vi "Multichannel Lockin--Develop.vi"() -> ()   [LabVIEW 2019, in "Instrument.Lockin.lvclass"]
uses:
  Instrument.Lockin/Instrument.Lockin.lvclass
  <vilib>/JKI/JKI SMO/SMO/Typedefs/SMOState --Enum.ctl
  Instrument.DAQ/Typedefs/Sweep.Channel--Cluster--Array.ctl
  Instrument.DAQ/Typedefs/Sweep.Channel--Cluster.ctl
  Instrument.DAQ/Typedefs/Sweep.Pattern--Enum.ctl
  Instrument.Lockin/Typedefs/Results Type--Enum.ctl
  <vilib>/Utility/error.llb/DialogType.ctl
  Instrument UI.Lockin/Instrument UI.Lockin.lvclass
  <vilib>/measure/NI_MAPro.lvlib
  <vilib>/Waveform/WDTOps.llb/WDT Waveform to XY Pairs DBL.vi
  <vilib>/Utility/config.llb/NI_LVConfig.lvlib
  <vilib>/JKI/JKI SMO/SMO/SMO.lvclass
  <userlib>/LevyLab/Instrument Framework/SMOs/RemoteControl/RemoteControl.lvclass
  <userlib>/LevyLab/Instrument Framework/SMOs/RemoteControl/Typedefs/Message--Cluster.ctl
  <userlib>/LevyLab/Instrument Framework/SMOs/RemoteControl/Typedefs/PrivateEvents--RemoteControl.Configure.ctl
  <userlib>/LevyLab/Instrument Framework/SMOs/Instrument/Instrument.lvclass
  Instrument.DAQ/Instrument.DAQ.lvclass
  <userlib>/LevyLab/Lockin-Multichannel/Lockin.DAQ/Typedefs/Set State-enum.ctl
  <vilib>/JKI/JKI SMO/SMO/Typedefs/Reserve State--Enum.ctl
  <vilib>/JKI/JKI SMO/SMO/Typedefs/Public Events.ctl
  <userlib>/LevyLab/Lockin-Multichannel/Lockin.DAQ/Typedefs/446xAO-enum.ctl
  <userlib>/LevyLab/Lockin-Multichannel/Lockin.DAQ/Typedefs/446xAI-enum.ctl
  Instrument.DAQ/Typedefs/DAQ.Config.AI.Coupling--enum.ctl
  Instrument.Lockin/Typedefs/Offset Mode--Enum.ctl
  Instrument.Lockin/Typedefs/API/Lockin.setAO_Amp--cluster.ctl
  Instrument.Lockin/Typedefs/API/Lockin.setAO_DC--cluster.ctl
  Instrument.Lockin/Typedefs/API/Lockin.setAO_f--cluster.ctl
  Instrument.Lockin/Typedefs/API/Lockin.setAO_phi--cluster.ctl
  Instrument.Lockin/Typedefs/API/Lockin.setAO_function--cluster.ctl
  Instrument.Lockin/Typedefs/API/Lockin.setAUX--cluster.ctl
  Instrument.Lockin/Typedefs/API/Lockin.setREF_f--cluster.ctl
  Instrument.Lockin/Typedefs/API/Lockin.setREF_phi--cluster.ctl
  Instrument.Lockin/Typedefs/REF Parameter--Enum.ctl
  Instrument.Lockin/Typedefs/API/Lockin.setREF_RollOff--cluster.ctl
  Instrument.Lockin/Typedefs/API/Lockin.setREF_TC--cluster.ctl
  db8adddc-ea00-4bba-81e3-073856fab83d.vi
  b40249d6-2344-4325-9322-c62ca3c32e30.vi
  4ac90d73-6816-45e1-9a9a-5cf5a9c18b14.vi
  7c039171-ebc7-488c-b96c-d45d5d49dc9d.vi
  615c5a2f-0bbc-45ac-9186-a3a982afc109.vi
  be3ecfbe-d453-46a9-a75a-8e102851b763.vi
  23a6cf49-6d38-4771-9ca1-822e649f0410.vi
  1f83e66f-7f6f-456b-9483-784a7ec7341a.vi
  8ae36af7-599d-4610-9c2c-7851f0fb9f0d.vi
  988d757e-36db-49af-af4d-8efcd29764ac.vi
  0dfb07b1-2a32-4a42-a1b7-b992f3b48bb1.vi
  90cbbb8a-83a7-4fa9-8dc2-325b52b36250.vi
  14a45371-8849-4e3a-b935-04e113710313.vi
  9e70ac36-a5eb-4546-996f-d1975d74bcd7.vi
  c2f37f8d-0579-483e-97a6-2ed33b24ebbd.vi
  aed423ae-cdb5-42aa-bd8f-e22cfa73b434.vi
  f9e94923-d644-4e5e-a3f3-1c5941609ee7.vi
  38ece5aa-da02-4231-8862-a988c08df37c.vi
  2d311ae9-1292-4ca0-8339-5bd3e0a854c1.vi
  37d717e0-1655-46e4-bb9c-9d30b95463df.vi
  3940afdf-3a76-4cdf-9013-99d5ad11d00a.vi
  5a0835ea-af00-4b0c-b4aa-accca3fcb3e4.vi
  95e32a6d-11f2-4e85-a49f-a0a7f7e69c5a.vi
  e3f2fa16-99b1-472f-9532-9ae1f83afe4f.vi
  <userlib>/LevyLab/Instrument Framework/SMOs/Logger.Error/Logger.Error.lvclass
  <vilib>/Utility/sysdir.llb/System Directory Type.ctl
  C:/Program Files (x86)/National Instruments/LabVIEW 2019/vi.lib/JKI/JKI SMO/SMO/SMO.lvclass
  Instrument.DAQ/Typedefs/AO.Channel.Function--Enum.ctl
  Instrument.DAQ/Typedefs/Sweep.Configuration--Cluster.ctl
  C:/Program Files (x86)/National Instruments/LabVIEW 2019/user.lib/LevyLab/Instrument Framework/SMOs/Instrument/Instrument.lvclass
  <userlib>/_OpenG.lib/error/error.llb/Filter Error Codes (Array)__ogtk.vi
  <vilib>/Waveform/WDTOps.llb/WDT Waveform Duration DBL.vi
  <vilib>/Platform/browser.llb/Open URL in Default Browser (string).vi
  <vilib>/measure/maspectr.llb/FFT Power Spectrum and PSD for N Chan.vi
panel:
  out "Results Plot Names":string[](array[string])
  out "Version":string="vDevelopment" caption="V"
  in  "Tab Control 4":T1(tab)
  in  "Disable all AI Ref":bool
  in  "Enable only AI Ref1":bool
  in  "Reset Phase":bool
  in  "AI Channels":T2(array[cluster]) {"References" items=["", "1"]}
  in  "AO freq link":dbl=13.0 format="%.3p"
  in  "AO Amp Limit":dbl=0.009999999 format="%.3p"
  in  "Limit Amplitudes":bool
  in  "Link Frequencies":bool
  in  "LP f (Hz)":dbl=100.0 format="%.3p"
  in  "Line":bool
  in  "Lowpass":bool
  in  "AO Channels":T3(array[cluster]) {"Phase" format="%.3g"; "Frequency" min=0.0001 max=10000.0 format="%.3g"; "Offset" format="%.3p"; "Amplitude" min=0.0 max=10.0 format="%.3p"}
  in  "REF Channels":T4(array[cluster]) {"Roll-Off" min=1; "TC" min=0.0001 format="%#_3p"; "Phase" format="%.3g"; "Frequency" min=0.0001 max=10000.0 format="%.3g"}
  in  "DAQ Config":T5(array[cluster]) {"AI.Coupling" items=["AC"=10045, "DC"=10050, "GND"=10066]}
  in  "auto DAQ":bool
  in  "Max Fs Refresh Rate (Hz)":dbl=10.0 format="%#_13g"
  in  "Sampling Mode":enum16{"Manual", "Auto Fs", "Max Fs"}(ring)
  in  "Sampling":cluster{"Fs":dbl, "#s":i32}={"Fs"=10000.0, "#s"=1000}
  in  "Auto x*F1":dbl=5000.0 format="%#_13g"
  in  "Load Configuration":bool
  in  "Save Configuration":bool
  in  "AI Simulation mode":T6(ring)=enum."AI = noise*AO"
  in  "decimating factor":i32=1
  in  "Remove":bool
  in  "Measure":bool
  in  "Stop Sweep":bool caption="Stop"
  in  "Sweep Time (s)":dbl=20.0 format="%#_1f"
  in  "Start Sweep":bool caption="Start"
  in  "Initial Wait (s)":dbl=1.0
  out "Sweep Timer (s)":dbl caption="Timer (s)"
  in  "Return to Start?":bool
  in  "Sweep Channels":T7 {"Channel" items=["AO1"=1, "AO2"=2]; "Start" format="%#_6p"; "End" format="%#_6p"}
  out "Sampling Status":string="Good"
  in  "Output Gain":cluster{"AI.Ch":string, "Gain":dbl}[](array[cluster])=[{"AI.Ch"="AO1", "Gain"=1.0}, {"AI.Ch"="AO2", "Gain"=1.0}, {"AI.Ch"="AO3", "Gain"=1.0}, {"AI.Ch"="AO4", "Gain"=1.0}, {"AI.Ch"="AO5", "Gain"=1.0}, {"AI.Ch"="AO6", "Gain"=1.0}, {"AI.Ch"="AO7", "Gain"=1.0}, {"AI.Ch"="AO8", "Gain"=1.0}, {"AI.Ch"="AO9", "Gain"=1.0}, {"AI.Ch"="AO10", "Gain"=1.0}, {"AI.Ch"="AO11", "Gain"=1.0}, {"AI.Ch"="AO12", "Gain"=1.0}, {"AI.Ch"="AO13", "Gain"=1.0}, {"AI.Ch"="AO14", "Gain"=1.0}, {"AI.Ch"="AO15", "Gain"=1.0}, {"AI.Ch"="AO16", "Gain"=1.0}]
  in  "Input Gain":cluster{"AI.Ch":string, "Gain":dbl}[](array[cluster])=[{"AI.Ch"="AI1", "Gain"=1.0}, {"AI.Ch"="AI2", "Gain"=1.0}, {"AI.Ch"="AI3", "Gain"=1.0}, {"AI.Ch"="AI4", "Gain"=1.0}, {"AI.Ch"="AI5", "Gain"=1.0}, {"AI.Ch"="AI6", "Gain"=1.0}, {"AI.Ch"="AI7", "Gain"=1.0}, {"AI.Ch"="AI8", "Gain"=1.0}, {"AI.Ch"="AI9", "Gain"=1.0}, {"AI.Ch"="AI10", "Gain"=1.0}, {"AI.Ch"="AI11", "Gain"=1.0}, {"AI.Ch"="AI12", "Gain"=1.0}, {"AI.Ch"="AI13", "Gain"=1.0}, {"AI.Ch"="AI14", "Gain"=1.0}, {"AI.Ch"="AI15", "Gain"=1.0}, {"AI.Ch"="AI16", "Gain"=1.0}]
  out "State History":string=" Exit\r Data: Cleanup\r Events: Unregister\r UI: Cleanup\r UI: Disable Buttons\r Configuration: Write\r Error Logger: Destroy\r Lockin SMO: Stop\r Remote SMO: Stop\r Macro: Exit\r UI: Update Sweep Timer\r UI: Update Lockin Graphs\r UI: Update Waveform Graphs\r 4461: OUT\r UI: Update Sweep Timer\r UI: Update Lockin Graphs\r UI: Update Waveform Graphs\r 4461: OUT\r UI: Update Sweep Timer\r UI: Update Lockin Graphs\r UI: Update Waveform Graphs\r 4461: OUT"
  out "Refresh time (ms)":u32=103
  out "LockinDAQ SMO State":T10=enum."Stopped" caption="SMO State"
  out "RC SMO State":T10=enum."Stopped" caption="SMO State"
  in  "Update":bool
  in  "Enable Output":bool caption="Enable"
  in  "Output Channel":i32=1 min=1
  out "Output (V)":dbl
  in  "Aux Channel":tag="Dev2/ao0"
  in  "Voltage Output (V)":dbl min=-50.0 max=50.0
  in  "Amplifier Gain":dbl=1.0 min=-15.0 max=15.0
  out "DAQ Output (V)":dbl=-0.0 min=-3.5 max=3.5
  out "Amplified Output (V)":dbl=-0.0 min=-3.5 max=3.5
  in  "AI Channel":i32=1
  in  "Reference Channel":i32=1
  in  "Type":T11
  in  "Allowed remote system":string
  in  "Get Calibration":bool
  out "Cal Info":T12(array[cluster]) {"SelfCal.LastDate/Time" format="%<%I:%M %p\n%m/%d/%Y>T"}
  in  "Self Calibrate":bool
  in  "Save":bool
  in  "Path":path=path "C:/Data/lockin"
  in  "Notes":string
  in  "Tab Control 3":enum32{"Page 1"}(tab)
  out "X":dbl=0.0014996100939563214 caption="X (V)" format="%#_3p"
  out "Y":dbl=-29.79492153733761 caption="Y (V)" format="%#_3p"
  in  "Channel":i32(ring)=1 items=["AI1 Ref1", "AI2 Ref1", "AI3 Ref1", "AI4 Ref1", "AI5 Ref1", "AI6 Ref1", "AI7 Ref1", "AI8 Ref1"]
  out "R":dbl=0.0014996100939563214 caption="R (V)" format="%#_3p"
  out "Theta":dbl=-29.79492153733761 caption="Theta (°)" format="%#_3p"
  in  "Display":enum16{"X and Y", "R and Theta", "Mean"}(ring)=enum."R and Theta" caption="Enum"
  in  "Close":bool
  out "Status":string="Shutdown"
  in  "Pause":bool
  in  "Reset":bool
  in  "Start":bool
  in  "Help":bool
  in  "Trigger":bool
  in  "Tab Control 2":T13(tab)
  in  "AI Graph All":bool
  in  "AI Graph None":bool
  in  "Y Axis (Output)":enum16{"Analog Output", "Reference"}(ring) caption="Enum 3"
  in  "Y Axis (Input)":enum16{"Device", "ADC"}(ring) caption="Enum 3"
  in  "Decimate":enum16{"1", "10", "100", "1000"}(ring) caption="Enum 3"
  in  "X Axis":enum16{"Time", "Samples"}(ring) caption="Enum 3"
  out "AI Graph":waveform(dbl)[](graph)
  out "AO Graph":waveform(dbl)[](graph)
  in  "AO Graph All":bool
  in  "AO Graph None":bool
  in  "Y/Theta Range":dbl caption="Axis Range" format="%#_6p"
  in  "X/R Range":dbl caption="Axis Range" format="%#_6p"
  out "Lockin 2":waveform(dbl)[](graph) caption="Lockin Display 2"
  out "Lockin 1":waveform(dbl)[](graph)
  in  "Lockin 1 None":bool
  in  "Lockin 1 All":bool
  out "Results":string[][](table)
  out "XY Graph":cluster{"Wavenumber":dbl[], "Data":dbl[]}[](graph)
  in  "XY Axis Range":dbl caption="Axis Range" format="%#_6p"
  out "Sweep Results Y":waveform(dbl)[](graph)
  out "Sweep Results X":waveform(dbl)[](graph)
  out "Sweep Results AI":waveform(dbl)[](graph)
  out "Sweep Results AO":waveform(dbl)[](graph)
  in  "# averages":u32=10 min=1
  in  "weighting mode":enum16{"Linear", "Exponential"}(ring)=enum."Exponential"
  in  "averaging mode":T14(ring)=enum."RMS averaging"
  in  "window":u16(ring) items=["Rectangle", "Hanning"]
  in  "export mode":u16(ring)=1 items=["Power Spectrum", "Power Spectral Density"]
  in  "restart":bool
  out "done?":bool=TRUE
  out "PS Chart":dbl[][](graph)
  out "PS WFGraph":cluster{"f0":dbl, "df":dbl, "magnitude":dbl[]}[](graph)
  out "averages":dbl=180.0
  # "Output"
  # "Input"
  # ">> DEVICE >>"
  # "Amp (V)"
  # "(*)"
  # "Ch"
  # "DC (V)"
  # "f (Hz)"
  # "Phase (°)"
  # "Function"
  # "Sweep"
  # "(*)"
  # "Ch"
  # "Ref1   2     3    4"
  # "Input: Pre-Filter"
  # "Output Settings"
  # "Reference"
  # "Reference Settings"
  # "Ch"
  # "f (Hz)"
  # "Phase (°)"
  # "TC (s)"
  # "Order"
  # "DAQ Channels"
  # "AI"
  # "Device"
  # "AO"
  # "Input: Offset"
  # "Ch"
  # "Range"
  # "Ch"
  # "Range"
  # "Coupling"
  # "Other Configuration"
  # "Sampling"
  # "Changing settings in this box will automatically\nreset the lockin and restart acquisition"
  # "Sweep"
  # "Channel"
  # "Start"
  # "End"
  # "Pattern"
  # "Status"
  # "Channel"
  # "Channel"
  # "Input Gain"
  # "Output Gain"
  # "Auxiliary Output"
  # "Configuration"
  # "- Use to control an auxiliiary card such as a multifunction DAQ (6115, 6120, etc)"
  # "Forward Lockin Input --> Lockin Output"
  # "- Choose an input lockin channel and value (X,Y, etc) and it will be written as a DC value to an output channel of your choosing.\n- Output is scaled by the input amplifier gain."
  # "Calibration"
  # "Self Cal\nLast Time"
  # "Self Cal\nLast Temp"
  # "Temp\nNow"
  # "Cal\nDue"
  # "Device"
  # "AI Graph"
  # "AO/Reference Graph"
  # "Lockin Results 1"
  # "Lockin Results 2"
  # "Lockin Results 2"
  # "Sweep Results"
  # "Sweep AO/AI"
  # "Power Spectra"
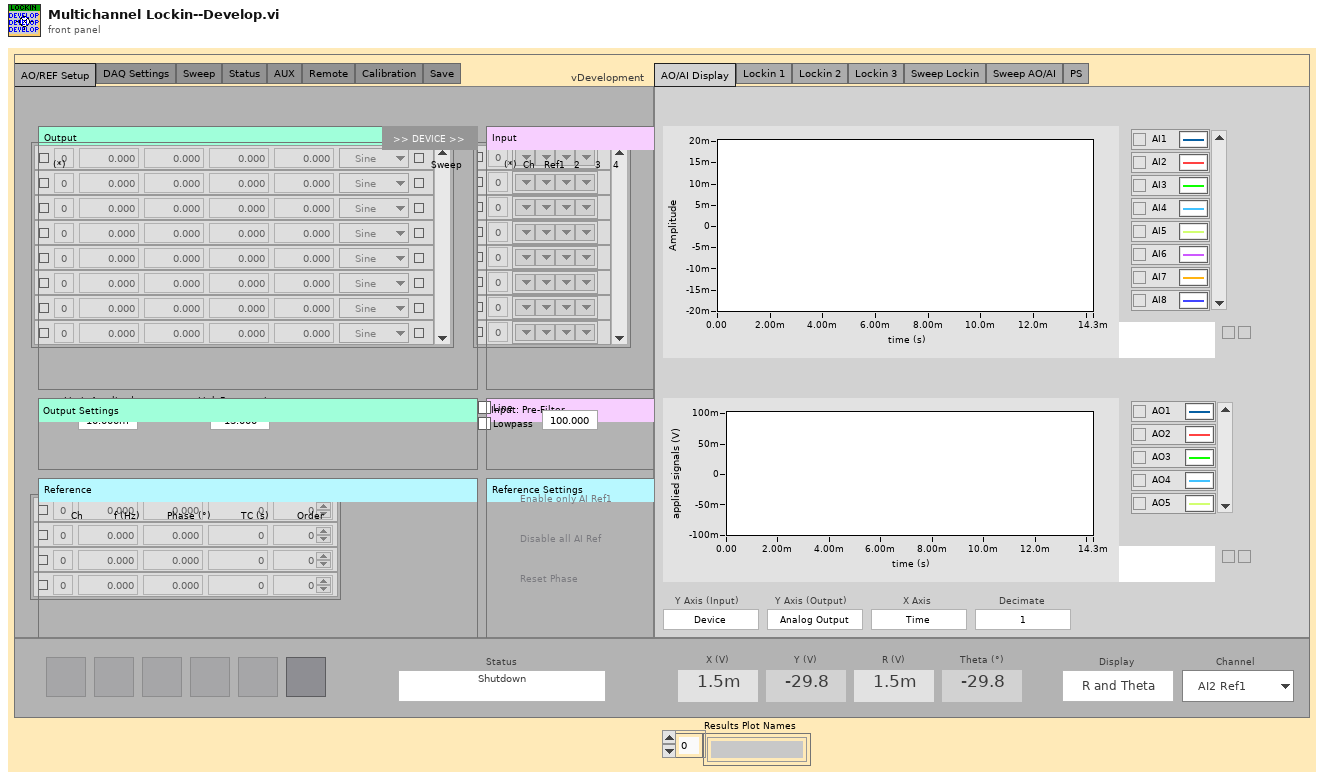
[diagram p1: front panel]
types:
  T1 = enum32{"AO/REF Setup", "DAQ Settings", "Sweep", "Status", "AUX", "Remote", "Calibration", "Save"}
  T2 = cluster{"Enable?":bool, "Channel":i32, "References":u16[]}[]
  T3 = cluster{"Enable?":bool, "Channel":i32, "Amplitude":dbl, "Offset":dbl, "Frequency":dbl, "Phase":dbl, "Function":enum16{"Sine", "Triangle", "Square"}, "Sweeping?":bool}[]
  T4 = cluster{"Enable?":bool, "Channel":i32, "Frequency":dbl, "Phase":dbl, "TC":dbl, "Roll-Off":i32}[]
  T5 = cluster{"Device":string, "AO.Ch":string, "AO.Range":enum16{"±0.1", "±1.0", "±10.0"}, "AI.Ch":string, "AI.Range":enum16{"±0.316", "±1.00", "±3.16", "±10.0", "±31.6", "±42.4"}, "AI.Coupling":u16}[]
  T6 = enum16{"AI = HW simulated", "AI = noise*AO", "AI = waveguide"}
  T7 = typedef "Instrument.DAQ.lvclass/Sweep.Channel--Cluster--Array.ctl" = T8[]
  T8 = typedef "Instrument.DAQ.lvclass/Sweep.Channel--Cluster.ctl" = cluster{"Enable?":bool, "Channel":u16, "Start":dbl, "End":dbl, "Pattern":T9}
  T9 = typedef "Instrument.DAQ.lvclass/Sweep.Pattern--Enum.ctl" = enum16{"Ramp /", "Ramp /\\", "Smooth Ramp _/", "Smooth Ramp _/\\_", "Frequency"}
  T10 = typedef "SMO.lvclass/SMOState --Enum.ctl" = enum16{"unknown", "Created", "Started", "Stopped"}
  T11 = typedef "Instrument.Lockin.lvclass/Results Type--Enum.ctl" = enum16{"X", "Y", "R", "Theta", "Mean"}
  T12 = cluster{"Active Device":string, "SelfCal.LastDate/Time":dbl, "SelfCal.LastTemp":dbl, "DevTemp":dbl, "calibration due?":bool}[]
  T13 = enum32{"AO/AI Display", "Lockin 1", "Lockin 2", "Lockin 3", "Sweep Lockin", "Sweep AO/AI", "PS"}
  T14 = enum16{"No averaging", "Vector averaging", "RMS averaging", "Peak hold"}
  T15 = enum16{"start", "stop", "reset", "start sweep", "stop sweep"}
  T16 = typedef "Lockin.DAQ.lvclass/Set State-enum.ctl" = enum16{"start", "stop", "reset", "start sweep", "stop sweep"}
  T17 = typedef "Instrument.DAQ.lvclass/Sweep.Configuration--Cluster.ctl" = cluster{"Sweep Time (s)":dbl, "Initial Wait (s)":dbl, "Return to Start":bool, "Channels":T7}
  T18 = enum32{"invalid app kind", "Development System", "Run Time System", "Student Edition", "Embedded LabVIEW", "Evaluation", "Custom"}
  T19 = enum32{"Invalid", "Standard", "Closed", "Hidden", "Minimized", "Maximized"}
  T20 = enum8{"Enabled", "Disabled", "Disabled and Grayed Out"}
  T21 = typedef "Instrument.Lockin.lvclass/Lockin.setAO_Amp--cluster.ctl" = cluster{"AO Channel":i32, "Amplitude (V)":dbl}
  T22 = enum16{"Amplitude", "DC", "Frequency", "Phase", "Function"}
  T23 = typedef "Instrument.Lockin.lvclass/Lockin.setAO_DC--cluster.ctl" = cluster{"AO Channel":i32, "DC (V)":dbl}
  T24 = typedef "Instrument.Lockin.lvclass/Lockin.setAO_f--cluster.ctl" = cluster{"AO Channel":i32, "Frequency (Hz)":dbl}
  T25 = typedef "Instrument.Lockin.lvclass/Lockin.setAO_phi--cluster.ctl" = cluster{"AO Channel":i32, "Phase (°)":dbl}
  T26 = typedef "Instrument.Lockin.lvclass/Lockin.setAO_function--cluster.ctl" = cluster{"AO Channel":i32, "Function":T27}
  T27 = typedef "Instrument.DAQ.lvclass/AO.Channel.Function--Enum.ctl" = enum16{"Sine", "Triangle", "Square"}
  T28 = typedef "Instrument.Lockin.lvclass/REF Parameter--Enum.ctl" = enum16{"Frequency", "Phase", "Time Constant", "RollOff"}
  T29 = typedef "Instrument.Lockin.lvclass/Lockin.setREF_f--cluster.ctl" = cluster{"REF Channel":i32, "Frequency (Hz)":dbl}
  T30 = typedef "Instrument.Lockin.lvclass/Lockin.setREF_phi--cluster.ctl" = cluster{"REF Channel":i32, "Phase (°)":dbl}
  T31 = typedef "Instrument.Lockin.lvclass/Lockin.setREF_TC--cluster.ctl" = cluster{"REF Channel":i32, "TC (s)":dbl}
  T32 = typedef "Instrument.Lockin.lvclass/Lockin.setREF_RollOff--cluster.ctl" = cluster{"REF Channel":i32, "Roll-Off":i32}
  T33 = typedef "Instrument.Lockin.lvclass/Offset Mode--Enum.ctl" = enum16{"Measure", "Remove"}
  T34 = cluster{"averaging mode":enum16{"No averaging", "Vector averaging", "RMS averaging", "Peak hold"}, "weighting mode":enum16{"Linear", "Exponential"}, "number of averages":u32}
  T35 = typedef "Instrument.Lockin.lvclass/Lockin.setAUX--cluster.ctl" = cluster{"AO Channel":i32, "AUX (V)":dbl}
  T36 = typedef "Lockin.DAQ.lvclass/446xAO-enum.ctl" = enum16{"±0.1", "±1.0", "±10.0"}
  T37 = typedef "Lockin.DAQ.lvclass/446xAI-enum.ctl" = enum16{"±0.316", "±1.00", "±3.16", "±10.0", "±31.6", "±42.4"}
  T38 = typedef "Instrument.DAQ.lvclass/DAQ.Config.AI.Coupling--enum.ctl" = u16
  T39 = cluster{"Device":string, "AO.Ch":string, "AO.Range":T36, "AI.Ch":string, "AI.Range":T37, "AI.Coupling":T38}[]
  T40 = typedef "Instrument.DAQ.lvclass/Channel.Gain--Cluster--Array.ctl" = T41[]
  T41 = typedef "Instrument.DAQ.lvclass/Channel.Gain--Cluster.ctl" = cluster{"Channel":string, "Gain":dbl}
  T42 = typedef "RemoteControl.lvclass/PrivateEvents--RemoteControl.Configure.ctl" = cluster{"address":string, "Port":u16, "AllowedRemote":string, "Commands":string[], "timeout":i32}
  T43 = typedef "RemoteControl.lvclass/Message--Cluster.ctl" = cluster{"Command":string, "Data":variant, "ID":string}
  T44 = cluster{"Core":cluster{"Current VI Reference":refnum<vi>, "Close Panel on Exit?":bool}, "to":i32, "Lockin":refnum<class "Instrument.Lockin.lvclass">, "RemoteControl":refnum<class "RemoteControl.lvclass">, "Lockin.DAQ":refnum<class "Instrument.DAQ.lvclass">, "Logger.Error":refnum<class "Logger.Error.lvclass">, "DAQ state":enum16{"idle", "created", "started", "stopped", "sweeping"}, "RemoteControl.Configure":T42, "Message":T43, "HandledMessage":T43, "SweepResults":cluster{"X results":waveform(dbl)[], "Y Results":waveform(dbl)[]}, "SweepWaveforms":cluster{"Sweep_AO":waveform(dbl)[], "Sweep_AI":waveform(dbl)[]}}
  T45 = enum16{"idle", "created", "started", "stopped", "sweeping"}
  T46 = typedef "Instrument.DAQ.lvclass/DAQ.Config.AO--Cluster--Array.ctl" = T47[]
  T47 = typedef "Instrument.DAQ.lvclass/DAQ.Config.AO--Cluster.ctl" = cluster{"Channels":tag, "Range":T48, "output terminal configuration":i32, "Type":T49}
  T48 = typedef "Instrument.DAQ.lvclass/DAQ.Config.AO.Range--enum.ctl" = enum16{"±0.1", "±1.0", "±10.0"}
  T49 = typedef "Instrument.DAQ.lvclass/DAQ.Type--enum.ctl" = enum16{"None", "USB 4431", "PXI 446x"}
  T50 = typedef "Instrument.DAQ.lvclass/DAQ.Config.AI--Cluster--Array.ctl" = T51[]
  T51 = typedef "Instrument.DAQ.lvclass/DAQ.Config.AI--Cluster.ctl" = cluster{"Channels":tag, "Coupling":T38, "Range":T52, "input terminal configuration":i32, "Type":T49}
  T52 = typedef "Instrument.DAQ.lvclass/DAQ.Config.AI.Range--enum.ctl" = enum16{"±0.316", "±1.00", "±3.16", "±10.0", "±31.6", "±42.4"}
  T53 = typedef "Lockin.DAQ.lvclass/Results--Cluster.ctl" = cluster{"Time Stamp":timestamp, "Results (Dictionary)":cluster{"key":string, "value":dbl}[]}
  T54 = typedef "Lockin.DAQ.lvclass/AO-cluster.ctl" = T55[]
  T55 = typedef "Instrument.Lockin.UI.lvclass/AO Channel--Cluster.ctl" = cluster{"Enable?":bool, "Channel":i32, "Amplitude":dbl, "Offset":dbl, "Frequency":dbl, "Phase":dbl, "Function":T56, "Sweeping?":bool}
  T56 = typedef "Lockin.DAQ.lvclass/Function-enum.ctl" = enum16{"Sine", "Triangle", "Square"}
  T57 = typedef "Lockin.DAQ.lvclass/REF-cluster.ctl" = T58[]
  T58 = typedef "Instrument.Lockin.UI.lvclass/REF Channel--Cluster.ctl" = cluster{"Enable?":bool, "Channel":i32, "Frequency":dbl, "Phase":dbl, "TC":dbl, "Roll-Off":i32}
  T59 = typedef "Lockin.DAQ.lvclass/PublicEvents--Lockin.DAQ.getDAQconfig.ctl" = T60[]
  T60 = typedef "Instrument.Lockin.UI.lvclass/Device Configuration--Cluster.ctl" = cluster{"Device":string, "AO.Ch":string, "AO.Range":T36, "AI.Ch":string, "AI.Range":T37, "AI.Coupling":T61}
  T61 = typedef "Lockin.DAQ.lvclass/AI.coupling-enum.ctl" = u16
  T62 = typedef "Lockin.DAQ.lvclass/PublicEvents--Lockin.DAQ.getCalibration.ctl" = T63[]
  T63 = typedef "Lockin.DAQ.lvclass/Cal Info - Cluster.ctl" = cluster{"Active Device":string, "SelfCal.LastDate/Time":dbl, "SelfCal.LastTemp":dbl, "DevTemp":dbl, "calibration due?":bool}
  T64 = typedef "Lockin.DAQ.lvclass/SweepResults--Cluster.ctl" = cluster{"X results":waveform(dbl)[], "Y Results":waveform(dbl)[]}
  T65 = cluster{"X":waveform(dbl)[], "Y":waveform(dbl)[]}
  T66 = typedef "Lockin.DAQ.lvclass/PublicEvents--Lockin.DAQ.getAI.ctl" = waveform(dbl)[]
  T67 = typedef "Lockin.DAQ.lvclass/PublicEvents--Lockin.DAQ.getAO.ctl" = waveform(dbl)[]
  T68 = typedef "Lockin.DAQ.lvclass/State-enum.ctl" = enum16{"idle", "created", "started", "stopped", "sweeping"}
  T69 = typedef "DialogType.ctl" = u16
  T70 = cluster{"Sweep_AO":waveform(dbl)[], "Sweep_AI":waveform(dbl)[]}
  T71 = cluster{"X results":waveform(dbl)[], "Y Results":waveform(dbl)[]}
  T72 = cluster{"Time Stamp":timestamp, "Results (Dictionary)":cluster{"key":string, "value":dbl}[]}
  T73 = cluster{"Current VI Reference":refnum<vi>, "Close Panel on Exit?":bool}
  T74 = typedef "SMO.lvclass/Public Events.ctl" = cluster{"Error":refnum<user-event>, "State":refnum<user-event>, "Reserve State":refnum<user-event>}
  T75 = typedef "RemoteControl.lvclass/PublicEvents--Cluster.ctl" = cluster{"SendMessageFromProcess":refnum<user-event>}
  T76 = typedef "Lockin.DAQ.lvclass/PublicEvents--Cluster.ctl" = cluster{"getAO":refnum<user-event>, "getAI":refnum<user-event>, "getREF":refnum<user-event>, "getResults":refnum<user-event>, "getCalibration":refnum<user-event>, "getAOChannels":refnum<user-event>, "getREFChannels":refnum<user-event>, "getDAQState":refnum<user-event>, "getSweepResults":refnum<user-event>, "getSweepWaveforms":refnum<user-event>, "getDAQconfig":refnum<user-event>}
  T77 = typedef "Instrument.DAQ.lvclass/AI.Channel--Cluster--Array.ctl" = T78[]
  T78 = typedef "Instrument.DAQ.lvclass/AI.Channel--Cluster.ctl" = cluster{"Enable?":bool, "Channel":i32, "References":i32[]}
  T79 = typedef "System Directory Type.ctl" = i32
  T80 = typedef "RemoteControl.lvclass/RC Com Type--enum.ctl" = enum16{"RC", "STM", "ZMQ"}
  T81 = typedef "Instrument.DAQ.lvclass/AO.Channel--Cluster--Array.ctl" = T82[]
  T82 = typedef "Instrument.DAQ.lvclass/AO.Channel--Cluster.ctl" = cluster{"Enable?":bool, "Channel":i32, "Amplitude":dbl, "Offset":dbl, "Frequency":dbl, "Phase":dbl, "Function":T27, "Sweeping?":bool}
  T83 = typedef "Instrument.DAQ.lvclass/REF.Channel--Cluster--Array.ctl" = T84[]
  T84 = typedef "Instrument.DAQ.lvclass/REF.Channel--Cluster.ctl" = cluster{"Enable?":bool, "Channel":i32, "Frequency":dbl, "Phase":dbl, "TC":dbl, "Roll-Off":i32}
  T85 = typedef "Instrument.DAQ.lvclass/Configuration.Prefilter--Cluster.ctl" = cluster{"60 Hz":bool, "Low Pass":bool, "Low Pass Cutoff (Hz)":dbl}
  T86 = typedef "Instrument.Lockin.lvclass/Lockin.Configuration--Cluster.ctl" = cluster{"AO Channels":T54, "REF Channels":T57, "AI Channels":T87, "REF Filter":T89, "Amplifers":cluster{"offsets":dbl[], "Input Gain":dbl[], "Output Gain":dbl[], "Amplifiers":T90}, "DAQ":cluster{"sampling":T91, "sample mode":i32, "buffer size (S)":u32, "decimation":u32}, "Calibration":cluster{"Cal Info":T63[]}, "AI Configuration":T92, "AO Configuration":T95, "Aux Channel":tag, "Simulation mode":T97}
  T87 = typedef "Lockin.DAQ.lvclass/AI-cluster.ctl" = T88[]
  T88 = typedef "Instrument.Lockin.UI.lvclass/AI Channel--Cluster.ctl" = cluster{"Enable?":bool, "Channel":i32, "References":u16[]}
  T89 = typedef "Lockin.DAQ.lvclass/AI Prefilter-cluster.ctl" = cluster{"60 Hz prefilter":bool, "LP prefilter":bool, "LP cutoff (Hz)":dbl}
  T90 = typedef "Lockin.DAQ.lvclass/AmplifierType-enum.ctl" = enum16{"Manual", "Krohn Hite", "Femto"}
  T91 = typedef "Lockin.DAQ.lvclass/Sampling.ctl" = cluster{"Fs":dbl, "#s":i32}
  T92 = typedef "Lockin.DAQ.lvclass/AI.config-array.ctl" = T93[]
  T93 = typedef "Lockin.DAQ.lvclass/AI.config-cluster.ctl" = cluster{"AI.channels":tag, "AI.Coupling":T61, "AI.Range":T37, "input terminal configuration":i32, "DAQ Type":T94}
  T94 = typedef "Lockin.DAQ.lvclass/DAQType-enum.ctl" = enum16{"None", "USB 4431", "PXI 446x"}
  T95 = typedef "Lockin.DAQ.lvclass/AO.config-array.ctl" = T96[]
  T96 = typedef "Lockin.DAQ.lvclass/AO.config-cluster.ctl" = cluster{"AO.channels":tag, "AO.Range":T36, "output terminal configuration":i32, "DAQ Type":T94}
  T97 = typedef "Lockin.DAQ.lvclass/AI Simulation-enum.ctl" = enum16{"AI = HW simulated", "AI = noise*AO", "AI = waveguide"}
  T98 = typedef "Instrument.DAQ.lvclass/DAQ.Configuration--Cluster.ctl" = cluster{"Device":string, "AO.Ch":string, "AO.Range":T48, "AI.Ch":string, "AI.Range":T52, "AI.Coupling":T38}
  T99 = typedef "Instrument.DAQ.lvclass/DAQ.Sampling--Cluster.ctl" = cluster{"Sampling":T100, "Sample Mode":T101, "Fs Mode":T102, "Fs Multiplier":dbl, "Refresh Rate (Hz)":dbl, "Decimation":i32}
  T100 = typedef "Instrument.DAQ.lvclass/DAQ.Sampling.Sampling--Cluster.ctl" = cluster{"Fs":dbl, "#s":i32}
  T101 = typedef "Instrument.DAQ.lvclass/DAQ.Sampling.Sample Mode--Ring.ctl" = i32
  T102 = typedef "Instrument.DAQ.lvclass/DAQ.Sampling.Fs Mode--enum.ctl" = enum16{"Manual", "Auto Fs", "Max Fs"}
  T103 = cluster{"Sweep Time (s)":dbl, "Initial Wait (s)":dbl, "Return to Start":bool, "Channels":T8[]}
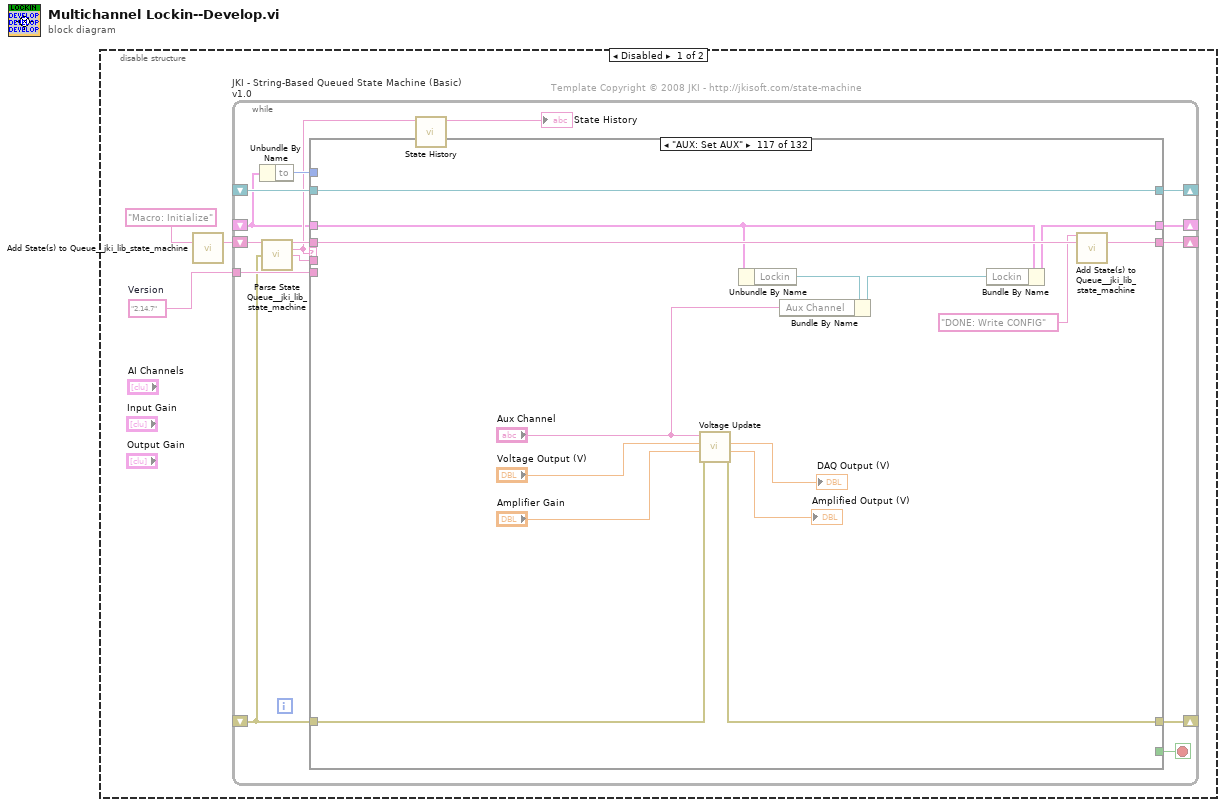
[diagram p0: block diagram]
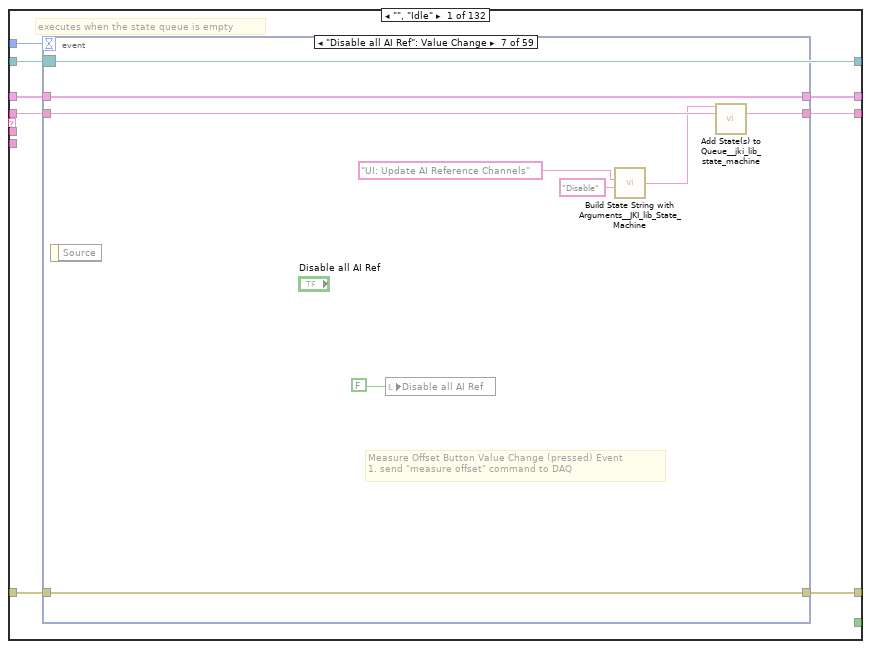
[diagram p2: hidden frame]
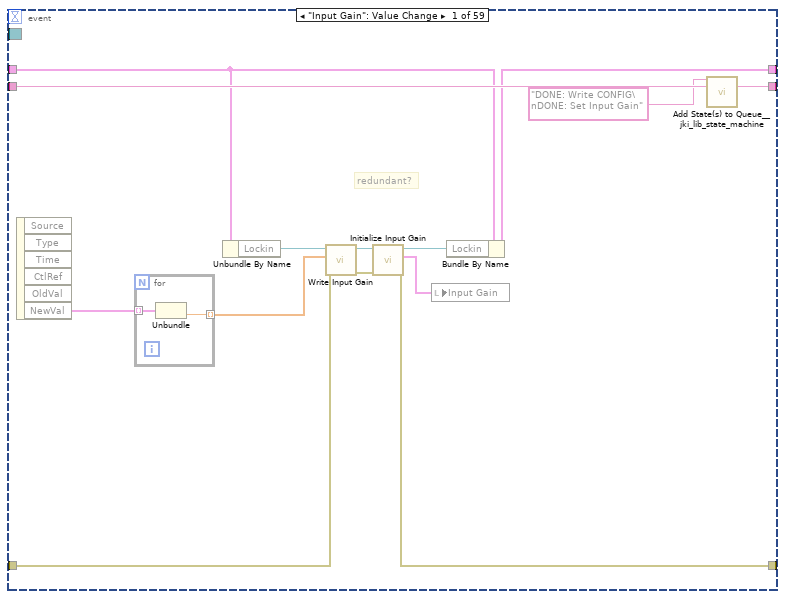
[diagram p3: hidden frame]
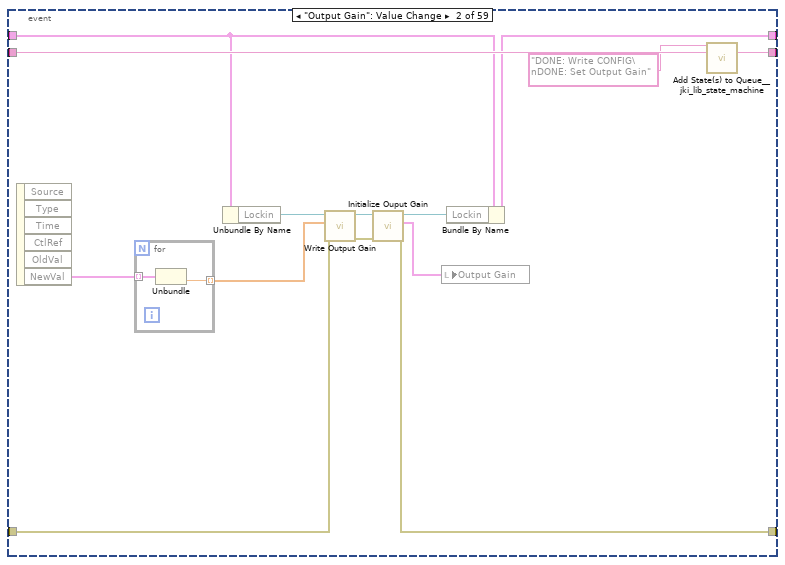
[diagram p4: hidden frame]
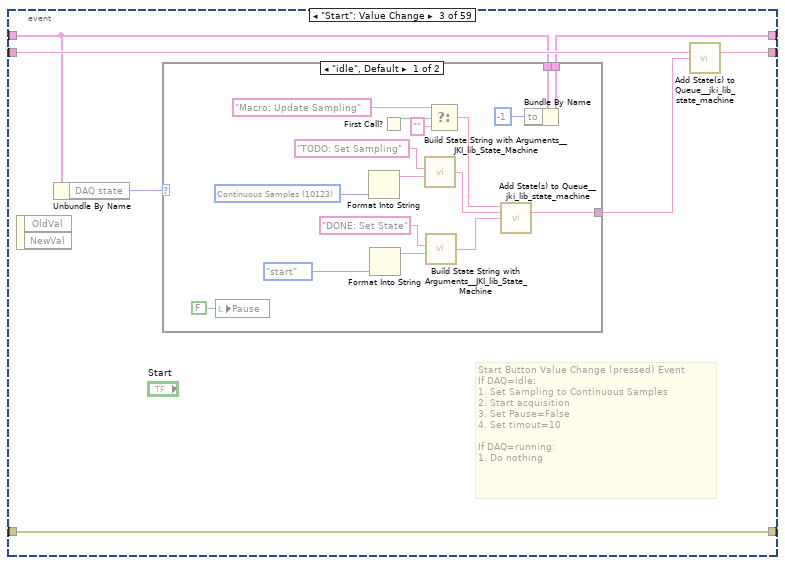
[diagram p5: hidden frame]
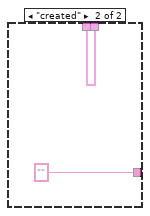
[diagram p6: hidden frame]
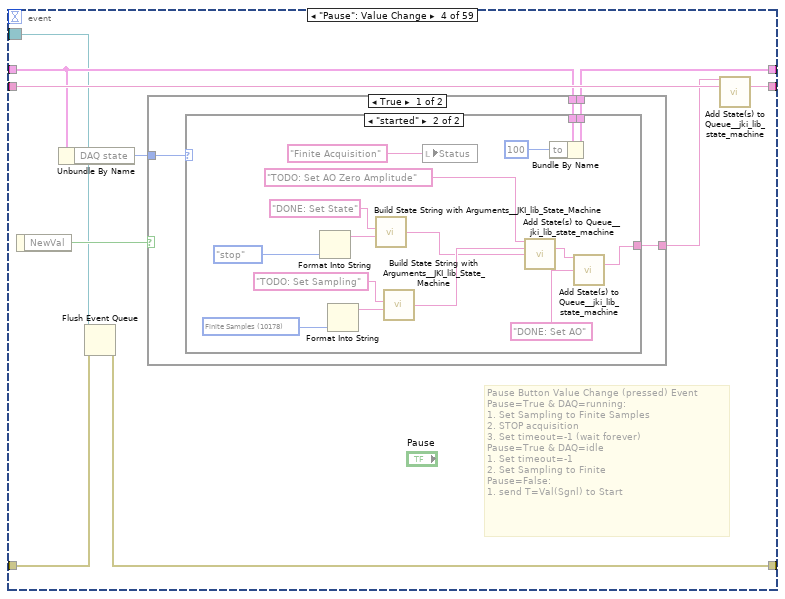
[diagram p7: hidden frame]
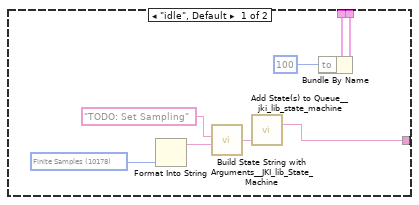
[diagram p8: hidden frame]
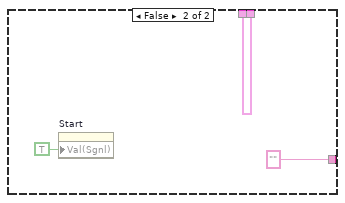
[diagram p9: hidden frame]
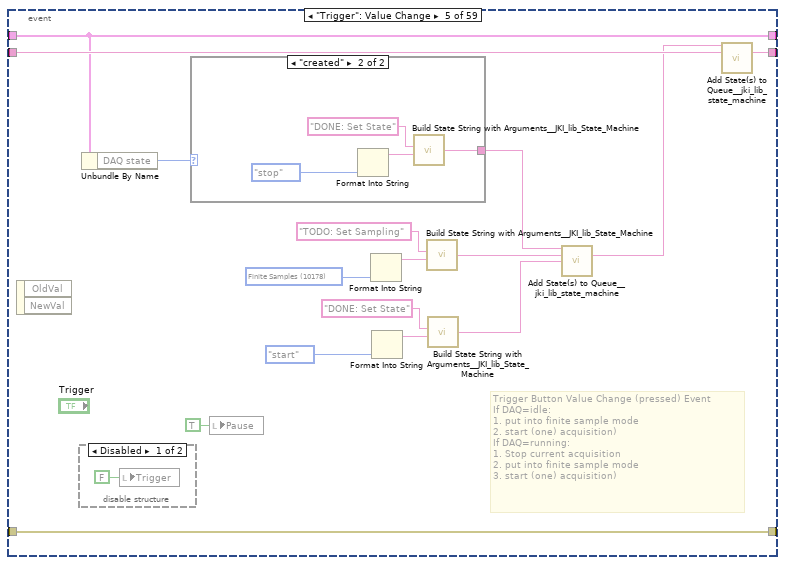
[diagram p10: hidden frame]
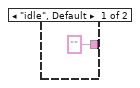
[diagram p12: hidden frame]
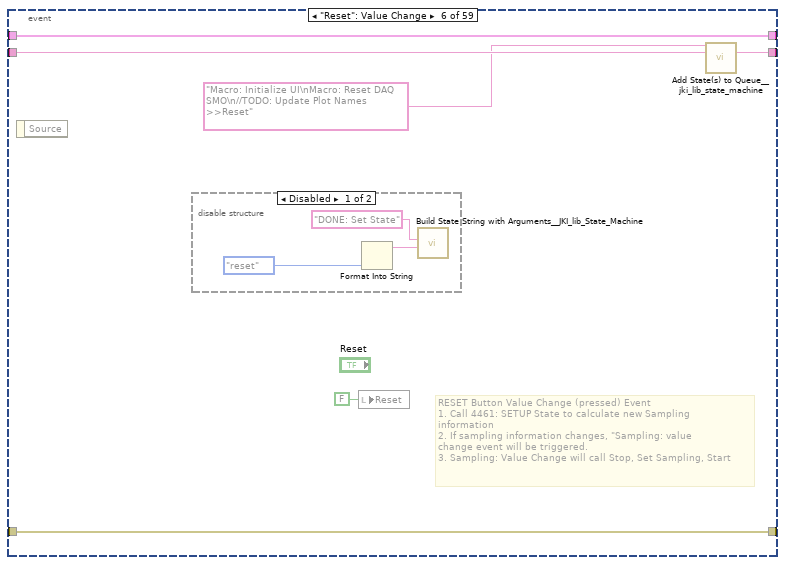
[diagram p13: hidden frame]
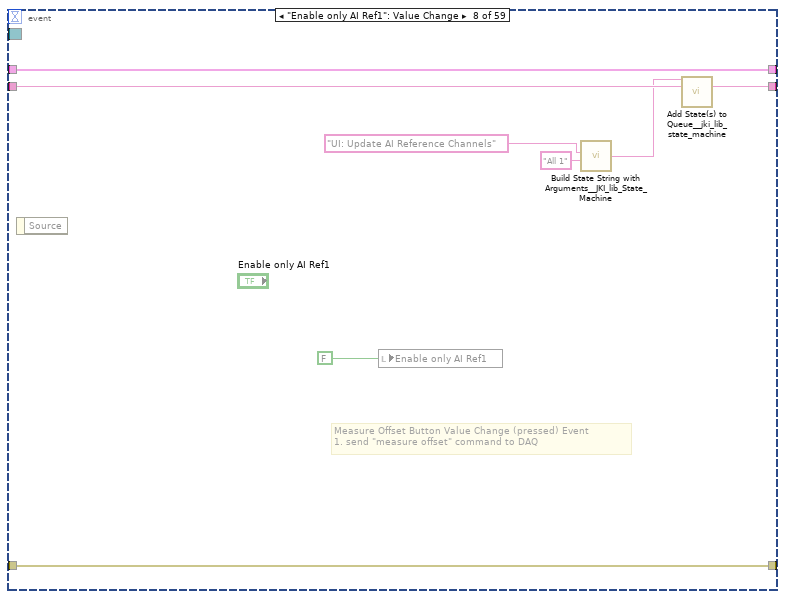
[diagram p15: hidden frame]
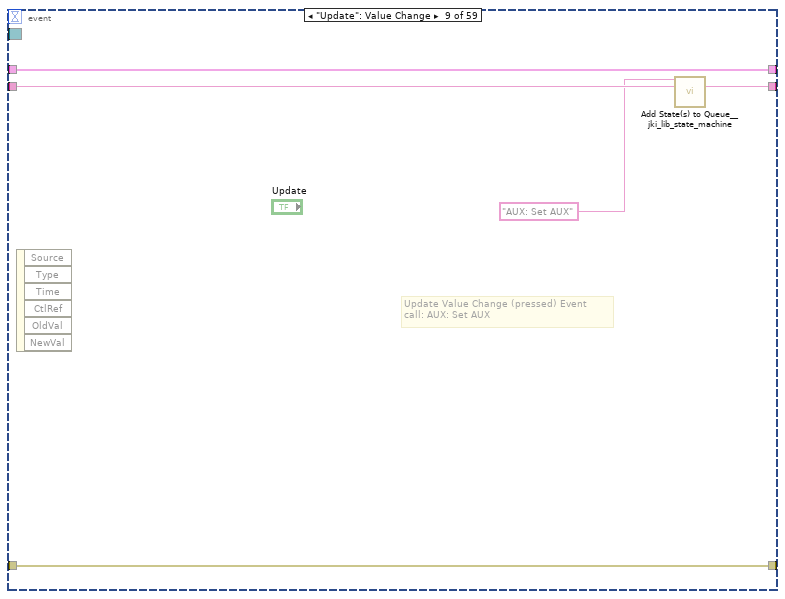
[diagram p16: hidden frame]
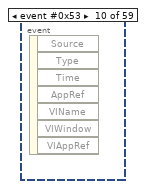
[diagram p17: hidden frame]
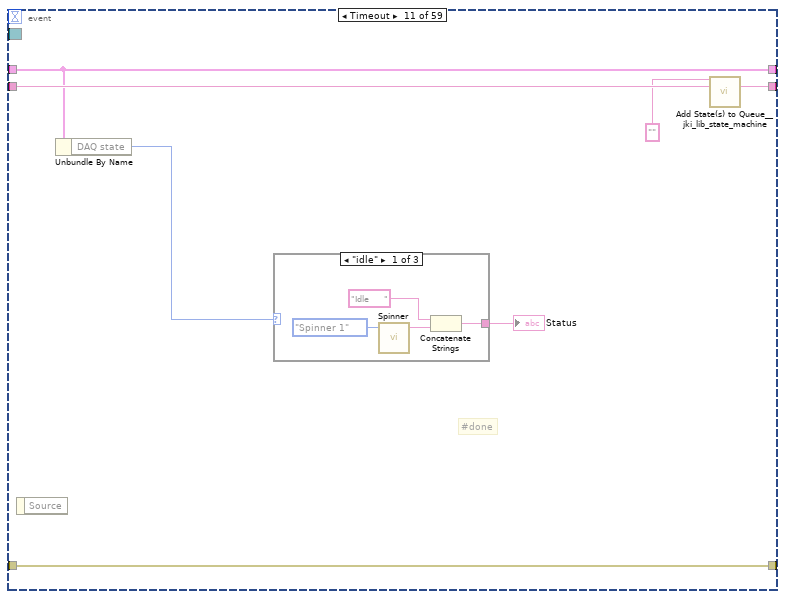
[diagram p18: hidden frame]
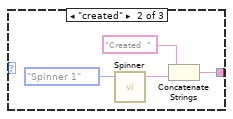
[diagram p19: hidden frame]
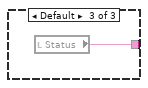
[diagram p20: hidden frame]
diagram:
  n1 = disable-structure shown="Disabled" {
    frame Disabled {
      w1 = "2.14.7"  # Version
      # "Template Copyright © 2008 JKI - http://jkisoft.com/state-machine"
      n2 = call <vilib>:"Add State(s) to Queue__jki_lib_state_machine.vi"("State(s) in (\"\")"="Macro: Initialize") -> ("States Out"=w3:string)  [unwired: 14 in]
      n3 = while "JKI - String-Based Queued State Machine (Basic) v1.0" {
        shift-right: [w10] -> _
        shift-left: _ -> [w4]
        shift-right: [w7] -> _
        shift-left: _ -> [w5]
        shift-right: [w17] -> _
        shift-left: w3 -> [w14]
        shift-right: [w11] -> _
        shift-left: _ -> [w12]
        tunnel: w1 -> [w6]
        stop <- w16 stop-if-true
        n4 = Unbundle By Name(w4) -> ("to"=w13:i32)
        n5 = call <vilib>:"Parse State Queue__jki_lib_state_machine.vi"("State Queue"=w14, "Error In (no error)"=w5) -> ("Remaining States"=w15:string, "Current State"=w8:string, "Arguments"=w18:string)  [unwired: 11 in]
        n6 = case shown="\"AUX: Set AUX\"" w8 {
          selector: w8 -> [_ _ w614 _ _ _ _ _ _ _ _ _ _ _ _ _ _ _ _ _ _ _ _ _ _ _ _ _ _ _ _ _ _ _ _ _ _ _ _ _ _ _ _ _ _ _ _ _ _ _ _ _ _ _ _ _ _ _ _ _ _ _ _ _ _ _ _ _ _ _ _ _ _ _ _ _ _ _ _ _ _ _ _ _ _ _ _ _ _ _ _ _ _ _ _ _ _ _ _ _ _ _ _ _ _ _ _ _ _ _ _ _ _ _ _ _ _ _ _ _ _ _ _ _ _ _ _ _ _ _ _ _]
          tunnel: w18 -> [_ _ _ _ _ _ _ _ _ _ _ _ _ _ _ _ _ _ _ _ w842 _ _ _ _ _ _ _ _ _ w1006 w1019 w1029 _ _ _ w1139 _ _ _ w1227 w1239 _ _ _ _ _ _ _ _ _ _ _ _ _ _ _ _ w1536 _ _ _ _ _ _ _ _ w1627 _ _ _ _ _ _ _ _ _ _ _ _ _ _ _ _ _ _ _ _ _ _ _ _ _ _ _ _ _ _ _ _ _ _ _ _ _ _ _ _ _ _ _ w2202 w2245 _ _ _ _ _ _ _ _ _ _ _ _ _ _ _ _ _ _ _]
          tunnel: [w25 w610 w617 w635 w648 w660 w665 w682 w689 w694 w719 w725 w730 w737 w742 w750 w776 w813 w835 w840 w853 w873 w888 w901 w906 w919 w940 w965 w972 w994 w1011 w1020 w1032 w1061 w1068 w1081 w1142 w1165 w1173 w1210 w1230 w1243 w1256 w1269 w1284 w1313 w1324 w1335 w1351 w1380 w1389 w1411 w1449 w1467 w1476 w1485 w1507 w1526 w1542 w1562 w1571 w1580 w1589 w1598 w1607 w1616 w1625 w1634 w1643 w1651 w1659 w1667 w1679 w1701 w1710 w1727 w1755 w1761 w1767 w1773 w1779 w1785 w1791 w1797 w1803 w1809 w1815 w1820 w1829 w1839 w1849 w1859 w1869 w1879 w1889 w1899 w1921 w1943 w1965 w1987 w2009 w2031 w2053 w2075 w2097 w2111 w2123 w2140 w2165 w2170 w2187 w2210 w2252 w2259 w2268 w2309 w2328 w2333 w2349 w2364 w2380 w2396 w2411 w2427 w2445 w2460 w2475 w2494 w2517 w2536 w2550 w2565] -> w17
          tunnel: [_ _ _ _ _ TRUE _ _ _ _ _ _ _ _ _ _ _ _ _ _ _ _ _ _ _ _ _ _ _ _ _ _ _ _ _ _ _ _ _ _ _ _ _ _ _ _ _ _ _ _ _ _ _ _ _ _ _ _ _ _ _ _ _ _ _ _ _ _ _ _ _ _ _ _ _ _ _ _ _ _ _ _ _ _ _ _ _ _ _ _ _ _ _ _ _ _ _ _ _ _ _ _ _ _ _ _ _ _ _ _ _ _ _ _ _ _ _ _ _ _ _ _ _ _ _ _ _ _ _ _ _ _] -> w16
          tunnel: w13 -> [w20 _ _ _ _ _ _ _ _ _ _ _ _ _ _ _ _ _ _ _ _ _ _ _ _ _ _ _ _ _ _ _ _ _ _ _ _ _ _ _ _ _ _ _ _ _ _ _ _ _ _ _ _ _ _ _ _ _ _ _ _ _ _ _ _ _ _ _ _ _ _ _ _ _ _ _ _ _ _ _ _ _ _ _ _ _ _ _ _ _ _ _ _ _ _ _ _ _ _ _ _ _ _ _ _ _ _ _ _ _ _ _ _ _ _ _ _ _ _ _ _ _ _ _ _ _ _ _ _ _ _ _]
          tunnel: w15 -> [w26 w611 w618 w636 w649 w661 w666 w683 w690 w695 w720 w726 w731 w732 w743 w751 w777 w814 w836 w841 w854 w874 w889 w902 w907 w920 w941 w966 w973 w995 w1012 w1021 w1033 w1062 w1069 w1082 w1143 w1166 w1174 w1211 w1231 w1244 w1257 w1270 w1285 w1314 w1325 w1336 w1352 w1381 w1390 w1412 w1450 w1468 w1477 w1486 w1508 w1527 w1543 w1563 w1572 w1581 w1590 w1599 w1608 w1617 w1626 w1635 w1644 w1652 w1660 w1668 w1680 w1702 w1709 w1726 w1756 w1762 w1768 w1774 w1780 w1786 w1792 w1798 w1804 w1810 w1816 w1821 w1830 w1840 w1850 w1860 w1870 w1880 w1890 w1900 w1922 w1944 w1966 w1988 w2010 w2032 w2054 w2076 w2098 w2112 w2124 w2127 w2166 w2171 w2188 w2211 w2253 w2260 w2267 w2305 w2329 w2334 w2350 w2365 w2381 w2397 w2412 w2428 w2446 w2461 w2476 w2495 w2518 w2537 w2551 w2566]
          tunnel: w12 -> [w19 w608 w613 w624 w644 w657 w663 w680 w688 w692 _ w722 w727 w735 w739 w749 w775 w811 w828 w837 w852 w872 w887 w899 w903 w917 w939 w962 w970 w991 w1009 w1017 w1026 w1059 w1066 w1079 w1140 w1164 w1170 w1209 w1228 w1241 w1253 w1266 w1283 w1312 w1323 w1334 w1349 w1379 w1388 w1405 w1444 w1466 w1475 w1481 w1502 w1522 w1541 w1561 w1570 w1579 w1588 w1597 w1606 w1615 w1624 w1633 w1642 w1650 w1658 w1666 w1670 w1700 w1708 w1725 w1754 w1760 w1766 w1772 w1778 w1784 w1790 w1796 w1802 w1808 w1814 w1817 w1828 w1838 w1848 w1858 w1868 w1878 w1888 w1898 w1920 w1942 w1964 w1986 w2008 w2030 w2052 w2074 w2096 w2110 w2122 w2132 w2162 w2167 w2186 w2209 w2251 w2256 w2266 w2306 w2327 w2330 w2348 w2363 w2379 w2395 w2410 w2426 w2444 w2459 w2474 w2493 w2516 w2535 w2549 w2564]
          tunnel: [w19 w608 w613 w624 w644 w657 w663 w680 w688 w692 w718 w722 w727 w735 w739 w749 w775 w811 w828 w837 w852 w872 w887 w899 w903 w917 w939 w962 w970 w991 w1009 w1017 w1026 w1059 w1066 w1079 w1140 w1164 w1170 w1209 w1228 w1241 w1253 w1266 w1283 w1312 w1323 w1334 w1349 w1379 w1388 w1405 w1444 w1466 w1475 w1481 w1502 w1522 w1541 w1561 w1570 w1579 w1588 w1597 w1606 w1615 w1624 w1633 w1642 w1650 w1658 w1666 w1670 w1700 w1708 w1725 w1754 w1760 w1766 w1772 w1778 w1784 w1790 w1796 w1802 w1808 w1814 w1817 w1828 w1838 w1848 w1858 w1868 w1878 w1888 w1898 w1920 w1942 w1964 w1986 w2008 w2030 w2052 w2074 w2096 w2110 w2122 w2132 w2162 w2167 w2186 w2209 w2251 w2256 w2266 w2306 w2327 w2330 w2348 w2363 w2379 w2395 w2410 w2426 w2444 w2459 w2474 w2493 w2516 w2535 w2549 w2564] -> w11
          tunnel: [w22 w607 w616 w634 w641 w656 w662 w676 w685 w691 w717 w724 w728 w733 w740 w745 w771 w798 w829 w838 w851 w871 w886 w900 w904 w918 w924 w963 w967 w992 w1010 w1018 w1028 w1058 w1065 w1080 w1141 w1163 w1171 w1201 w1229 w1242 w1254 w1267 w1279 w1311 w1322 w1333 w1350 w1353 w1387 w1401 w1439 w1465 w1473 w1480 w1497 w1516 w1534 w1555 w1565 w1578 w1584 w1595 w1600 w1613 w1620 w1632 w1641 w1649 w1653 w1661 w1669 w1696 w1703 w1715 w1743 w1758 w1764 w1770 w1776 w1782 w1788 w1794 w1800 w1806 w1812 w1818 w1826 w1832 w1845 w1853 w1862 w1872 w1881 w1891 w1911 w1933 w1955 w1977 w1999 w2022 w2044 w2066 w2088 w2106 w2116 w2126 w2163 w2168 w2178 w2193 w2243 w2257 w2262 w2303 w2322 w2331 w2344 w2357 w2373 w2391 w2408 w2423 w2443 w2453 w2469 w2491 w2514 w2532 w2547 w2561] -> w10
          tunnel: [w24 w609 w620 w633 w642 w659 w664 w674 w684 w693 w698 w721 w729 w736 w741 w744 w770 w812 w834 w839 w849 w860 w876 w897 w905 w909 w938 w964 w971 w993 w1007 w1015 w1027 w1060 w1067 w1070 w1127 w1148 w1172 w1188 w1221 w1234 w1255 w1268 w1280 w1305 w1315 w1326 w1348 w1360 w1382 w1410 w1442 w1463 w1471 w1479 w1499 w1520 w1538 w1558 w1567 w1575 w1586 w1592 w1604 w1609 w1618 w1629 w1638 w1646 w1654 w1664 w1678 w1693 w1707 w1724 w1745 w1759 w1765 w1771 w1777 w1783 w1789 w1795 w1801 w1807 w1813 w1819 w1827 w1837 w1847 w1856 w1866 w1877 w1886 w1897 w1907 w1929 w1951 w1973 w1995 w2018 w2040 w2062 w2084 w2102 w2119 w2131 w2164 w2169 w2179 w2207 w2248 w2258 w2263 w2286 w2315 w2332 w2346 w2362 w2375 w2393 w2401 w2421 w2430 w2458 w2473 w2486 w2510 w2533 w2539 w2560] -> w7
          tunnel: w6 -> [_ _ _ _ _ _ _ _ _ _ _ _ _ _ _ _ _ _ _ _ _ _ _ _ _ _ _ _ _ _ _ _ _ _ _ _ _ _ _ _ _ _ _ _ _ _ _ _ w1339 _ _ _ _ _ _ _ _ _ _ _ _ _ _ _ _ _ _ _ _ _ _ _ _ _ _ _ _ _ _ _ _ _ _ _ _ _ _ _ _ _ _ _ _ _ _ _ _ _ _ _ _ _ _ _ _ _ _ _ _ _ _ _ _ _ _ _ _ _ _ _ _ _ _ _ _ _ _ _ _ _ _ _]
          tunnel: w5 -> [w23 w609 w619 w633 w638 w659 w664 w674 w686 w693 w697 w721 w729 w736 w741 w747 w773 w812 w834 w839 w844 w868 w884 w897 w905 w912 w927 w964 w971 w993 w1008 w1016 w1031 w1060 w1067 w1071 w1137 w1155 w1172 w1192 w1226 w1238 w1255 w1268 w1275 w1307 w1318 w1329 w1346 w1356 w1383 w1409 w1448 w1464 w1472 w1482 w1496 w1519 w1539 w1559 w1568 w1576 w1583 w1593 w1601 w1611 w1619 w1630 w1639 w1647 w1655 w1662 w1672 w1692 w1704 w1723 w1746 w1759 w1765 w1771 w1777 w1783 w1789 w1795 w1801 w1807 w1813 w1819 w1827 w1837 w1847 w1856 w1866 w1877 w1886 w1897 w1903 w1927 w1947 w1969 w1991 w2013 w2035 w2057 w2079 w2101 w2120 w2131 w2164 w2169 w2184 w2199 w2249 w2258 w2261 w2291 w2316 w2332 w2337 w2353 w2366 w2387 w2400 w2415 w2431 w2451 w2466 w2485 w2507 w2525 w2540 w2554]
          tunnel: w4 -> [w21 w607 w616 w627 w641 w656 w662 _ w685 w691 w717 w724 w728 w733 w740 w745 w771 w798 w829 w838 w850 w870 w885 w900 w904 w918 w925 w963 w967 w992 w1010 w1018 w1028 w1058 w1065 w1080 w1141 w1163 w1171 w1201 w1229 w1242 w1254 w1267 w1279 w1310 w1321 w1332 w1350 w1362 w1387 w1402 w1440 w1465 w1473 w1480 w1498 w1515 w1534 w1555 w1565 w1578 w1584 w1595 w1600 w1613 w1620 w1632 w1641 w1649 w1653 w1661 w1669 w1691 w1703 w1717 w1744 w1758 w1764 w1770 w1776 w1782 w1788 w1794 w1800 w1806 w1812 w1818 w1822 w1835 w1841 w1851 w1861 w1871 w1884 w1895 w1910 w1932 w1954 w1976 w1998 w2021 w2043 w2065 w2087 w2105 w2118 w2126 w2163 w2168 w2178 w2193 w2243 w2257 w2262 w2303 w2318 w2331 w2340 w2361 w2377 w2388 w2406 w2424 w2434 w2452 w2472 w2490 w2512 w2529 w2545 w2562]
          frame "", "Idle" {
            # "executes when the state queue is empty"
            n7 = event shown="[6] \"Disable all AI Ref\": Value Change" {
              selector: w19 -> [_ _ _ w86 _ _ _ _ _ _ _ _ _ _ _ _ _ _ _ _ _ _ _ _ _ _ _ _ _ _ _ _ _ _ _ _ _ _ _ _ _ _ _ _ _ _ _ _ _ _ _ _ _ _ _ _ _ _ _]
              dyn-events: _ -> [_ _ _ _ _ _ _ _ _ _ _ _ _ _ _ _ _ _ _ _ _ _ _ _ _ _ _ _ _ _ _ _ _ _ _ _ _ _ _ _ _ _ _ _ _ _ _ _ _ _ _ _ _ _ _ _ _ _ _]
              timeout: w20 -> [_ _ _ _ _ _ _ _ _ _ _ _ _ _ _ _ _ _ _ _ _ _ _ _ _ _ _ _ _ _ _ _ _ _ _ _ _ _ _ _ _ _ _ _ _ _ _ _ _ _ _ _ _ _ _ _ _ _ _]
              tunnel: w26 -> [w40 w56 w65 w94 w141 w153 w164 w172 w176 _ w184 w204 w213 w223 w230 w240 w244 w249 w254 w259 w264 w269 w276 w283 w287 w292 w308 w323 w340 w350 w356 w362 w370 w377 w389 w399 w427 w429 w437 w445 w455 w470 w477 w482 w487 w492 w497 w505 w512 w519 w526 w532 w552 w561 w570 w579 w585 w591 w598]
              tunnel: [w39 w55 w64 w93 w140 w152 w163 w171 w177 _ w182 w205 w214 w224 w229 w239 w245 w250 w255 w260 w265 w270 w275 w282 w288 w293 w309 w322 w339 w349 w355 w361 w369 w376 w388 w398 w426 w430 w436 w444 w454 w469 w476 w483 w488 w493 w498 w504 w511 w518 w525 w531 w551 w560 w569 w578 w584 w590 w602] -> w25
              tunnel: [w33 w44 w63 w87 w139 w150 w161 w169 w174 _ w178 w197 w206 w217 w228 w235 w242 w247 w252 w257 w262 w267 w274 w281 w284 w290 w303 w311 w332 w341 w353 w359 w365 w374 w381 w391 w419 w431 w433 w441 w459 w463 w472 w480 w485 w490 w495 w502 w509 w516 w523 w530 w540 w559 w567 w576 w582 w587 w601] -> w24
              tunnel: w23 -> [w35 w48 w63 w88 w139 w150 w161 w169 w174 _ w178 w198 w206 w218 w228 w236 w242 w247 w252 w257 w262 w267 w274 w281 w284 w290 w295 w317 w334 w342 w353 w359 w365 w374 w382 w393 w420 w431 w433 w441 w459 w463 w472 w480 w485 w490 w495 w502 w509 w516 w523 w530 w550 w559 w567 w576 w582 w588 w601]
              tunnel: [w38 w53 w62 w92 w138 w151 w162 w170 w175 _ w183 w203 w212 w222 w227 w238 w243 w248 w253 w258 w263 w268 w272 w279 w285 w291 w306 w321 w337 w347 w354 w360 w367 w372 w386 w397 w424 w432 w438 w446 w457 w467 w474 w481 w486 w491 w496 w503 w510 w517 w524 w529 w543 w558 w568 w577 w583 w589 w600] -> w22
              tunnel: w21 -> [w37 w52 w61 w91 w138 w151 w162 w170 w175 _ w183 w201 w210 w220 w227 w234 w243 w248 w253 w258 w263 w268 w272 w279 w285 w291 w304 w320 w336 w346 w354 w360 w366 w373 w385 w396 w423 w432 w438 w446 w458 w466 w473 w481 w486 w491 w496 w503 w510 w517 w524 w529 w543 w558 w568 w577 w583 w589 w600]
              event "Input Gain": Value Change {
                # "redundant?"
                n8 = event-data() -> ("NewVal"=w30:cluster{"AI.Ch":string, "Gain":dbl}[])  [unwired: 1 in, 5 out]
                n9 = for {
                  tunnel: w30 -> [w42] mode=indexing
                  tunnel: [w41] -> w29 mode=indexing
                  n10 = Unbundle(w42) -> ("Gain"=w41:dbl)  [unwired: 1 out]
                }
                n11 = Unbundle By Name(w37) -> ("Lockin"=w36:refnum<class "Instrument.Lockin.lvclass">)
                n12 = call <userlib>:"Write Input Gain.vi"("error in (no error)"=w35, "InputGain"=w29, "Instrument.Lockin in"=w36) -> ("error out"=w34:errorcluster, "Instrument.Lockin out"=w32:refnum<class "Instrument.Lockin.lvclass">)  [unwired: 7 in]
                n13 = call "Initialize Input Gain.vi"("error in (no error)"=w34, "Instrument.DAQ"=w32) -> ("error out"=w33:errorcluster, "Input Gain"=w28:T40, "Instrument.DAQ out"=w31:refnum<class "Instrument.DAQ.lvclass">)  [unwired: 7 in]
                n14 = local write "Input Gain"(w28) -> ()
                n15 = Bundle By Name(cluster=w37, "Lockin"=w31) -> (w38:T44)
                n16 = call <vilib>:"Add State(s) to Queue__jki_lib_state_machine.vi"("State(s) in Front (\"\")"="DONE: Write CONFIG\nDONE: Set Input Gain" ("State(s) in Front (\"\")"), "State(s) in (\"\")"=w40) -> ("States Out"=w39:string)  [unwired: 13 in]
              }
              event "Output Gain": Value Change {
                n17 = event-data() -> ("NewVal"=w51:cluster{"AI.Ch":string, "Gain":dbl}[])  [unwired: 1 in, 5 out]
                n18 = for {
                  tunnel: w51 -> [w58] mode=indexing
                  tunnel: [w57] -> w50 mode=indexing
                  n19 = Unbundle(w58) -> ("Gain"=w57:dbl)  [unwired: 1 out]
                }
                n20 = Unbundle By Name(w52) -> ("Lockin"=w49:refnum<class "Instrument.Lockin.lvclass">)
                n21 = call <userlib>:"Write Output Gain.vi"("error in (no error)"=w48, "OutputGain"=w50, "Instrument.Lockin in"=w49) -> ("error out"=w46:errorcluster, "Instrument.Lockin out"=w47:refnum<class "Instrument.Lockin.lvclass">)  [unwired: 7 in]
                n22 = call "Initialize Ouput Gain.vi"("error in (no error)"=w46, "Instrument.DAQ"=w47) -> ("error out"=w44:errorcluster, "Output Gain"=w43:T40, "Instrument.DAQ out"=w45:refnum<class "Instrument.DAQ.lvclass">)  [unwired: 7 in]
                n23 = local write "Output Gain"(w43) -> ()
                n24 = Bundle By Name(cluster=w52, "Lockin"=w45) -> (w53:T44)
                n25 = call <vilib>:"Add State(s) to Queue__jki_lib_state_machine.vi"("State(s) in Front (\"\")"="DONE: Write CONFIG\nDONE: Set Output Gain" ("State(s) in Front (\"\")"), "State(s) in (\"\")"=w56) -> ("States Out"=w55:string)  [unwired: 13 in]
              }
              event "Start": Value Change {
                # "Start Button Value Change (pressed) Event\nIf DAQ=idle:\n1. Set Sampling to Continuous Samples\n2. Start acquisition\n3. Set Pause=False\n4. Set timout=10\n\nIf DAQ=running:\n1. Do nothing"
                n26 = event-data() -> ()  [unwired: 1 in, 2 out]
                n27 = Unbundle By Name(w61) -> ("DAQ state"=w60:T45)
                n28 = case shown="\"idle\", Default" w60 {
                  tunnel: [w72 "" ("State with Arguments")] -> w59
                  tunnel: w61 -> [w78 w84]
                  tunnel: [w77 w84] -> w62
                  frame "idle", Default {
                    w73 = 10123 items=["Finite Samples"=10178, "Continuous Samples"=10123] ("Sample Mode")
                    n29 = local write "Pause"(FALSE ("Pause")) -> ()
                    n30 = Format Into String(w73) -> (resulting string=w74:string)  [unwired: 3 in, 1 out]
                    n31 = Format Into String(T15."start" ("State")) -> (resulting string=w82:string)  [unwired: 3 in, 1 out]
                    n32 = First Call?() -> (First Call?: T/F=w69:bool)
                    n33 = call <vilib>:"Build State String with Arguments__JKI_lib_State_Machine.vi"("Arguments (\"\")"=w74, "State"="TODO: Set Sampling" ("f")) -> ("State with Arguments"=w71:string)  [unwired: 4 in]
                    n34 = call <vilib>:"Build State String with Arguments__JKI_lib_State_Machine.vi"("Arguments (\"\")"=w82, "State"="DONE: Set State" ("f")) -> ("State with Arguments"=w70:string)  [unwired: 4 in]
                    n35 = Select(t="Macro: Update Sampling" ("f"), s=w69, f="") -> (s? t:f=w67:string)
                    n36 = call <vilib>:"Add State(s) to Queue__jki_lib_state_machine.vi"("State(s) in Front (\"\")"=w67, "State(s) in (\"\")"=w71, "State(s) at Back (\"\")"=w70) -> ("States Out"=w72:string)  [unwired: 12 in]
                    n37 = Bundle By Name(cluster=w78, "to"=-1) -> (w77:T44)
                  }
                  frame "created" {
                  }
                }
                n38 = call <vilib>:"Add State(s) to Queue__jki_lib_state_machine.vi"("State(s) in (\"\")"=w65, "State(s) at Back (\"\")"=w59) -> ("States Out"=w64:string)  [unwired: 13 in]
              }
              event "Pause": Value Change {
                # "Pause Button Value Change (pressed) Event\nPause=True & DAQ=running:\n1. Set Sampling to Finite Samples\n2. STOP acquisition\n3. Set timeout=-1 (wait forever)\nPause=True & DAQ=idle\n1. Set timeout=-1\n2. Set Sampling to Finite\nPause=False:\n1. send T=Val(Sgnl) to Start"
                n39 = event-data() -> ("NewVal"=w90:bool)  [unwired: 1 in]
                n40 = Unbundle By Name(w91) -> ("DAQ state"=w89:T45)
                n41 = Flush Event Queue(0:w86, 3:w88) -> (11:w87:errorcluster)  [unwired: 4 in, 2 out]
                n42 = case shown="True" w90 {
                  tunnel: [w96 "" ("States Out")] -> w85
                  tunnel: w91 -> [w98 w124]
                  tunnel: [w97 w124] -> w92
                  tunnel: w89 -> [w95 _]
                  frame True {
                    n43 = case shown="\"started\"" w95 {
                      tunnel: w98 -> [w103 w119]
                      tunnel: [w102 w118] -> w97
                      tunnel: [w99 w109] -> w96
                      frame "idle", Default {
                        w105 = 10178 items=["Finite Samples"=10178, "Continuous Samples"=10123] ("Sample Mode")
                        n44 = Format Into String(w105) -> (resulting string=w106:string)  [unwired: 3 in, 1 out]
                        n45 = call <vilib>:"Build State String with Arguments__JKI_lib_State_Machine.vi"("Arguments (\"\")"=w106, "State"="TODO: Set Sampling" ("f")) -> ("State with Arguments"=w100:string)  [unwired: 4 in]
                        n46 = call <vilib>:"Add State(s) to Queue__jki_lib_state_machine.vi"("State(s) at Back (\"\")"=w100) -> ("States Out"=w99:string)  [unwired: 14 in]
                        n47 = Bundle By Name(cluster=w103, "to"=100) -> (w102:T44)
                      }
                      frame "started" {
                        w114 = 10178 items=["Finite Samples"=10178, "Continuous Samples"=10123] ("Sample Mode")
                        n48 = Format Into String(T15."stop" ("State")) -> (resulting string=w122:string)  [unwired: 3 in, 1 out]
                        n49 = Format Into String(w114) -> (resulting string=w115:string)  [unwired: 3 in, 1 out]
                        n50 = call <vilib>:"Build State String with Arguments__JKI_lib_State_Machine.vi"("Arguments (\"\")"=w122, "State"="DONE: Set State" ("f")) -> ("State with Arguments"=w107:string)  [unwired: 4 in]
                        n51 = call <vilib>:"Build State String with Arguments__JKI_lib_State_Machine.vi"("Arguments (\"\")"=w115, "State"="TODO: Set Sampling" ("f")) -> ("State with Arguments"=w108:string)  [unwired: 4 in]
                        n52 = local write "Status"("Finite Acquisition" ("Status")) -> ()
                        n53 = call <vilib>:"Add State(s) to Queue__jki_lib_state_machine.vi"("State(s) in Front (\"\")"="TODO: Set AO Zero Amplitude" ("f"), "State(s) in (\"\")"=w108, "State(s) at Back (\"\")"=w107) -> ("States Out"=w111:string)  [unwired: 12 in]
                        n54 = Bundle By Name(cluster=w119, "to"=100) -> (w118:T44)
                        n55 = call <vilib>:"Add State(s) to Queue__jki_lib_state_machine.vi"("State(s) in Front (\"\")"=w111, "State(s) at Back (\"\")"="DONE: Set AO" ("f")) -> ("States Out"=w109:string)  [unwired: 13 in]
                      }
                    }
                  }
                  frame False {
                    n56 = property on="Start" class="Bool (strict)"("Val(Sgnl)"=TRUE ("Value (Signaling)")) -> ()  [unwired: 2 in, 2 out]
                  }
                }
                n57 = call <vilib>:"Add State(s) to Queue__jki_lib_state_machine.vi"("State(s) in Front (\"\")"=w85, "State(s) in (\"\")"=w94) -> ("States Out"=w93:string)  [unwired: 13 in]
              }
              event "Trigger": Value Change {
                w136 = 10178 items=["Finite Samples"=10178, "Continuous Samples"=10123] ("Sample Mode")
                # "Trigger Button Value Change (pressed) Event\nIf DAQ=idle:\n1. put into finite sample mode\n2. start (one) acquisition)\nIf DAQ=running:\n1. Stop current acquisition\n2. put into finite sample mode\n3. start (one) acquisition)"
                n58 = event-data() -> ()  [unwired: 1 in, 2 out]
                n59 = disable-structure shown="Disabled" {
                  frame Disabled {
                    n60 = local write "Trigger"(FALSE ("Trigger")) -> ()
                  }
                  frame Enabled {
                  }
                }
                n61 = Unbundle By Name(w138) -> ("DAQ state"=w137:T45)
                n62 = case shown="\"created\"" w137 {
                  tunnel: ["" ("State with Arguments") w144] -> w128
                  frame "idle", Default {
                  }
                  frame "created" {
                    n63 = Format Into String(T15."stop" ("State")) -> (resulting string=w147:string)  [unwired: 3 in, 1 out]
                    n64 = call <vilib>:"Build State String with Arguments__JKI_lib_State_Machine.vi"("Arguments (\"\")"=w147, "State"="DONE: Set State" ("f")) -> ("State with Arguments"=w144:string)  [unwired: 4 in]
                  }
                }
                n65 = local write "Pause"(TRUE ("Pause")) -> ()
                n66 = Format Into String(w136) -> (resulting string=w135:string)  [unwired: 3 in, 1 out]
                n67 = Format Into String(T15."start" ("State")) -> (resulting string=w131:string)  [unwired: 3 in, 1 out]
                n68 = call <vilib>:"Build State String with Arguments__JKI_lib_State_Machine.vi"("Arguments (\"\")"=w135, "State"="TODO: Set Sampling" ("f")) -> ("State with Arguments"=w130:string)  [unwired: 4 in]
                n69 = call <vilib>:"Build State String with Arguments__JKI_lib_State_Machine.vi"("Arguments (\"\")"=w131, "State"="DONE: Set State" ("f")) -> ("State with Arguments"=w129:string)  [unwired: 4 in]
                n70 = call <vilib>:"Add State(s) to Queue__jki_lib_state_machine.vi"("State(s) in Front (\"\")"=w128, "State(s) in (\"\")"=w130, "State(s) at Back (\"\")"=w129) -> ("States Out"=w127:string)  [unwired: 12 in]
                n71 = call <vilib>:"Add State(s) to Queue__jki_lib_state_machine.vi"("State(s) in Front (\"\")"=w127, "State(s) in (\"\")"=w141) -> ("States Out"=w140:string)  [unwired: 13 in]
              }
              event "Reset": Value Change {
                # "RESET Button Value Change (pressed) Event\n1. Call 4461: SETUP State to calculate new Sampling\ninformation\n2. If sampling information changes, \"Sampling: value\nchange event will be triggered.\n3. Sampling: Value Change will call Stop, Set Sampling, Start"
                n72 = event-data() -> ()  [unwired: 1 in, 1 out]
                n73 = disable-structure shown="Disabled" {
                  frame Disabled {
                    n74 = Format Into String(Set_State-enum."reset" ("State")) -> (resulting string=w156:string)  [unwired: 3 in, 1 out]
                    n75 = call <vilib>:"Build State String with Arguments__JKI_lib_State_Machine.vi"("Arguments (\"\")"=w156, "State"="DONE: Set State" ("f")) -> ()  [unwired: 4 in, 1 out]
                  }
                  frame Enabled {
                  }
                }
                n76 = local write "Reset"(FALSE ("Reset")) -> ()
                n77 = call <vilib>:"Add State(s) to Queue__jki_lib_state_machine.vi"("State(s) in Front (\"\")"="Macro: Initialize UI\nMacro: Reset DAQ SMO\n//TODO: Update Plot Names >>Reset" ("State(s) in Front (\"\")"), "State(s) in (\"\")"=w153) -> ("States Out"=w152:string)  [unwired: 13 in]
              }
              event "Disable all AI Ref": Value Change {
                # "Measure Offset Button Value Change (pressed) Event\n1. send \"measure offset\" command to DAQ"
                n78 = event-data() -> ()  [unwired: 1 in, 1 out]
                n79 = local write "Disable all AI Ref"(FALSE ("Measure\nOffset")) -> ()
                n80 = call <vilib>:"Build State String with Arguments__JKI_lib_State_Machine.vi"("Arguments (\"\")"="Disable" ("Arguments (\"\")"), "State"="UI: Update AI Reference Channels" ("State(s) in Front (\"\")")) -> ("State with Arguments"=w160:string)  [unwired: 4 in]
                n81 = call <vilib>:"Add State(s) to Queue__jki_lib_state_machine.vi"("State(s) in Front (\"\")"=w160, "State(s) in (\"\")"=w164) -> ("States Out"=w163:string)  [unwired: 13 in]
              }
              event "Enable only AI Ref1": Value Change {
                # "Measure Offset Button Value Change (pressed) Event\n1. send \"measure offset\" command to DAQ"
                n82 = event-data() -> ()  [unwired: 1 in, 1 out]
                n83 = local write "Enable only AI Ref1"(FALSE ("Measure\nOffset")) -> ()
                n84 = call <vilib>:"Build State String with Arguments__JKI_lib_State_Machine.vi"("Arguments (\"\")"="All 1" ("Arguments (\"\")"), "State"="UI: Update AI Reference Channels" ("State(s) in Front (\"\")")) -> ("State with Arguments"=w168:string)  [unwired: 4 in]
                n85 = call <vilib>:"Add State(s) to Queue__jki_lib_state_machine.vi"("State(s) in Front (\"\")"=w168, "State(s) in (\"\")"=w172) -> ("States Out"=w171:string)  [unwired: 13 in]
              }
              event "Update": Value Change {
                # "Update Value Change (pressed) Event\ncall: AUX: Set AUX"
                n86 = event-data() -> ()  [unwired: 1 in, 6 out]
                n87 = call <vilib>:"Add State(s) to Queue__jki_lib_state_machine.vi"("State(s) in Front (\"\")"="AUX: Set AUX" ("State(s) in Front (\"\")"), "State(s) in (\"\")"=w176) -> ("States Out"=w177:string)  [unwired: 13 in]
              }
              event event #0x53 {
                n88 = event-data() -> ()  [unwired: 1 in, 7 out]
              }
              event Timeout {
                # "#done"
                n89 = event-data() -> ()  [unwired: 1 in, 1 out]
                n90 = Unbundle By Name(w183) -> ("DAQ state"=w179:T45)
                n91 = case shown="\"idle\"" w179 {
                  tunnel: [w187 w191 w193] -> w181
                  frame "idle" {
                    n92 = call "Spinner.vi"("Enum"=enum16{"Spinner 1", "Spinner 2", "Spinner 3"}."Spinner 1") -> ("Spinner Out"=w185:string)  [unwired: 4 in]
                    n93 = Concatenate Strings("Idle     " ("Status"), w185) -> (w187:string)
                  }
                  frame "created" {
                    n94 = call "Spinner.vi"("Enum"=enum16{"Spinner 1", "Spinner 2", "Spinner 3"}."Spinner 1") -> ("Spinner Out"=w189:string)  [unwired: 4 in]
                    n95 = Concatenate Strings("Created  " ("Status"), w189) -> (w191:string)
                  }
                  frame Default {
                    n96 = local read "Status"() -> (w193:string)
                  }
                }
                "Status" <- w181
                n97 = call <vilib>:"Add State(s) to Queue__jki_lib_state_machine.vi"("State(s) in Front (\"\")"="" ("t"), "State(s) in (\"\")"=w184) -> ("States Out"=w182:string)  [unwired: 13 in]
              }
              event "REF Channels": Value Change {
                # "if number of lockin channels is not the same as before reset the lockin\nupdate: no, just reset phase...?"
                n98 = event-data() -> ("NewVal"=w194:T4, "OldVal"=w195:T4)  [unwired: 1 in]
                n99 = Unbundle By Name(w201) -> ("Lockin"=w200:refnum<class "Instrument.Lockin.lvclass">)  [unwired: 1 out]
                n100 = Not Equal?(x=w194, y=w195) -> ()  [unwired: 1 out]
                n101 = call <userlib>:"Write Channels_ REF.vi"("error in (no error)"=w198, "Channels: REF"=w194, "Instrument.Lockin in"=w200) -> ("error out"=w197:errorcluster, "Instrument.Lockin out"=w199:refnum<class "Instrument.Lockin.lvclass">)  [unwired: 7 in]
                n102 = Bundle By Name(cluster=w201, "Lockin"=w199) -> (w203:T44)
                n103 = call <vilib>:"Add State(s) to Queue__jki_lib_state_machine.vi"("State(s) in (\"\")"="DONE: Adjust Channels\nUI: Update Rings\nTODO: Update Plot Names\nDONE: Write CONFIG\nDONE: Set REF\nDONE: Reset Phase" ("f")) -> ("States Out"=w202:string)  [unwired: 14 in]
                n104 = call <vilib>:"Add State(s) to Queue__jki_lib_state_machine.vi"("State(s) in Front (\"\")"=w202, "State(s) in (\"\")"=w204) -> ("States Out"=w205:string)  [unwired: 13 in]
              }
              event "AI Channels": Value Change {
                n105 = event-data() -> ("NewVal"=w207:T2)  [unwired: 1 in]
                n106 = Unbundle By Name(w210) -> ("Lockin"=w209:refnum<class "Instrument.Lockin.lvclass">)
                n107 = Bundle By Name(cluster=w209, "AI"=w207) -> (w208:refnum<class "Instrument.Lockin.lvclass">)
                n108 = Bundle By Name(cluster=w210, "Lockin"=w208) -> (w212:T44)
                n109 = call <vilib>:"Add State(s) to Queue__jki_lib_state_machine.vi"("State(s) in Front (\"\")"="UI: Update Rings\nDONE: Write CONFIG\nDONE: Set AI" ("f"), "State(s) in (\"\")"=w213) -> ("States Out"=w214:string)  [unwired: 13 in]
              }
              event "AO Channels": Value Change {
                n110 = event-data() -> ("NewVal"=w215:T3)  [unwired: 1 in, 5 out]
                n111 = Unbundle By Name(w220) -> ("Lockin"=w219:refnum<class "Instrument.Lockin.lvclass">)
                n112 = call <userlib>:"Write Channels_ AO.vi"("error in (no error)"=w218, "Channels: AO"=w215, "Instrument.Lockin in"=w219) -> ("error out"=w217:errorcluster, "Instrument.Lockin out"=w216:refnum<class "Instrument.Lockin.lvclass">)  [unwired: 7 in]
                n113 = Bundle By Name(cluster=w220, "Lockin"=w216) -> (w222:T44)
                n114 = call <vilib>:"Add State(s) to Queue__jki_lib_state_machine.vi"("State(s) in Front (\"\")"="DONE: Adjust Channels\nUI: Update Rings\nDONE: Write CONFIG\nDONE: Set AO" ("f"), "State(s) in (\"\")"=w223) -> ("States Out"=w224:string)  [unwired: 13 in]
              }
              event "Auto x*F1", "Max Fs Refresh Rate (Hz)", "Sampling Mode", "decimating factor": Value Change {
                # "#done mostly"
                n115 = event-data() -> ()  [unwired: 1 in, 6 out]
                n116 = call <vilib>:"Add State(s) to Queue__jki_lib_state_machine.vi"("State(s) in Front (\"\")"="Macro: Update Sampling" ("State(s) in Front (\"\")")) -> ("States Out"=w226:string)  [unwired: 14 in]
                n117 = call <vilib>:"Add State(s) to Queue__jki_lib_state_machine.vi"("State(s) in Front (\"\")"=w226, "State(s) in (\"\")"=w230) -> ("States Out"=w229:string)  [unwired: 13 in]
              }
              event "Sampling": Value Change {
                # "#done\nmostly"
                n118 = event-data() -> ("NewVal"=w233:cluster{"Fs":dbl, "#s":i32})  [unwired: 1 in, 1 out]
                n119 = Unbundle By Name(w234) -> ("Lockin"=w232:refnum<class "Instrument.Lockin.lvclass">)  [unwired: 1 out]
                n120 = call <userlib>:"Write sampling.vi"("error in (no error)"=w236, "sampling"=w233, "Instrument.Lockin in"=w232) -> ("error out"=w235:errorcluster, "Instrument.Lockin out"=w237:refnum<class "Instrument.Lockin.lvclass">)  [unwired: 7 in]
                n121 = Bundle By Name(cluster=w234, "Lockin"=w237) -> (w238:T44)
                n122 = call <vilib>:"Add State(s) to Queue__jki_lib_state_machine.vi"("State(s) in Front (\"\")"="Macro: Update Sampling" ("State(s) in Front (\"\")"), "State(s) in (\"\")"=w240) -> ("States Out"=w239:string)  [unwired: 13 in]
              }
              event "AI Graph All": Value Change {
                # "#done"
                # "X Axis, Y Axis Out Value Change (pressed) Event\ncall: UI: Update Waveform Graph Labels"
                n123 = event-data() -> ()  [unwired: 1 in, 6 out]
                n124 = call <vilib>:"Add State(s) to Queue__jki_lib_state_machine.vi"("State(s) in Front (\"\")"="DONE: AI Graph Plot Visible >> All" ("State(s) in Front (\"\")"), "State(s) in (\"\")"=w244) -> ("States Out"=w245:string)  [unwired: 13 in]
              }
              event "AI Graph None": Value Change {
                # "#done"
                # "X Axis, Y Axis Out Value Change (pressed) Event\ncall: UI: Update Waveform Graph Labels"
                n125 = event-data() -> ()  [unwired: 1 in, 6 out]
                n126 = call <vilib>:"Add State(s) to Queue__jki_lib_state_machine.vi"("State(s) in Front (\"\")"="DONE: AI Graph Plot Visible >> None" ("State(s) in Front (\"\")"), "State(s) in (\"\")"=w249) -> ("States Out"=w250:string)  [unwired: 13 in]
              }
              event "AO Graph All": Value Change {
                # "#done"
                # "X Axis, Y Axis Out Value Change (pressed) Event\ncall: UI: Update Waveform Graph Labels"
                n127 = event-data() -> ()  [unwired: 1 in, 6 out]
                n128 = call <vilib>:"Add State(s) to Queue__jki_lib_state_machine.vi"("State(s) in Front (\"\")"="DONE: AO Graph Plot Visible >> All" ("State(s) in Front (\"\")"), "State(s) in (\"\")"=w254) -> ("States Out"=w255:string)  [unwired: 13 in]
              }
              event "AO Graph None": Value Change {
                # "#done"
                # "X Axis, Y Axis Out Value Change (pressed) Event\ncall: UI: Update Waveform Graph Labels"
                n129 = event-data() -> ()  [unwired: 1 in, 6 out]
                n130 = call <vilib>:"Add State(s) to Queue__jki_lib_state_machine.vi"("State(s) in Front (\"\")"="DONE: AO Graph Plot Visible >> None" ("State(s) in Front (\"\")"), "State(s) in (\"\")"=w259) -> ("States Out"=w260:string)  [unwired: 13 in]
              }
              event "Lockin 1 All": Value Change {
                # "#done"
                # "X Axis, Y Axis Out Value Change (pressed) Event\ncall: UI: Update Waveform Graph Labels"
                n131 = event-data() -> ()  [unwired: 1 in, 6 out]
                n132 = call <vilib>:"Add State(s) to Queue__jki_lib_state_machine.vi"("State(s) in Front (\"\")"="DONE: Lockin 1 Plot Visible >> All" ("State(s) in Front (\"\")"), "State(s) in (\"\")"=w264) -> ("States Out"=w265:string)  [unwired: 13 in]
              }
              event "Lockin 1 None": Value Change {
                # "#done"
                # "X Axis, Y Axis Out Value Change (pressed) Event\ncall: UI: Update Waveform Graph Labels"
                n133 = event-data() -> ()  [unwired: 1 in, 6 out]
                n134 = call <vilib>:"Add State(s) to Queue__jki_lib_state_machine.vi"("State(s) in Front (\"\")"="DONE: Lockin 1 Plot Visible >> None" ("State(s) in Front (\"\")"), "State(s) in (\"\")"=w269) -> ("States Out"=w270:string)  [unwired: 13 in]
              }
              event "Get Calibration": Value Change {
                # "#done"
                # "Self Calibrate Mode Button Value Change (pressed) Event"
                n135 = event-data() -> ()  [unwired: 1 in, 2 out]
                n136 = local write "Get Calibration"(FALSE ("Self Calibrate")) -> ()
                n137 = call <vilib>:"Add State(s) to Queue__jki_lib_state_machine.vi"("State(s) in Front (\"\")"="DONE: Calibration >> False" ("f"), "State(s) in (\"\")"=w276) -> ("States Out"=w275:string)  [unwired: 13 in]
              }
              event "Self Calibrate": Value Change {
                # "#done"
                # "Self Calibrate Mode Button Value Change (pressed) Event"
                n138 = event-data() -> ()  [unwired: 1 in, 2 out]
                n139 = local write "Self Calibrate"(FALSE ("Self Calibrate")) -> ()
                n140 = property on="Pause" class="Bool (strict)"("Val(Sgnl)"=TRUE ("Value (Signaling)")) -> ()  [unwired: 2 in, 2 out]
                n141 = call <vilib>:"Add State(s) to Queue__jki_lib_state_machine.vi"("State(s) in Front (\"\")"="\nDONE: Calibration >> True" ("f"), "State(s) in (\"\")"=w283) -> ("States Out"=w282:string)  [unwired: 13 in]
              }
              event "AI Simulation mode": Value Change {
                # "#done"
                n142 = event-data() -> ()  [unwired: 1 in, 1 out]
                n143 = call <vilib>:"Add State(s) to Queue__jki_lib_state_machine.vi"("State(s) in Front (\"\")"="DONE: Write CONFIG\nDONE: Set AI Config" ("State(s) in Front (\"\")"), "State(s) in (\"\")"=w287) -> ("States Out"=w288:string)  [unwired: 13 in]
              }
              event "Link Frequencies", "Limit Amplitudes", "AO freq link": Value Change {
                # "#done"
                # "Same f\", \"Limit Amp\", \"AO freq link\": Value Change Value Change (pressed) Event\ncall:\nData: Adjust Channels\nConfiguration: Write\nLockin SMO: Set AO\nLockin SMO: Set REF"
                n144 = event-data() -> ()  [unwired: 1 in, 6 out]
                n145 = call <vilib>:"Add State(s) to Queue__jki_lib_state_machine.vi"("State(s) in Front (\"\")"="DONE: Adjust Channels\nUI: Update Rings\nDONE: Write CONFIG\nDONE: Set AO\nDONE: Set REF" ("f"), "State(s) in (\"\")"=w292) -> ("States Out"=w293:string)  [unwired: 13 in]
              }
              event "DAQ Config": Value Change {
                w298 = -1 items=["Default"=-1, "RSE"=10083, "Differential"=10106, "Pseudodifferential"=12529] ("output terminal configuration")
                w299 = -1 items=["Default"=-1, "RSE"=10083, "NRSE"=10078, "Differential"=10106, "Pseudodifferential"=12529] ("input terminal configuration")
                # "#done\nmost of these commands are taken care \nof Instrument.DAQ itself"
                n146 = event-data() -> ("NewVal"=w297:T5)  [unwired: 1 in]
                n147 = Unbundle By Name(w304) -> ("Lockin"=w300:refnum<class "Instrument.Lockin.lvclass">)
                n148 = call "config UI to not UI (AO and AI).vi"("output terminal configuration"=w298, "input terminal configuration"=w299, "New Ch []"=w297) -> ("AO Config"=w302:T46, "AI Config"=w296:T50)  [unwired: 7 in]
                n149 = call <userlib>:"Write AI Configuration.vi"("error in (no error)"=w295, "AI Configuration"=w296, "Instrument.Lockin in"=w300) -> ("error out"=w294:errorcluster, "Instrument.Lockin out"=w301:refnum<class "Instrument.Lockin.lvclass">)  [unwired: 7 in]
                n150 = call <userlib>:"Write AO Configuration.vi"("error in (no error)"=w294, "AO Configuration"=w302, "Instrument.Lockin in"=w301) -> ("error out"=w303:errorcluster, "Instrument.Lockin out"=w305:refnum<class "Instrument.Lockin.lvclass">)  [unwired: 7 in]
                n151 = Bundle By Name(cluster=w304, "Lockin"=w305) -> (w306:T44)
                n152 = call <vilib>:"Add State(s) to Queue__jki_lib_state_machine.vi"("State(s) in Front (\"\")"="DONE: Write CONFIG\nDONE: Set AO Config\nDONE: Set AI Config\nDONE: Initialize REF Ch\nDONE: Initialize AO Ch\nDONE: Initialize AI Ch\nDONE: Initialize Gains\nTODO: Update Plot Names" ("State(s) in Front (\"\")"), "State(s) in (\"\")"=w308) -> ("States Out"=w309:string)  [unwired: 13 in]
              }
              event User Event {
                # "#done"
                n153 = event-data() -> ("Results"=w316:T53)  [unwired: 1 in, 4 out]
                n154 = Unbundle By Name(w320) -> ("Lockin"=w319:refnum<class "Instrument.Lockin.lvclass">)
                n155 = call <userlib>:"Write Results.vi"("error in (no error)"=w317, "Results"=w316, "Instrument.Lockin in"=w319) -> ("error out"=w313:errorcluster, "Instrument.Lockin out"=w318:refnum<class "Instrument.Lockin.lvclass">)  [unwired: 7 in]
                n156 = call <userlib>:"MGI Milliseconds Since Last Call.vi"("Error In"=w313) -> ("ms"=→"Refresh time (ms)":u32, "Error Out"=w311:errorcluster)  [unwired: 5 in]
                n157 = Bundle By Name(cluster=w320, "Lockin"=w318) -> (w321:T44)
                n158 = call <userlib>:"Periodic Trigger__ogtk.vi"("time (ms)"=u32 100) -> ("Triggered"=w315:bool)  [unwired: 12 in, 2 out]
                n159 = case shown="True" w315 {
                  tunnel: ["" ("State(s) in Front (\"\")") w327] -> w310
                  frame False {
                  }
                  frame True {
                    n160 = local read "Tab Control 2"() -> (w328:T13)
                    n161 = case shown="\"PS\"" w328 {
                      tunnel: ["" ("State(s) in Front (\"\")") "4461: FFT" ("State(s) in Front (\"\")")] -> w326
                      frame Default {
                      }
                      frame "PS" {
                      }
                    }
                    n162 = call <vilib>:"Add State(s) to Queue__jki_lib_state_machine.vi"("State(s) in Front (\"\")"="4461: OUT\nDONE: Update Waveform Graphs\nDONE: Sync AO AI Plot Visibility\nDONE: Update Lockin Graphs\nDONE: Sync Lockin Plot Visibility\nDONE: Update Sweep Timer" ("State(s) in Front (\"\")"), "State(s) at Back (\"\")"=w326) -> ("States Out"=w327:string)  [unwired: 13 in]
                  }
                }
                n163 = call <vilib>:"Add State(s) to Queue__jki_lib_state_machine.vi"("State(s) in Front (\"\")"=w310, "State(s) in (\"\")"=w323) -> ("States Out"=w322:string)  [unwired: 13 in]
              }
              event User Event {
                # "#done"
                n164 = event-data() -> ("Channels: AO"=w331:T54)  [unwired: 1 in, 4 out]
                n165 = Unbundle By Name(w336) -> ("Lockin"=w335:refnum<class "Instrument.Lockin.lvclass">)
                n166 = call <userlib>:"Write Channels_ AO.vi"("error in (no error)"=w334, "Channels: AO"=w331, "Instrument.Lockin in"=w335) -> ("error out"=w332:errorcluster, "Instrument.Lockin out"=w333:refnum<class "Instrument.Lockin.lvclass">)  [unwired: 7 in]
                n167 = local write "AO Channels"(w331) -> ()
                n168 = Bundle By Name(cluster=w336, "Lockin"=w333) -> (w337:T44)
                n169 = call <vilib>:"Add State(s) to Queue__jki_lib_state_machine.vi"("State(s) in Front (\"\")"="" ("State(s) in Front (\"\")"), "State(s) in (\"\")"=w340) -> ("States Out"=w339:string)  [unwired: 13 in]
              }
              event User Event {
                # "#done"
                n170 = event-data() -> ("Channels: REF"=w343:T57)  [unwired: 1 in, 4 out]
                n171 = Unbundle By Name(w346) -> ("Lockin"=w345:refnum<class "Instrument.Lockin.lvclass">)
                n172 = call <userlib>:"Write Channels_ REF.vi"("error in (no error)"=w342, "Channels: REF"=w343, "Instrument.Lockin in"=w345) -> ("error out"=w341:errorcluster, "Instrument.Lockin out"=w344:refnum<class "Instrument.Lockin.lvclass">)  [unwired: 7 in]
                n173 = Bundle By Name(cluster=w346, "Lockin"=w344) -> (w347:T44)
                n174 = call <vilib>:"Add State(s) to Queue__jki_lib_state_machine.vi"("State(s) in Front (\"\")"="" ("State(s) in Front (\"\")"), "State(s) in (\"\")"=w350) -> ("States Out"=w349:string)  [unwired: 13 in]
              }
              event User Event {
                # "#done"
                # "Check Calibrate Mode Button Value Change (pressed) Event"
                n175 = event-data() -> ("getDAQconfig"=w351:T59)  [unwired: 1 in]
                n176 = property on="DAQ Config" class="Arr (strict)"("Val(Sgnl)"=w351) -> ()  [unwired: 2 in, 2 out]
                n177 = call <vilib>:"Add State(s) to Queue__jki_lib_state_machine.vi"("State(s) in (\"\")"=w356, "State(s) at Back (\"\")"="" ("State(s) at Back (\"\")")) -> ("States Out"=w355:string)  [unwired: 13 in]
              }
              event User Event {
                # "#done"
                # "Check Calibrate Mode Button Value Change (pressed) Event"
                n178 = event-data() -> ("getCalibration"=→"Cal Info":T62)  [unwired: 1 in]
                n179 = call <vilib>:"Add State(s) to Queue__jki_lib_state_machine.vi"("State(s) in (\"\")"=w362, "State(s) at Back (\"\")"="" ("State(s) at Back (\"\")")) -> ("States Out"=w361:string)  [unwired: 13 in]
              }
              event User Event {
                # "#done"
                n180 = event-data() -> ("Sweep_AO"=w364:waveform(dbl)[], "Sweep_AI"=w363:waveform(dbl)[])  [unwired: 1 in, 4 out]
                n181 = Bundle By Name(cluster=w366, "SweepWaveforms.Sweep_AO"=w364, "SweepWaveforms.Sweep_AI"=w363) -> (w367:T44)
                n182 = call <vilib>:"Add State(s) to Queue__jki_lib_state_machine.vi"("State(s) in Front (\"\")"="DONE: Update Sweep WFMs Graphs" ("State(s) in Front (\"\")"), "State(s) in (\"\")"=w370) -> ("States Out"=w369:string)  [unwired: 13 in]
              }
              event User Event {
                # "#done"
                n183 = event-data() -> ("getSweepResults"=w371:T64)  [unwired: 1 in, 4 out]
                n184 = Bundle By Name(cluster=w373, "SweepResults"=w371) -> (w372:T44)
                n185 = call <vilib>:"Add State(s) to Queue__jki_lib_state_machine.vi"("State(s) in Front (\"\")"="DONE: Update Sweep Results Graphs" ("State(s) in Front (\"\")"), "State(s) in (\"\")"=w377) -> ("States Out"=w376:string)  [unwired: 13 in]
              }
              event User Event {
                # "#done"
                n186 = event-data() -> ("X"=w380:waveform(dbl)[], "Y"=w379:waveform(dbl)[])  [unwired: 1 in]
                n187 = Bundle("X"=w380, "Y"=w379) -> (w378:T65)  [unwired: 1 in]
                n188 = Unbundle By Name(w385) -> ("Lockin"=w384:refnum<class "Instrument.Lockin.lvclass">)
                n189 = call <userlib>:"Write REF WFM.vi"("error in (no error)"=w382, "Reference"=w378, "Instrument.Lockin in"=w384) -> ("error out"=w381:errorcluster, "Instrument.Lockin out"=w383:refnum<class "Instrument.Lockin.lvclass">)  [unwired: 7 in]
                n190 = Bundle By Name(cluster=w385, "Lockin"=w383) -> (w386:T44)
                n191 = call <vilib>:"Add State(s) to Queue__jki_lib_state_machine.vi"("State(s) in Front (\"\")"="" ("State(s) in Front (\"\")"), "State(s) in (\"\")"=w389) -> ("States Out"=w388:string)  [unwired: 13 in]
              }
              event User Event {
                # "#done"
                n192 = event-data() -> ("getAI"=w390:T66)  [unwired: 1 in, 4 out]
                n193 = Unbundle By Name(w396) -> ("Lockin"=w395:refnum<class "Instrument.Lockin.lvclass">)
                n194 = call <userlib>:"Write AI WFM.vi"("error in (no error)"=w393, "AI WFM"=w390, "Instrument.Lockin in"=w395) -> ("error out"=w392:errorcluster, "Instrument.Lockin out"=w394:refnum<class "Instrument.Lockin.lvclass">)  [unwired: 7 in]
                n195 = Bundle By Name(cluster=w396, "Lockin"=w394) -> (w397:T44)
                n196 = disable-structure shown="Disabled" {
                  disable-tunnel: w392 -> [w406 w417]
                  disable-tunnel: [w405 w417] -> w391
                  disable-tunnel: w390 -> [w404 _]
                  frame Enabled {
                    n197 = Index Array(array=w404) -> (element=w416:waveform(dbl))  [unwired: 1 in]
                    n198 = local read "Refresh time (ms)"() -> (w400:u32)
                    n199 = call-poly <vilib>:"Waveform Duration.vi"("error in (no error)"=w406, "waveform in"=w416) -> ("error out"=w405:errorcluster, "duration"=w415:dbl)  [unwired: 7 in, 1 out]
                    n200 = Multiply(x=w415, y=1000.0) -> (x*y=w402:dbl)
                    n201 = Multiply(x=w402, y=2.0) -> (x*y=w401:dbl)
                    n202 = Less?(x=w400, y=w401) -> (x < y?=w407:bool)
                    n203 = Select(t=u32 6618880, s=w407, f=u32 16711680) -> (s? t:f=w411:u32)
                    n204 = Select(t="Good", s=w407, f="#s/Fs: too small!") -> (s? t:f=→"Sampling Status":string)
                    n205 = property on="Sampling Status" class="Str"("Text.BGColor"=w411) -> ()  [unwired: 2 in, 2 out]
                  }
                  frame Disabled {
                  }
                }
                n206 = call <vilib>:"Add State(s) to Queue__jki_lib_state_machine.vi"("State(s) in (\"\")"=w399) -> ("States Out"=w398:string)  [unwired: 14 in]
              }
              event User Event {
                # "#done"
                n207 = event-data() -> ("get AO"=w421:T67)  [unwired: 1 in, 4 out]
                n208 = Unbundle By Name(w423) -> ("Lockin"=w422:refnum<class "Instrument.Lockin.lvclass">)
                n209 = call <userlib>:"Write AO WFM.vi"("error in (no error)"=w420, "AO WFM"=w421, "Instrument.Lockin in"=w422) -> ("error out"=w419:errorcluster, "Instrument.Lockin out"=w418:refnum<class "Instrument.Lockin.lvclass">)  [unwired: 7 in]
                n210 = Bundle By Name(cluster=w423, "Lockin"=w418) -> (w424:T44)
                n211 = call <vilib>:"Add State(s) to Queue__jki_lib_state_machine.vi"("State(s) in Front (\"\")"="" ("State(s) in Front (\"\")"), "State(s) in (\"\")"=w427) -> ("States Out"=w426:string)  [unwired: 13 in]
              }
              event "Allowed remote system": Value Change {
                # "#done\n(not used)"
                n212 = event-data() -> ()  [unwired: 1 in, 6 out]
                n213 = call <vilib>:"Add State(s) to Queue__jki_lib_state_machine.vi"("State(s) in Front (\"\")"="DONE: AllowedRemote" ("State(s) in Front (\"\")"), "State(s) in (\"\")"=w429) -> ("States Out"=w430:string)  [unwired: 13 in]
              }
              event User Event {
                # "#done\n(obsolete)"
                # "Disable: I think this could cause an infinite loop when trying to exit"
                n214 = event-data() -> ("SMO State"=w434:T10)  [unwired: 1 in]
                "RC SMO State" <- w434
                n215 = case shown="\"Started\"" w434 {
                  tunnel: ["" ("State Queue") "//DONE: Stop Remote\n//DONE: Start Remote" ("State Queue")] -> w435
                  frame "Started" {
                  }
                  frame Default {
                  }
                }
                n216 = call <vilib>:"Add State(s) to Queue__jki_lib_state_machine.vi"("State(s) in Front (\"\")"=w435, "State(s) in (\"\")"=w437) -> ("States Out"=w436:string)  [unwired: 13 in]
              }
              event User Event {
                # "#done"
                n217 = event-data() -> ("SMO State"=w442:T10)  [unwired: 1 in]
                "LockinDAQ SMO State" <- w442
                n218 = case shown="Default" w442 {
                  tunnel: ["DONE: Enable Buttons" ("State Queue") "DONE: Stop\nDONE: Start" ("State Queue")] -> w443
                  frame "Started" {
                  }
                  frame Default {
                  }
                }
                n219 = call <vilib>:"Add State(s) to Queue__jki_lib_state_machine.vi"("State(s) in Front (\"\")"=w443, "State(s) in (\"\")"=w445) -> ("States Out"=w444:string)  [unwired: 13 in]
              }
              event User Event {
                # "#done\n(obsolete)"
                # "#todo: future: call Command: Handle Command"
                # "Message sent by the RemoteControl.lvclass:process"
                n220 = event-data() -> ("Message"=w456:T43, "Message.Command"=w453:string)  [unwired: 1 in, 4 out]
                n221 = Bundle By Name(cluster=w458, "Message"=w456) -> (w457:T44)
                n222 = Concatenate Strings("Command: ", w453) -> (w451:string)
                n223 = call <vilib>:"Add State(s) to Queue__jki_lib_state_machine.vi"("State(s) in Front (\"\")"=w451, "State(s) at Back (\"\")"="DONE: Reply to Command") -> ("States Out"=w450:string)  [unwired: 13 in]
                n224 = call <vilib>:"Add State(s) to Queue__jki_lib_state_machine.vi"("State(s) in Front (\"\")"=w450, "State(s) in (\"\")"=w455) -> ("States Out"=w454:string)  [unwired: 13 in]
              }
              event "Line", "Lowpass", "LP f (Hz)": Value Change {
                # "#done"
                n225 = event-data() -> ()  [unwired: 1 in, 6 out]
                n226 = Unbundle By Name(w466) -> ("Lockin"=w465:refnum<class "Instrument.Lockin.lvclass">)
                n227 = Bundle By Name(cluster=w465, "60 Hz"="Line", "Low Pass"="Lowpass", "Low Pass Cutoff (Hz)"="LP f (Hz)") -> (w464:refnum<class "Instrument.Lockin.lvclass">)
                n228 = Bundle By Name(cluster=w466, "Lockin"=w464) -> (w467:T44)
                n229 = call <vilib>:"Add State(s) to Queue__jki_lib_state_machine.vi"("State(s) in Front (\"\")"="DONE: Write CONFIG\nDONE: Set Prefilter" ("State(s) in Front (\"\")"), "State(s) in (\"\")"=w470) -> ("States Out"=w469:string)  [unwired: 13 in]
              }
              event User Event {
                # "#done"
                n230 = event-data() -> ("state"=w471:T68)  [unwired: 1 in, 4 out]
                n231 = case shown="\"sweeping\"" w471 {
                  frame Default {
                  }
                  frame "sweeping" {
                    n232 = call <userlib>:"MGI Milliseconds Since Last Reset.vi"("Reset (F)"=TRUE) -> ()  [unwired: 5 in, 2 out]
                  }
                }
                n233 = Bundle By Name(cluster=w473, "DAQ state"=w471) -> (w474:T44)
                n234 = call <vilib>:"Add State(s) to Queue__jki_lib_state_machine.vi"("State(s) in Front (\"\")"="DONE: Update Status" ("State(s) in Front (\"\")"), "State(s) in (\"\")"=w477) -> ("States Out"=w476:string)  [unwired: 13 in]
              }
              event "X Axis": Value Change {
                # "#done"
                # "X Axis, Y Axis Out Value Change (pressed) Event\ncall: UI: Update Waveform Graph Labels"
                n235 = event-data() -> ()  [unwired: 1 in, 6 out]
                n236 = call <vilib>:"Add State(s) to Queue__jki_lib_state_machine.vi"("State(s) in Front (\"\")"="done: Update Waveform Graph Labels" ("State(s) in Front (\"\")"), "State(s) in (\"\")"=w482) -> ("States Out"=w483:string)  [unwired: 13 in]
              }
              event "Y Axis (Output)": Value Change {
                # "#done"
                # "X Axis, Y Axis Out Value Change (pressed) Event\ncall: UI: Update Waveform Graph Labels"
                n237 = event-data() -> ()  [unwired: 1 in, 6 out]
                n238 = call <vilib>:"Add State(s) to Queue__jki_lib_state_machine.vi"("State(s) in Front (\"\")"="TODO: Update Plot Names" ("State(s) in Front (\"\")"), "State(s) in (\"\")"=w487) -> ("States Out"=w488:string)  [unwired: 13 in]
              }
              event "XY Axis Range", "X/R Range", "Y/Theta Range": Value Change {
                # "#done"
                # "X&Y Axis Range\", \"XorR Axis Range\", \"YorTheta Axis Range\" Value Change (pressed) Event\ncall: UI: Update Lockin Graph Range"
                n239 = event-data() -> ()  [unwired: 1 in, 6 out]
                n240 = call <vilib>:"Add State(s) to Queue__jki_lib_state_machine.vi"("State(s) in Front (\"\")"="DONE: Update Lockin Graph Range" ("State(s) in Front (\"\")"), "State(s) in (\"\")"=w492) -> ("States Out"=w493:string)  [unwired: 13 in]
              }
              event "Display": Value Change {
                # "#done"
                # "Display Value Change Value Change (pressed) Event\ncall:\nUI: Update Displays"
                n241 = event-data() -> ()  [unwired: 1 in, 6 out]
                n242 = call <vilib>:"Add State(s) to Queue__jki_lib_state_machine.vi"("State(s) in Front (\"\")"="DONE: Update Displays" ("f"), "State(s) in (\"\")"=w497) -> ("States Out"=w498:string)  [unwired: 13 in]
              }
              event "Reset Phase": Value Change {
                # "#done"
                # "Measure Offset Button Value Change (pressed) Event\n1. send \"measure offset\" command to DAQ"
                n243 = event-data() -> ()  [unwired: 1 in, 1 out]
                n244 = local write "Reset Phase"(FALSE ("Measure\nOffset")) -> ()
                n245 = call <vilib>:"Add State(s) to Queue__jki_lib_state_machine.vi"("State(s) in Front (\"\")"="DONE: Reset Phase" ("State(s) in Front (\"\")")) -> ("States Out"=w501:string)  [unwired: 14 in]
                n246 = call <vilib>:"Add State(s) to Queue__jki_lib_state_machine.vi"("State(s) in Front (\"\")"=w501, "State(s) in (\"\")"=w505) -> ("States Out"=w504:string)  [unwired: 13 in]
              }
              event "auto DAQ": Value Change {
                # "#done"
                # "Measure Offset Button Value Change (pressed) Event\n1. send \"measure offset\" command to DAQ"
                n247 = event-data() -> ()  [unwired: 1 in, 1 out]
                n248 = local write "auto DAQ"(FALSE ("Measure\nOffset")) -> ()
                n249 = call <vilib>:"Add State(s) to Queue__jki_lib_state_machine.vi"("State(s) in Front (\"\")"="DONE: Auto DAQ" ("State(s) in Front (\"\")")) -> ("States Out"=w508:string)  [unwired: 14 in]
                n250 = call <vilib>:"Add State(s) to Queue__jki_lib_state_machine.vi"("State(s) in Front (\"\")"=w508, "State(s) in (\"\")"=w512) -> ("States Out"=w511:string)  [unwired: 13 in]
              }
              event "Measure": Value Change {
                # "#done"
                # "Measure Offset Button Value Change (pressed) Event\n1. send \"measure offset\" command to DAQ"
                n251 = event-data() -> ()  [unwired: 1 in, 1 out]
                n252 = local write "Measure"(FALSE ("Measure\nOffset")) -> ()
                n253 = call <vilib>:"Add State(s) to Queue__jki_lib_state_machine.vi"("State(s) in Front (\"\")"="DONE: Measure Offset" ("State(s) in Front (\"\")")) -> ("States Out"=w515:string)  [unwired: 14 in]
                n254 = call <vilib>:"Add State(s) to Queue__jki_lib_state_machine.vi"("State(s) in Front (\"\")"=w515, "State(s) in (\"\")"=w519) -> ("States Out"=w518:string)  [unwired: 13 in]
              }
              event "Remove": Value Change {
                # "#done"
                # "Zero Offset Button Value Change (pressed) Event\n1. send \"zero offset\" command to DAQ"
                n255 = event-data() -> ()  [unwired: 1 in, 1 out]
                n256 = local write "Remove"(FALSE ("Zero\nOffset")) -> ()
                n257 = call <vilib>:"Add State(s) to Queue__jki_lib_state_machine.vi"("State(s) in Front (\"\")"="DONE: Remove Offset" ("State(s) in Front (\"\")")) -> ("States Out"=w522:string)  [unwired: 14 in]
                n258 = call <vilib>:"Add State(s) to Queue__jki_lib_state_machine.vi"("State(s) in Front (\"\")"=w522, "State(s) in (\"\")"=w526) -> ("States Out"=w525:string)  [unwired: 13 in]
              }
              event "Close": Value Change {
                w527 = "Macro: Exit"
                # "#done"
                # "Stop Button Value Change (pressed) Event\n(this executes Macro: Exit to terminate the VI)"
                n259 = event-data() -> ("OldVal"=w528:bool)  [unwired: 1 in]
                n260 = local write "Close"(w528) -> ()
                n261 = disable-structure shown="Disabled" {
                  disable-tunnel: w527 -> [w533 _]
                  frame Disabled {
                    n262 = Two Button Dialog(message="Are you sure you want to exit?") -> (T button?=w535:bool)  [unwired: 2 in]
                    n263 = Select(t=w533, s=w535, f="") -> ()  [unwired: 1 out]
                  }
                  frame Enabled {
                  }
                }
                n264 = call <vilib>:"Add State(s) to Queue__jki_lib_state_machine.vi"("State(s) in Front (\"\")"=w527, "State(s) in (\"\")"=w532) -> ("States Out"=w531:string)  [unwired: 13 in]
              }
              event "Start Sweep": Value Change {
                # "#done"
                # "New Start Button Value Change (pressed) Event"
                n265 = event-data() -> ()  [unwired: 1 in, 1 out]
                n266 = Unbundle By Name(w543) -> ("Lockin.DAQ"=w541:refnum<class "Instrument.DAQ.lvclass">)
                n267 = Bundle By Name(cluster=T17 {"Sweep Time (s)"=0.0, "Initial Wait (s)"=0.0, "Return to Start"=FALSE, "Channels"=[]} ("setSweep"), "Channels"="Sweep Channels", "Sweep Time (s)"="Sweep Time (s)", "Initial Wait (s)"="Initial Wait (s)", "Return to Start"="Return to Start?") -> (w538:T17)
                n268 = call "DAQ.setSweep.vi"("error in (no error)"=w550, "setSweep"=w538, "Instrument.DAQ"=w541) -> ("error out"=w540:errorcluster)  [unwired: 7 in, 1 out]
                n269 = Format Into String(T15."start sweep" ("State")) -> (resulting string=w549:string)  [unwired: 3 in, 1 out]
                n270 = call <vilib>:"Build State String with Arguments__JKI_lib_State_Machine.vi"("Arguments (\"\")"=w549, "State"="DONE: Set State" ("f")) -> ("State with Arguments"=w546:string)  [unwired: 4 in]
                n271 = call <vilib>:"Add State(s) to Queue__jki_lib_state_machine.vi"("State(s) in Front (\"\")"=w546, "State(s) in (\"\")"=w552) -> ("States Out"=w551:string)  [unwired: 13 in]
              }
              event "Stop Sweep": Value Change {
                # "New Start Button Value Change (pressed) Event"
                n272 = event-data() -> ()  [unwired: 1 in, 6 out]
                n273 = local write "Stop Sweep"(FALSE ("Sweep Start")) -> ()
                n274 = Format Into String(T15."stop sweep" ("State")) -> (resulting string=w556:string)  [unwired: 3 in, 1 out]
                n275 = call <vilib>:"Build State String with Arguments__JKI_lib_State_Machine.vi"("Arguments (\"\")"=w556, "State"="DONE: Set State" ("f")) -> ("State with Arguments"=w553:string)  [unwired: 4 in]
                n276 = call <vilib>:"Add State(s) to Queue__jki_lib_state_machine.vi"("State(s) in Front (\"\")"=w553, "State(s) in (\"\")"=w561) -> ("States Out"=w560:string)  [unwired: 13 in]
              }
              event "Load Configuration": Value Change {
                # "#done\n(not used)"
                # "LOAD CONFIG Button Value Change (pressed) Event"
                n277 = event-data() -> ("NewVal"=w566:bool)  [unwired: 1 in, 1 out]
                n278 = local write "Load Configuration"(FALSE ("load config")) -> ()
                n279 = Select(t="DONE: Read CONFIG" ("State(s) at Back (\"\")"), s=w566, f="") -> (s? t:f=w563:string)
                n280 = call <vilib>:"Add State(s) to Queue__jki_lib_state_machine.vi"("State(s) in Front (\"\")"=w563, "State(s) in (\"\")"=w570) -> ("States Out"=w569:string)  [unwired: 13 in]
              }
              event "Save Configuration": Value Change {
                # "#done\n(not used)"
                # "save config Button Value Change (pressed) Event"
                n281 = event-data() -> ("NewVal"=w573:bool)  [unwired: 1 in]
                n282 = local write "Save Configuration"(FALSE ("save config")) -> ()
                n283 = Select(t="DONE: Write CONFIG" ("State(s) at Back (\"\")"), s=w573, f="") -> (s? t:f=w574:string)
                n284 = call <vilib>:"Add State(s) to Queue__jki_lib_state_machine.vi"("State(s) in Front (\"\")"=w574, "State(s) in (\"\")"=w579) -> ("States Out"=w578:string)  [unwired: 13 in]
              }
              event "Save": Value Change {
                # "#done \n(not used)"
                # "Save Mode Button Value Change (pressed) Event"
                n285 = event-data() -> ("OldVal"=w580:bool)  [unwired: 1 in]
                n286 = local write "Save"(w580) -> ()
                n287 = call <vilib>:"Add State(s) to Queue__jki_lib_state_machine.vi"("State(s) in (\"\")"=w585, "State(s) at Back (\"\")"="done: SAVE") -> ("States Out"=w584:string)  [unwired: 13 in]
              }
              event "Help": Value Change {
                # "#done"
                # "Help Button Value Change (pressed) Event\nIf Help = True: Send user to help webpage; Set Help=False\nIf Help=Fale, Do nothing"
                n288 = event-data() -> ("NewVal"=w586:bool)  [unwired: 1 in]
                n289 = case shown="True" w586 {
                  tunnel: w588 -> [w592 w596]
                  tunnel: [w592 w594] -> w587
                  frame False {
                  }
                  frame True {
                    n290 = local write "Help"(FALSE ("Help")) -> ()
                    n291 = call-poly <vilib>:"Open URL in Default Browser.vi"("error in (no error)"=w596, "URL"="https://app.asana.com/0/205665857037275/list") -> ("error out"=w594:errorcluster)  [unwired: 4 in, 1 out]
                  }
                }
                n292 = call <vilib>:"Add State(s) to Queue__jki_lib_state_machine.vi"("State(s) in (\"\")"=w591) -> ("States Out"=w590:string)  [unwired: 14 in]
              }
              event Panel Close? {
                w597 = "Macro: Exit"
                # "Discard the event because we'll close the front panel ourselves in Macro: Exit"
                # "Close Panel button (pressed) Event\n(this executes Macro: Exit to terminate the VI)"
                n293 = event-data() -> ()  [unwired: 1 in, 1 out]
                n294 = disable-structure shown="Disabled" {
                  disable-tunnel: w597 -> [w603 _]
                  frame Disabled {
                    n295 = Two Button Dialog(message="Are you sure you want to exit?") -> (T button?=w605:bool)  [unwired: 2 in]
                    n296 = Select(t=w603, s=w605, f="") -> ()  [unwired: 1 out]
                  }
                  frame Enabled {
                  }
                }
                n297 = call <vilib>:"Add State(s) to Queue__jki_lib_state_machine.vi"("State(s) in Front (\"\")"=w597, "State(s) in (\"\")"=w598) -> ("States Out"=w602:string)  [unwired: 13 in]
                n298 = event-data("Discard?"=TRUE) -> ()  [unwired: 1 in, 1 out]
              }
            }
          }
          frame "---------- Core ----------" {
            # "Do not put any code in this frame.\n(it is a separator no-op)"
            n299 = call <vilib>:"Add State(s) to Queue__jki_lib_state_machine.vi"("State(s) in (\"\")"=w611) -> ("States Out"=w610:string)  [unwired: 14 in]
          }
          frame Default {
            w623 = 42 items=["No error", "Argument error", "Memory is full", "Out of zone", "End of file", "File already open", "Generic file I/O error", "File not found", "File permission error", "Disk is full", "Duplicate path", "Too many files open", "System feature not enabled", "Resource file not found", "Cannot add resource", "Resource not found", "Image not found", "Image memory error", "Pen does not exist", "Config type invalid", "Config token not found", "Config parse error", "Config memory error", "Bad external code format", "Bad external code offset", "External code not present", "Null window", "Destroy window error", "Null menu", "Print aborted", "Bad print record", "Print driver error", "Windows error during printing", "Memory error during printing", "Print dialog error", "Generic print error", "Invalid device refnum", "Device not found", "Device parameter error", "Device unit error", "Cannot open device", "Device call aborted", "Generic error", "Cancelled by user", "Object ID too low", "Object ID too high", "Object not in heap", "Unknown heap", "Unknown object (invalid DefProc)", "Unknown object (DefProc not in table)", "Message out of range", "Invalid (null) method", "Unknown message", "Manager call not supported", "Bad address", "Network operation in progress", "Network operation timed out", "Connection is busy", "Network attribute not supported", "Network error", "Address in use", "System out of memory", "Connection aborted", "Connection refused", "Not connected", "Already connected", "Connection closed", "Initialization error (interapplication manager)", "Bad occurrence", "Wait on unbound occurrence handler", "Occurrence queue overflow", "Datalog type conflict", "Unused", "Unrecognized type (interapplication manager)", "Memory corrupt", "Failed to make temporary DLL", "Old CIN version", "Drag socket not found", "Failed to load drop-object", "Failed to register OLE object", "Failed to release OLE object", "Format specifier type mismatch", "Unknown format specifier", "Too few format specifiers", "Too many format specifiers", "Scan failed", "Newer CIN version", "Error converting to variant", "Runtime menu error", "Password tampered", "Variant attribute not found", "Incompatible variant data type", "Event data is not available", "Event Store is not present", "Occurrence is not found", "Event Queue is not created", "Event info is not available", "Refnum passed is NULL", "Error retrieving Class GUID", "Error retrieving CoClass GUID", "Error retrieving TypeLib GUID.", "Bad built application magic bytes.", "Specific driver is different from the specific driver associated with the Logical Name.", "There is no session opened to the class driver.", "Max Error", "MAX - Error with config objects", "MAX - Error loading configuration", "MAX - Group not supported"]
            # "Current State"
            # "Do not delete, rename, or modify this frame.\n(this is used to capture unhandled states and typos)"
            # "Handle mistyped state name (developer tool)"
            n300 = Format Into String(format string="Software Exception: Unhandled State \"%s\"." ("message"), error in=w619, w614) -> (resulting string=w622:string, error out=w621:errorcluster)  [unwired: 1 in]
            n301 = call <vilib>:"Error Cluster From Error Code.vi"("show call chain? (False)"=TRUE, "error in (no error)"=w621, "error message (\"\")"=w622, "error code (0)"=w623) -> ("error out"=w620:errorcluster)  [unwired: 5 in]
            n302 = call <vilib>:"Add State(s) to Queue__jki_lib_state_machine.vi"("State(s) in (\"\")"=w618) -> ("States Out"=w617:string)  [unwired: 14 in]
          }
          frame "Initialize Core Data" {
            # "Do not delete, rename, or modify this frame.\n(this is used to determine panel behavior on exit)"
            # "originally closed?"
            # "exe?"
            # "If panel starts closed or is an EXE, then close it when we exit"
            n303 = property class="VI"() -> ("Front Panel.Open"=w632:bool)  [unwired: 2 in, 2 out]
            n304 = property class="App"() -> ("App.Kind"=w631:T18)  [unwired: 2 in, 2 out]
            n305 = control-ref of="Current VI Reference"() -> (w625:refnum<vi>)
            n306 = Not(x=w632) -> (.not. x?=w629:bool)
            n307 = Equal?(x=w631, y=T18."Run Time System" ("Application:Kind")) -> (x = y?=w628:bool)
            n308 = Or(x=w629, y=w628) -> (x .or. y?=w626:bool)
            n309 = Bundle By Name(cluster=w627, "Core.Current VI Reference"=w625, "Core.Close Panel on Exit?"=w626) -> (w634:T44)
            n310 = call <vilib>:"Add State(s) to Queue__jki_lib_state_machine.vi"("State(s) in (\"\")"=w636) -> ("States Out"=w635:string)  [unwired: 14 in]
          }
          frame "Error Handler" {
            # "Handle any errors here.\nYou can also output any states to clean-up after errors occur"
            # "Clear error"
            n311 = Unbundle By Name(w641) -> ("Lockin"=w640:refnum<class "Instrument.Lockin.lvclass">)
            n312 = call-dynamic "Handle Error.vi"("Stop on Unhandled Error (T)"=FALSE, "error in"=w638, "SMO"=w640) -> ("handling error"=w637:errorcluster)  [unwired: 6 in, 2 out]
            n313 = call-poly <userlib>:"Filter Error Codes__ogtk.vi"("Error In"=w637, "Error Codes to Filter"=i32[] [-200077, -200462, -200245, -200279]) -> ("Error Out"=w645:errorcluster)  [unwired: 7 in, 2 out]
            n314 = case shown="Error" w645 {
              selector: w645 -> [w650 w655]
              tunnel: ["" "Macro: Exit"] -> w647
              tunnel: [w650 w652] -> w643
              frame No Error {
              }
              frame Error {
                w653 = T69 1 items=["no dialog", "OK message", "continue or stop message", "OK message + warnings", "continue/stop + warnings"] ("type of dialog (OK msg:1)")
                # "Unhandled Error -- Display it"
                n315 = call <vilib>:"General Error Handler.vi"("type of dialog (OK msg:1)"=w653, "error in (no error)"=w655) -> ("error out"=w652:errorcluster)  [unwired: 9 in, 4 out]
              }
            }
            n316 = call <userlib>:"Clear All Errors__ogtk.vi"("Error In"=w643) -> ("Error Out"=w642:errorcluster)  [unwired: 3 in]
            n317 = call <vilib>:"Add State(s) to Queue__jki_lib_state_machine.vi"("State(s) in Front (\"\")"=w647, "State(s) in (\"\")"=w649) -> ("States Out"=w648:string)  [unwired: 13 in]
          }
          frame "Exit" {
            # "Do not put any code in this frame.\n(No errors that occur here will be handled.)"
            n318 = call <vilib>:"Add State(s) to Queue__jki_lib_state_machine.vi"("State(s) in (\"\")"=w661) -> ("States Out"=w660:string)  [unwired: 14 in]
          }
          frame "---------- Data ----------" {
            # "Do not put any code in this frame.\n(It is a separator no-op. You can make a copy of this frame to create a new Data frame)"
            n319 = call <vilib>:"Add State(s) to Queue__jki_lib_state_machine.vi"("State(s) in (\"\")"=w666) -> ("States Out"=w665:string)  [unwired: 14 in]
          }
          frame "Data: Initialize" {
            w667 = refnum<class "Instrument.DAQ.lvclass"> refnum  # Lockin.DAQ
            w669 = refnum<class "Logger.Error.lvclass"> refnum  # Logger.Error
            w675 = T70 {"Sweep_AO"=[], "Sweep_AI"=[]}  # SweepWaveforms
            w668 = T71 {"X results"=[], "Y Results"=[]}  # SweepResults
            w672 = T45."idle"  # DAQ state
            w677 = T42 {"address"="", "Port"=0, "AllowedRemote"="", "Commands"=[], "timeout"=0}  # RemoteControl.Configure
            (unwired) T72 {"Time Stamp"=timestamp(0 s since 1904-01-01), "Results (Dictionary)"=[]}  # Results
            w678 = T43 {"Command"="", "Data"=variant, "ID"=""}  # HandledMessage
            w679 = T43 {"Command"="", "Data"=variant, "ID"=""}  # Message
            w671 = refnum<class "Instrument.Lockin.lvclass"> refnum  # Lockin
            w670 = refnum<class "RemoteControl.lvclass"> refnum  # RemoteControl
            (unwired) waveform(dbl)[] []  # AI WFM
            w673 = 100  # to
            (unwired) waveform(dbl)[] []  # AO WFM
            (unwired) waveform(dbl)[] []  # REF WFM
            w681 = T73 {"Current VI Reference"=refnum, "Close Panel on Exit?"=FALSE}  # Core
            # "is sent to RC:process"
            # "comes from RC:process"
            # "do not delete - used by framework"
            # "Initialize the shift-register data, here.\n(data names are defined by what you wire into the bundle function)"
            n320 = call <vilib>:"Add State(s) to Queue__jki_lib_state_machine.vi"("State(s) in (\"\")"=w683) -> ("States Out"=w682:string)  [unwired: 14 in]
            n321 = Bundle("Core"=w681, "to"=w673, "Lockin"=w671, "RemoteControl"=w670, "Lockin.DAQ"=w667, "Logger.Error"=w669, "DAQ state"=w672, "RemoteControl.Configure"=w677, "Message"=w679, "HandledMessage"=w678, "SweepResults"=w668, "SweepWaveforms"=w675) -> (w676:T44)  [unwired: 1 in]
          }
          frame "Data: Cleanup" {
            # "Cleanup any data and references, here.\n(this is called automatically, by the Macro: Exit)"
            n322 = Unbundle By Name(w685) -> ("Core.Current VI Reference"=w687:refnum<vi>)
            n323 = Close Reference(reference=w687, error in (no error)=w686) -> (error out=w684:errorcluster)
            n324 = call <vilib>:"Add State(s) to Queue__jki_lib_state_machine.vi"("State(s) in (\"\")"=w690) -> ("States Out"=w689:string)  [unwired: 14 in]
          }
          frame "---------- Events ----------" {
            # "Template Separator\n(You can make a copy of, or modify, this frame)"
            n325 = call <vilib>:"Add State(s) to Queue__jki_lib_state_machine.vi"("State(s) in (\"\")"=w695) -> ("States Out"=w694:string)  [unwired: 14 in]
          }
          frame "Events: Register" {
            w704 = T74 {"Error"=refnum, "State"=refnum, "Reserve State"=refnum}  # LockinDAQ SMO Public Events
            w713 = T74 {"Error"=refnum, "State"=refnum, "Reserve State"=refnum}  # RC SMO Public Events
            n326 = Unbundle By Name(w717) -> ("RemoteControl"=w709:refnum<class "RemoteControl.lvclass">, "Lockin.DAQ"=w696:refnum<class "Instrument.DAQ.lvclass">)
            n327 = call <vilib>:"GetPublicEvents.vi"("SMO"=w709) -> ("error out"=w708:errorcluster, "Public Events"=w712:T74, "SMO out"=w706:refnum<class "RemoteControl.lvclass">)  [unwired: 8 in]
            n328 = Variant To Data(error in=w708, type=w713, Variant=w712) -> (data=w711:T74, error out=w707:errorcluster)
            n329 = call <vilib>:"GetPublicEvents.vi"("SMO"=w696) -> ("error out"=w701:errorcluster, "Public Events"=w703:T74, "SMO out"=w699:refnum<class "Instrument.DAQ.lvclass">)  [unwired: 8 in]
            n330 = call <userlib>:"RemoteControl.GetPublicEvents.vi"("RemoteControl"=w706) -> ("error out"=w705:errorcluster, "RC Public Events"=w716:T75)  [unwired: 8 in, 1 out]
            n331 = Variant To Data(error in=w701, type=w704, Variant=w703) -> (data=w702:T74, error out=w700:errorcluster)
            n332 = call <userlib>:"Lockin.DAQ.GetPublicEvents.vi"("Lockin.DAQ"=w699) -> ("error out"=w714:errorcluster, "LIADAQ Public Events"=w710:T76)  [unwired: 8 in, 1 out]
            n333 = register-events(w711, w716, w702, w710) -> (reference out=w718:refnum<event-registration>, error out=w715:errorcluster)  [unwired: 2 in]
            n334 = Merge Errors(w715, w714, w705, w700, w707, w697) -> (w698:errorcluster)
            n335 = call <vilib>:"Add State(s) to Queue__jki_lib_state_machine.vi"("State(s) in (\"\")"=w720) -> ("States Out"=w719:string)  [unwired: 14 in]
          }
          frame "Events: Unregister" {
            n336 = Unregister For Events(event registration refnum=w722, error in=w721) -> (error out=w723:errorcluster)
            n337 = call <vilib>:"Clear Errors.vi"("error in (no error)"=w723) -> ()  [unwired: 5 in, 2 out]
            n338 = call <vilib>:"Add State(s) to Queue__jki_lib_state_machine.vi"("State(s) in (\"\")"=w726) -> ("States Out"=w725:string)  [unwired: 14 in]
          }
          frame "---------- Macro ----------" {
            # "Do not put any code in this frame.\n(It is a separator no-op. You can make a copy of this frame to create a new Macro frame)"
            n339 = call <vilib>:"Add State(s) to Queue__jki_lib_state_machine.vi"("State(s) in (\"\")"=w731) -> ("States Out"=w730:string)  [unwired: 14 in]
          }
          frame "Macro: Initialize" {
            n340 = call <vilib>:"Add State(s) to Queue__jki_lib_state_machine.vi"("State(s) in Front (\"\")"="Data: Initialize\nInitialize Core Data\n\nDONE: Initialize\n\nDONE: Create Remote\nDONE: Create\nEvents: Register\nDONE: Start Remote\nDONE: Start\n\nDONE: Create\n\nUI: Front Panel State >> Open\n\nDONE: Initialize CONFIG\nDONE: Read CONFIG\n\nMacro: Initialize UI\nDONE: Update Sweep WFMs Graphs\nDONE: Disable Buttons\n\nDONE: AllowedRemote\n\nMacro: Initialize DAQ SMO", "State(s) in (\"\")"=w732) -> ("States Out"=w737:string)  [unwired: 13 in]
          }
          frame "Macro: Initialize UI" {
            n341 = call <vilib>:"Add State(s) to Queue__jki_lib_state_machine.vi"("State(s) in Front (\"\")"="DONE: Initialize REF Ch\nDONE: Initialize AO Ch\nDONE: Initialize Gains\nDONE: Initialize AI Ch\nTODO: Update Plot Names\ndone: Update Waveform Graph Labels\nDONE: Update Displays" ("State(s) in Front (\"\")"), "State(s) in (\"\")"=w743) -> ("States Out"=w742:string)  [unwired: 13 in]
          }
          frame "Macro: Initialize DAQ SMO" {
            # "#todo"
            n342 = Unbundle By Name(w745) -> ("Lockin.DAQ"=w748:refnum<class "Instrument.DAQ.lvclass">)
            n343 = while {
              tunnel: [w763] -> w746
              tunnel: w748 -> [w762]
              tunnel: w747 -> [w761]
              tunnel: [w759] -> w744
              i -> [w756]
              stop <- w753 stop-if-true
              n344 = call <vilib>:"GetState.vi"("error in (no error)"=w761, "SMO"=w762) -> ("error out"=w760:errorcluster, "SMO State"=w758:T10)  [unwired: 7 in, 1 out]
              n345 = case shown="\"Started\"" w758 {
                tunnel: ["" "DONE: Set AI Config\nDONE: Set AO Config\nDONE: Set AI\nDONE: Set AO\nDONE: Set REF\nDONE: Set Input Gain\nDONE: Set Output Gain\nMacro: Update Sampling\n//TODO: Set Sampling"] -> w763
                tunnel: w760 -> [w765 w768]
                tunnel: [w764 w768] -> w759
                frame Default {
                  n346 = call <userlib>:"Wait (ms)__ogtk.vi"("error in (no error)"=w765, "milliseconds to wait"=u32 100) -> ("error out"=w764:errorcluster)  [unwired: 8 in, 1 out]
                }
                frame "Started" {
                }
              }
              n347 = Equal?(x=w758, y=SMOState_--Enum."Started") -> (x = y?=w754:bool)
              n348 = Greater?(x=w756, y=10) -> (0:w752:bool)
              n349 = Or(x=w754, y=w752) -> (x .or. y?=w753:bool)
            }
            n350 = call <vilib>:"Add State(s) to Queue__jki_lib_state_machine.vi"("State(s) in Front (\"\")"=w746, "State(s) in (\"\")"=w751) -> ("States Out"=w750:string)  [unwired: 13 in]
          }
          frame "Macro: Reset DAQ SMO" {
            # "#todo"
            n351 = Unbundle By Name(w771) -> ("Lockin.DAQ"=w774:refnum<class "Instrument.DAQ.lvclass">)
            n352 = while {
              tunnel: [w789] -> w772
              tunnel: w774 -> [w788]
              tunnel: w773 -> [w787]
              tunnel: [w785] -> w770
              i -> [w782]
              stop <- w779 stop-if-true
              n353 = call <vilib>:"GetState.vi"("error in (no error)"=w787, "SMO"=w788) -> ("error out"=w786:errorcluster, "SMO State"=w784:T10)  [unwired: 7 in, 1 out]
              n354 = case shown="\"Started\"" w784 {
                tunnel: ["" "DONE: Set AI Config\nDONE: Set AO Config\nDONE: Set AI\nDONE: Set AO\nDONE: Set REF\nDONE: Set Input Gain\nDONE: Set Output Gain\nMacro: Update Sampling\n//TODO: Set Sampling"] -> w789
                tunnel: w786 -> [w791 w794]
                tunnel: [w790 w794] -> w785
                frame Default {
                  n355 = call <userlib>:"Wait (ms)__ogtk.vi"("error in (no error)"=w791, "milliseconds to wait"=u32 100) -> ("error out"=w790:errorcluster)  [unwired: 8 in, 1 out]
                }
                frame "Started" {
                }
              }
              n356 = Equal?(x=w784, y=SMOState_--Enum."Started") -> (x = y?=w780:bool)
              n357 = Greater?(x=w782, y=10) -> (0:w778:bool)
              n358 = Or(x=w780, y=w778) -> (x .or. y?=w779:bool)
            }
            n359 = call <vilib>:"Add State(s) to Queue__jki_lib_state_machine.vi"("State(s) in Front (\"\")"=w772, "State(s) in (\"\")"=w777) -> ("States Out"=w776:string)  [unwired: 13 in]
          }
          frame "Macro: Update Sampling" {
            w809 = 10123 items=["Finite Samples"=10178, "Continuous Samples"=10123] ("Sample Mode")
            w808 = 10178 items=["Finite Samples"=10178, "Continuous Samples"=10123] ("Sample Mode")
            # "Do not put any code in this frame.\n(It is a separator no-op. You can make a copy of this frame to create a new Macro frame)"
            n360 = Unbundle By Name(w798) -> ("DAQ state"=w799:T45)
            n361 = case shown="\"created\", Default" w799 {
              tunnel: ["" ("State with Arguments") w816] -> w805
              frame "idle" {
              }
              frame "created", Default {
                n362 = Format Into String(T15."stop" ("State")) -> (resulting string=w819:string)  [unwired: 3 in, 1 out]
                n363 = call <vilib>:"Build State String with Arguments__JKI_lib_State_Machine.vi"("Arguments (\"\")"=w819, "State"="DONE: Set State" ("f")) -> ("State with Arguments"=w816:string)  [unwired: 4 in]
              }
            }
            n364 = local read "Start"() -> (w796:bool)
            n365 = case shown="\"created\", Default" w799 {
              tunnel: ["" ("State with Arguments") w821] -> w803
              frame "idle" {
              }
              frame "created", Default {
                n366 = Format Into String(T15."start" ("State")) -> (resulting string=w822:string)  [unwired: 3 in, 1 out]
                n367 = call <vilib>:"Build State String with Arguments__JKI_lib_State_Machine.vi"("Arguments (\"\")"=w822, "State"="DONE: Set State" ("f")) -> ("State with Arguments"=w821:string)  [unwired: 4 in]
              }
            }
            n368 = Select(t=w809, s=w796, f=w808) -> (s? t:f=w807:i32)
            n369 = Format Into String(w807) -> (resulting string=w806:string)  [unwired: 3 in, 1 out]
            n370 = call <vilib>:"Build State String with Arguments__JKI_lib_State_Machine.vi"("Arguments (\"\")"=w806, "State"="TODO: Set Sampling") -> ("State with Arguments"=w804:string)  [unwired: 4 in]
            n371 = call <vilib>:"Add State(s) to Queue__jki_lib_state_machine.vi"("State(s) in Front (\"\")"=w805, "State(s) in (\"\")"=w804, "State(s) at Back (\"\")"=w803) -> ("States Out"=w797:string)  [unwired: 12 in]
            n372 = call <vilib>:"Add State(s) to Queue__jki_lib_state_machine.vi"("State(s) in Front (\"\")"="4461: SAMPLING SETUP" ("State(s) in Front (\"\")"), "State(s) in (\"\")"="DONE: Write CONFIG" ("State(s) in Front (\"\")"), "State(s) at Back (\"\")"=w797) -> ("States Out"=w800:string)  [unwired: 12 in]
            n373 = call <vilib>:"Add State(s) to Queue__jki_lib_state_machine.vi"("State(s) in Front (\"\")"=w800, "State(s) in (\"\")"=w814) -> ("States Out"=w813:string)  [unwired: 13 in]
          }
          frame "Macro: Exit" {
            # "Exit Macro\n(This is called once, when the VI exits)"
            n374 = Unbundle By Name(w829) -> ("Core.Close Panel on Exit?"=w833:bool)
            n375 = Select(t="UI: Front Panel State >> Close", s=w833, f="") -> (s? t:f=w832:string)
            n376 = call <vilib>:"Add State(s) to Queue__jki_lib_state_machine.vi"("State(s) in Front (\"\")"="TODO: Set AO Zero Amplitude\nDONE: Stop Remote\nDONE: Stop\nDONE: Stop\nDONE: Write CONFIG\nDONE: Disable Buttons\nUI: Cleanup", "State(s) in (\"\")"=w832, "State(s) at Back (\"\")"="Events: Unregister\nData: Cleanup\nExit") -> ("States Out"=w830:string)  [unwired: 12 in]
            n377 = call <vilib>:"Add State(s) to Queue__jki_lib_state_machine.vi"("State(s) in Front (\"\")"=w830, "State(s) in (\"\")"=w836) -> ("States Out"=w835:string)  [unwired: 13 in]
          }
          frame "---------- UI ----------" {
            # "Do not put any code in this frame.\n(It is a separator no-op. You can make a copy of this frame to create a new UI frame)"
            n378 = call <vilib>:"Add State(s) to Queue__jki_lib_state_machine.vi"("State(s) in (\"\")"=w841) -> ("States Out"=w840:string)  [unwired: 14 in]
          }
          frame "UI: Update AI Reference Channels" {
            # "#done\nin UI or lockin or DAQ?"
            # "Add or remove AI channels"
            n379 = Unbundle By Name(w850) -> ("Lockin"=w847:refnum<class "Instrument.Lockin.lvclass">)
            n380 = case shown="\"All 1\"" w842 {
              tunnel: [u16[] [1] ("References") u16[] [0] ("References")] -> w843
              frame "All 1" {
              }
              frame "Disable", Default {
              }
            }
            n381 = Unbundle By Name(w847) -> ("AI"=w848:T77)
            n382 = for {
              tunnel: w848 -> [w859] mode=indexing
              tunnel: [w858] -> w846 mode=indexing
              tunnel: w843 -> [w857]
              n383 = Bundle By Name(cluster=w859, "References"=w857) -> (w858:T78)
            }
            n384 = Bundle By Name(cluster=w847, "AI"=w846) -> (w845:refnum<class "Instrument.Lockin.lvclass">)
            n385 = property on="AI Channels" class="Arr (strict)"(error in=w844, "Val(Sgnl)"=w846) -> (error out=w849:errorcluster)  [unwired: 1 in, 1 out]
            n386 = Bundle By Name(cluster=w850, "Lockin"=w845) -> (w851:T44)
            n387 = call <vilib>:"Add State(s) to Queue__jki_lib_state_machine.vi"("State(s) in (\"\")"=w854) -> ("States Out"=w853:string)  [unwired: 14 in]
          }
          frame "UI: Initialize Gains" {
            # "#todo\nfigure out where to call"
            # "#todo\nfigure out where to call"
            n388 = Unbundle By Name(w870) -> ("Lockin"=w869:refnum<class "Instrument.Lockin.lvclass">)
            n389 = call "Initialize Input Gain.vi"("error in (no error)"=w868, "Instrument.DAQ"=w869) -> ("error out"=w866:errorcluster, "Input Gain"=w864:T40, "Instrument.DAQ out"=w867:refnum<class "Instrument.DAQ.lvclass">)  [unwired: 7 in]
            n390 = property on="Input Gain" class="Arr (strict)"(error in=w866, "Val(Sgnl)"=w864) -> (error out=w865:errorcluster)  [unwired: 1 in, 1 out]
            n391 = call "Initialize Ouput Gain.vi"("error in (no error)"=w865, "Instrument.DAQ"=w867) -> ("error out"=w861:errorcluster, "Output Gain"=w863:T40, "Instrument.DAQ out"=w862:refnum<class "Instrument.DAQ.lvclass">)  [unwired: 7 in]
            n392 = property on="Output Gain" class="Arr (strict)"(error in=w861, "Val(Sgnl)"=w863) -> (error out=w860:errorcluster)  [unwired: 1 in, 1 out]
            n393 = Bundle By Name(cluster=w870, "Lockin"=w862) -> (w871:T44)
            n394 = call <vilib>:"Add State(s) to Queue__jki_lib_state_machine.vi"("State(s) in (\"\")"=w874) -> ("States Out"=w873:string)  [unwired: 14 in]
          }
          frame "UI: Update Rings" {
            # "#done"
            # "#done"
            # "#done"
            # "update Ch.AI after removing\nunused Ch.REF"
            # "update AI Ref Channel ring"
            # "update Sweep Channel ring"
            n395 = call "Get AO StringsAndValues.vi"("error in (no error)"=w884) -> ("error out"=w882:errorcluster, "AO Strings and Values"=w883:cluster{string, i32}[])  [unwired: 9 in]
            n396 = disable-structure shown="Disabled" {
              frame Disabled {
                n397 = call "Get AI REF (f) StringsAndValues.vi"() -> ("error out"=w892:errorcluster, "AI REF (f) StringsAndValues"=w891:cluster{string, i32}[], 3:w890)  [unwired: 9 in]
                n398 = property on="Channel" class="Ring (strict)"(error in=w892, "StringsAndValues[]"=w891) -> ()  [unwired: 1 in, 2 out]
              }
              frame Enabled {
              }
            }
            n399 = property on="Channel" class="Ring (strict)"(error in=w882, "StringsAndValues[]"=w883) -> (error out=w880:errorcluster)  [unwired: 1 in, 1 out]
            n400 = call "Get REF StringsAndValues.vi"("error in (no error)"=w880) -> ("error out"=w881:errorcluster, "REF Strings and Values"=w879:cluster{string, i32}[])  [unwired: 9 in]
            n401 = property on="Reference" class="Ring (strict)"(error in=w881, "StringsAndValues[]"=w879) -> (error out=w877:errorcluster)  [unwired: 1 in, 1 out]
            n402 = call "Remove Unused References.vi"("error in (no error)"=w877) -> ("error out"=w876:errorcluster, "Channels.AI out"=w875:T77)  [unwired: 9 in]
            n403 = local write "AI Channels"(w875) -> ()
            n404 = Bundle By Name(cluster=w885) -> (w886:T44, "Lockin"=w878:refnum<class "Instrument.Lockin.lvclass">)
            n405 = call <vilib>:"Add State(s) to Queue__jki_lib_state_machine.vi"("State(s) in (\"\")"=w889) -> ("States Out"=w888:string)  [unwired: 14 in]
          }
          frame "UI: Cleanup" {
            w894 = FALSE ("Close")
            w893 = waveform(dbl)[] [] ("Signals Graph")
            w896 = waveform(dbl)[][] [] ("History Data")
            # "Initialize the User Interface, here.\n(this is called automatically, by the Macro: Exit)"
            n406 = property on="Lockin 1" class="WFChart (strict)"("History Data"=w896) -> ()  [unwired: 2 in, 2 out]
            n407 = local write "Sweep Results X"(w893) -> ()
            n408 = local write "Sweep Results Y"(w893) -> ()
            n409 = property on="AI Graph" class="WFGraph (strict)"("Value"=w893) -> (error out=w895:errorcluster)  [unwired: 2 in, 1 out]
            n410 = property on="Lockin 2" class="WFChart (strict)"("History Data"=w896) -> ()  [unwired: 2 in, 2 out]
            n411 = property on="AO Graph" class="WFGraph (strict)"(error in=w895, "Value"=w893) -> ()  [unwired: 1 in, 2 out]
            n412 = local write "Self Calibrate"(w894) -> ()
            n413 = local write "Trigger"(w894) -> ()
            n414 = local write "Close"(w894) -> ()
            n415 = local write "Pause"(w894) -> ()
            n416 = local write "Reset"(w894) -> ()
            n417 = local write "Start"(w894) -> ()
            n418 = local write "Status"("Shutdown" ("Status")) -> ()
            n419 = call <vilib>:"Add State(s) to Queue__jki_lib_state_machine.vi"("State(s) in (\"\")"=w902) -> ("States Out"=w901:string)  [unwired: 14 in]
          }
          frame "---------- DONE ----------" {
            n420 = call <vilib>:"Add State(s) to Queue__jki_lib_state_machine.vi"("State(s) in (\"\")"=w907) -> ("States Out"=w906:string)  [unwired: 14 in]
          }
          frame "done: Update Waveform Graph Labels" {
            # "#done"
            n421 = control-ref of="AI Graph"() -> (w916:refnum<vi>)
            n422 = control-ref of="AO Graph"() -> (w911:refnum<vi>)
            n423 = call <userlib>:"X Axis WFM Graph.vi"("error in (no error)"=w912, "X Axis"="X Axis", "WaveformGraph in"=w916) -> ("error out"=w914:errorcluster)  [unwired: 8 in]
            n424 = call <userlib>:"X Axis WFM Graph.vi"("error in (no error)"=w914, "X Axis"="X Axis", "WaveformGraph in"=w911) -> ("error out"=w913:errorcluster)  [unwired: 8 in]
            n425 = control-ref of="AO Graph"() -> (w910:refnum<vi>)
            n426 = call <userlib>:"Y Axis Output WFM Graph.vi"("error in (no error)"=w913, "Y Axis Out"="Y Axis (Output)", "WaveformGraph in"=w910) -> ("error out"=w909:errorcluster)  [unwired: 8 in]
            n427 = call <vilib>:"Add State(s) to Queue__jki_lib_state_machine.vi"("State(s) in (\"\")"=w920) -> ("States Out"=w919:string)  [unwired: 14 in]
          }
          frame "DONE: Adjust Channels" {
            # "#done\nmove to Inst.DAQ"
            # "#done\nmove to Inst.DAQ"
            # "#done"
            # "#done"
            n428 = Unbundle By Name(w925) -> ("Lockin"=w926:refnum<class "Instrument.Lockin.lvclass">)
            n429 = call "Initialize REF Channels.vi"("error in (no error)"=w927, "Instrument.DAQ"=w926) -> ("error out"=w928:errorcluster, "Instrument.DAQ out"=w929:refnum<class "Instrument.DAQ.lvclass">)  [unwired: 8 in]
            n430 = call "Initialize AO Channels.vi"("error in (no error)"=w928, "Instrument.DAQ"=w929) -> ("error out"=w933:errorcluster, "Instrument.DAQ out"=w935:refnum<class "Instrument.DAQ.lvclass">)  [unwired: 8 in]
            n431 = case shown="True" "Limit Amplitudes" {
              tunnel: w935 -> [w943 w948]
              tunnel: [w943 w947] -> w934
              tunnel: w933 -> [w942 w946]
              tunnel: [w942 w945] -> w932
              tunnel: "AO Amp Limit" -> [_ w944]
              frame False {
              }
              frame True {
                n432 = call "Limit AO Amplitude.vi"("error in (no error)"=w946, 10:w944, "Instrument.DAQ"=w948) -> ("error out"=w945:errorcluster, "Instrument.DAQ out"=w947:refnum<class "Instrument.DAQ.lvclass">)  [unwired: 7 in]
              }
            }
            n433 = case shown="True" "Link Frequencies" {
              tunnel: w934 -> [w950 w955]
              tunnel: [w950 w954] -> w930
              tunnel: w932 -> [w949 w953]
              tunnel: [w949 w952] -> w938
              tunnel: "AO freq link" -> [_ w951]
              frame False {
              }
              frame True {
                n434 = call "Set all f same.vi"("error in (no error)"=w953, 10:w951, "Instrument.DAQ"=w955) -> ("error out"=w952:errorcluster, "Instrument.DAQ out"=w954:refnum<class "Instrument.DAQ.lvclass">)  [unwired: 7 in]
              }
            }
            n435 = Unbundle By Name(w930) -> ("AO"=w937, "REF"=w936)
            n436 = Bundle By Name(cluster=w925, "Lockin"=w930) -> (w924:T44)
            n437 = local write "REF Channels"(w936) -> ()
            n438 = local write "AO Channels"(w937) -> ()
            n439 = call <vilib>:"Add State(s) to Queue__jki_lib_state_machine.vi"("State(s) in (\"\")"=w941) -> ("States Out"=w940:string)  [unwired: 14 in]
          }
          frame "DONE: Update Lockin Graph Range" {
            # "#done"
            n440 = Negate(x="XY Axis Range") -> (-x=w958:dbl)
            n441 = Negate(x="X/R Range") -> (-x=w960:dbl)
            n442 = Negate(x="Y/Theta Range") -> (-x=w961:dbl)
            n443 = property on="Lockin 1" class="WFChart (strict)"("YScale.Maximum"="X/R Range", "YScale.Minimum"=w960) -> ()  [unwired: 2 in, 2 out]
            n444 = property on="Lockin 2" class="WFChart (strict)"("YScale.Maximum"="Y/Theta Range", "YScale.Minimum"=w961) -> ()  [unwired: 2 in, 2 out]
            n445 = property on="XY Graph" class="XYGraph (strict)"("XScale.Maximum"="XY Axis Range", "XScale.Minimum"=w958, "YScale.Maximum"="XY Axis Range", "YScale.Minimum"=w958) -> ()  [unwired: 2 in, 2 out]
            n446 = call <vilib>:"Add State(s) to Queue__jki_lib_state_machine.vi"("State(s) in (\"\")"=w966) -> ("States Out"=w965:string)  [unwired: 14 in]
          }
          frame "DONE: Update Status" {
            # "#done"
            n447 = Unbundle By Name(w967) -> ("DAQ state"=w969:T45)
            n448 = case shown="\"stopped\"" w969 {
              tunnel: ["Idle" ("Status") "Started" ("Status") "Stopped" ("Status") "Running" ("Status") "Sweeping" ("Status")] -> w968
              frame "idle", Default {
                w975 = FALSE ("Trigger")
                n449 = local write "Reset"(w975) -> ()
                n450 = local write "Trigger"(w975) -> ()
                n451 = local write "Start"(w975) -> ()
              }
              frame "started" {
                w976 = FALSE ("Trigger")
                n452 = local write "Start Sweep"(w976) -> ()
                n453 = local write "Reset"(w976) -> ()
                n454 = local write "Stop Sweep"(w976) -> ()
                n455 = local write "Start"(TRUE ("Trigger")) -> ()
              }
              frame "stopped" {
                w981 = FALSE ("Trigger")
                n456 = local write "Reset"(w981) -> ()
                n457 = local write "Trigger"(w981) -> ()
                n458 = local write "Start"(FALSE ("Trigger")) -> ()
              }
              frame "created" {
                n459 = local write "Start"(TRUE ("Start")) -> ()
                n460 = local write "Reset"(FALSE ("Reset")) -> ()
              }
              frame "sweeping" {
                n461 = call <userlib>:"MGI Milliseconds Since Last Reset.vi"("Reset (F)"=TRUE) -> ()  [unwired: 5 in, 2 out]
              }
            }
            n462 = local write "Status"(w968) -> ()
            n463 = call <vilib>:"Add State(s) to Queue__jki_lib_state_machine.vi"("State(s) in (\"\")"=w973) -> ("States Out"=w972:string)  [unwired: 14 in]
          }
          frame "DONE: Update Sweep Timer" {
            # "#done"
            n464 = local read "Status"() -> (w990:string)
            n465 = local read "Sweep Time (s)"() -> (w988:dbl)
            n466 = local read "Initial Wait (s)"() -> (w987:dbl)
            n467 = case shown="\"Sweeping\"" w990 {
              tunnel: [0.0 w1000] -> w989
              tunnel: w988 -> [_ w998]
              tunnel: w987 -> [_ w997]
              frame Default {
              }
              frame "Sweeping" {
                # "some overhead"
                n468 = call <userlib>:"MGI Milliseconds Since Last Reset.vi"() -> ("ms"=w1004:u32)  [unwired: 6 in, 1 out]
                n469 = Divide(x=w1004, y=u32 1000) -> (x/y=w1002:dbl)
                n470 = Negate(x=w1002) -> (-x=w1001:dbl)
                n471 = Compound Arithmetic op=ADD(2.0 ("value"), w997, w998, w1001) -> (w1000:dbl)
              }
            }
            "Sweep Timer (s)" <- w989
            n472 = call <vilib>:"Add State(s) to Queue__jki_lib_state_machine.vi"("State(s) in (\"\")"=w995) -> ("States Out"=w994:string)  [unwired: 14 in]
          }
          frame "UI: Defer Panel Updates" {
            n473 = case shown="\"True\"" w1006 {
              tunnel: [FALSE ("Defer Updates?") TRUE ("Defer Updates?")] -> w1005
              frame "False", Default {
              }
              frame "True" {
              }
            }
            n474 = call <userlib>:"MGI Defer Panel Updates.vi"("Error In"=w1008, "Defer Updates?"=w1005) -> ("Error Out"=w1007:errorcluster)  [unwired: 9 in]
            n475 = call <vilib>:"Add State(s) to Queue__jki_lib_state_machine.vi"("State(s) in (\"\")"=w1012) -> ("States Out"=w1011:string)  [unwired: 14 in]
          }
          frame "UI: Cursor Set" {
            # "Argument"
            # "Set and Unset Cursor Busy.\n(Usage: \"UI: Cursor Set >> Busy|Idle\")"
            n476 = case shown="\"Busy\"" w1019 {
              tunnel: w1016 -> [w1023 w1025]
              tunnel: [w1022 w1024] -> w1015
              frame "Idle", Default {
                n477 = call <vilib>:"Unset Busy.vi"("error in (no error)"=w1023) -> ("error out"=w1022:errorcluster)  [unwired: 10 in]
              }
              frame "Busy" {
                n478 = call <vilib>:"Set Busy.vi"("error in (no error)"=w1025) -> ("error out"=w1024:errorcluster)  [unwired: 9 in, 1 out]
              }
            }
            n479 = call <vilib>:"Add State(s) to Queue__jki_lib_state_machine.vi"("State(s) in (\"\")"=w1021) -> ("States Out"=w1020:string)  [unwired: 14 in]
          }
          frame "UI: Front Panel State" {
            # "Argument"
            n480 = Unbundle By Name(w1028) -> ("Core.Current VI Reference"=w1030:refnum<vi>)
            n481 = case shown="\"Open\", Default" w1029 {
              tunnel: w1031 -> [w1037 w1050]
              tunnel: [w1039 w1051] -> w1027
              tunnel: w1030 -> [w1038 w1048]
              frame "Open", Default {
                n482 = property class="VI"(reference=w1038, error in=w1037) -> (reference out=w1035:refnum<vi>, error out=w1036:errorcluster, "Front Panel.Open"=w1034:bool)
                n483 = case shown="True" w1034 {
                  tunnel: [w1042 w1045] -> w1039
                  tunnel: w1036 -> [w1041 w1045]
                  tunnel: w1035 -> [w1040 _]
                  frame False {
                    n484 = invoke class="VI" method="FP.Open"(reference=w1040, error in=w1041, "Activate"=TRUE, "State"=T19."Standard") -> (error out=w1042:errorcluster)  [unwired: 1 in, 4 out]
                  }
                  frame True {
                  }
                }
              }
              frame "Close" {
                n485 = property class="VI"(reference=w1048, error in=w1050) -> (reference out=w1047:refnum<vi>, error out=w1049:errorcluster, "Front Panel.Open"=w1046:bool)
                n486 = case shown="True" w1046 {
                  tunnel: [w1052 w1055] -> w1051
                  tunnel: w1049 -> [w1052 w1054]
                  tunnel: w1047 -> [_ w1053]
                  frame False {
                  }
                  frame True {
                    n487 = invoke class="VI" method="FP.Close"(reference=w1053, error in=w1054) -> (error out=w1055:errorcluster)  [unwired: 1 in, 2 out]
                  }
                }
              }
            }
            n488 = call <vilib>:"Add State(s) to Queue__jki_lib_state_machine.vi"("State(s) in (\"\")"=w1033) -> ("States Out"=w1032:string)  [unwired: 14 in]
          }
          frame "DONE: Update Sweep Results Graphs" {
            # "#done"
            n489 = Unbundle By Name(w1058) -> ("SweepResults.X results"=→"Sweep Results X":waveform(dbl)[], "SweepResults.Y Results"=→"Sweep Results Y":waveform(dbl)[])
            n490 = call <vilib>:"Add State(s) to Queue__jki_lib_state_machine.vi"("State(s) in (\"\")"=w1062) -> ("States Out"=w1061:string)  [unwired: 14 in]
          }
          frame "DONE: Update Sweep WFMs Graphs" {
            # "#done"
            n491 = Unbundle By Name(w1065) -> ("SweepWaveforms.Sweep_AO"=→"Sweep Results AO":waveform(dbl)[], "SweepWaveforms.Sweep_AI"=→"Sweep Results AI":waveform(dbl)[])
            n492 = call <vilib>:"Add State(s) to Queue__jki_lib_state_machine.vi"("State(s) in (\"\")"=w1069) -> ("States Out"=w1068:string)  [unwired: 14 in]
          }
          frame "DONE: Sync Lockin Plot Visibility" {
            # "#done\n(mostly)"
            # "#done"
            # "Do not put any code in this frame.\n(It is a separator no-op. You can make a copy of this frame to create a new UI frame)"
            n493 = local read "Results Plot Names"() -> (w1072:string[])
            n494 = Array Size(array=w1072) -> (size(s)=w1073:i32)
            n495 = feedback #1() -> (w1075:string[])  [unwired: 1 in]
            n496 = feedback-in #1(w1072) -> ()
            n497 = Not Equal?(x=w1075, y=w1072) -> (x != y?=w1077:bool)
            n498 = First Call?() -> (First Call?: T/F=w1078:bool)
            n499 = Or(x=w1078, y=w1077) -> (x .or. y?=w1076:bool)
            n500 = case shown="True" w1076 {
              tunnel: w1071 -> [w1100 w1104]
              tunnel: w1072 -> [_ w1105]
              tunnel: [w1100 w1101] -> w1074
              frame False {
              }
              frame True {
                n501 = for {
                  tunnel: w1104 -> [w1126]
                  tunnel: [w1111] -> w1102
                  tunnel: w1105 -> [w1106] mode=indexing
                  i -> [w1121]
                  n502 = control-ref of="XY Graph"() -> (w1116:refnum<vi>)
                  n503 = control-ref of="Lockin 2"() -> (w1117:refnum<vi>)
                  n504 = control-ref of="Lockin 1"() -> (w1118:refnum<vi>)
                  n505 = call <userlib>:"Legend - WaveformChart.vi"("error in (no error)"=w1126, "Plot.Plot Name"=w1106, "Active Plot"=w1121, "WaveformChart in"=w1118) -> ("error out"=w1122:errorcluster, "Plot.Plot Name"=w1120:string, "Active Plot"=w1125:i32)  [unwired: 4 in, 1 out]
                  n506 = control-ref of="Sweep Results Y"() -> (w1114:refnum<vi>)
                  n507 = control-ref of="Sweep Results X"() -> (w1115:refnum<vi>)
                  n508 = call <userlib>:"Legend - WaveformChart.vi"("error in (no error)"=w1122, "Plot.Plot Name"=w1120, "Active Plot"=w1125, "WaveformChart in"=w1117) -> ("error out"=w1123:errorcluster, "Plot.Plot Name"=w1119:string, "Active Plot"=w1124:i32)  [unwired: 4 in, 1 out]
                  n509 = call <userlib>:"Legend - XYGraph.vi"("error in (no error)"=w1123, "Plot.Plot Name"=w1119, "Active Plot"=w1124, "XYGraph in"=w1116) -> ("error out"=w1113:errorcluster, "Plot.Plot Name"=w1107:string, "Active Plot"=w1110:i32)  [unwired: 4 in, 1 out]
                  n510 = call <userlib>:"Legend - WaveformGraph.vi"("error in (no error)"=w1113, "Plot.Plot Name"=w1107, "Active Plot"=w1110, "WFGraph in"=w1115) -> ("error out"=w1112:errorcluster, "Plot.Plot Name"=w1108:string, "Active Plot"=w1109:i32)  [unwired: 4 in, 1 out]
                  n511 = call <userlib>:"Legend - WaveformGraph.vi"("error in (no error)"=w1112, "Plot.Plot Name"=w1108, "Active Plot"=w1109, "WFGraph in"=w1114) -> ("error out"=w1111:errorcluster)  [unwired: 4 in, 3 out]
                }
                n512 = property on="Channel" class="Ring (strict)"(error in=w1104, "Strings []"=w1105) -> (error out=w1103:errorcluster)  [unwired: 1 in, 1 out]
                n513 = Merge Errors(w1103, w1102) -> (w1101:errorcluster)
              }
            }
            n514 = for {
              N: w1073 -> [_]
              tunnel: w1074 -> [w1089]
              tunnel: [w1084] -> w1070
              i -> [w1098]
              n515 = control-ref of="Lockin 1"() -> (w1099:refnum<vi>)
              n516 = call <userlib>:"Get Plot Visibility - WaveformChart.vi"("error in (no error)"=w1089, "ActPlot"=w1098, "WaveformChart in"=w1099) -> ("error out"=w1088:errorcluster, "Plot.Visible?"=w1083:bool, "Active Plot"=w1093:i32)  [unwired: 6 in]
              n517 = control-ref of="Lockin 2"() -> (w1097:refnum<vi>)
              n518 = call <userlib>:"Set Plot Visibility - WaveformChart.vi"("error in (no error)"=w1088, "Plot.Visible?"=w1083, "ActPlot"=w1093, "WaveformChart in"=w1097) -> ("error out"=w1087:errorcluster, "Active Plot"=w1092:i32)  [unwired: 6 in]
              n519 = control-ref of="XY Graph"() -> (w1096:refnum<vi>)
              n520 = call <userlib>:"Set Plot Visibility - XYGraph.vi"("error in (no error)"=w1087, "Plot.Visible?"=w1083, "ActPlot"=w1092, "XYGraph in"=w1096) -> ("error out"=w1086:errorcluster, "Active Plot"=w1091:i32)  [unwired: 6 in]
              n521 = control-ref of="Sweep Results Y"() -> (w1095:refnum<vi>)
              n522 = control-ref of="Sweep Results X"() -> (w1094:refnum<vi>)
              n523 = call <userlib>:"Set Plot Visibility - WaveformGraph.vi"("error in (no error)"=w1086, "Plot.Visible?"=w1083, "ActPlot"=w1091, "WFGraph in"=w1095) -> ("error out"=w1085:errorcluster, "Active Plot"=w1090:i32)  [unwired: 6 in]
              n524 = call <userlib>:"Set Plot Visibility - WaveformGraph.vi"("error in (no error)"=w1085, "Plot.Visible?"=w1083, "ActPlot"=w1090, "WFGraph in"=w1094) -> ("error out"=w1084:errorcluster)  [unwired: 6 in, 1 out]
            }
            n525 = call <vilib>:"Add State(s) to Queue__jki_lib_state_machine.vi"("State(s) in (\"\")"=w1082) -> ("States Out"=w1081:string)  [unwired: 14 in]
          }
          frame "DONE: Lockin 1 Plot Visible" {
            # "#done"
            # "Do not put any code in this frame.\n(It is a separator no-op. You can make a copy of this frame to create a new UI frame)"
            n526 = case shown="\"All\"" w1139 {
              tunnel: [FALSE TRUE] -> w1135
              frame "None", Default {
              }
              frame "All" {
              }
            }
            n527 = control-ref of="Lockin 1"() -> (w1138:refnum<vi>)
            n528 = control-ref of="Lockin 2"() -> (w1136:refnum<vi>)
            n529 = control-ref of="Sweep Results X"() -> (w1134:refnum<vi>)
            n530 = control-ref of="Sweep Results Y"() -> (w1133:refnum<vi>)
            n531 = call <userlib>:"Plots Visible - All or None - WaveformChart.vi"("error in (no error)"=w1137, "All Visible?"=w1135, "WaveformChart in"=w1138) -> ("error out"=w1131:errorcluster)  [unwired: 7 in, 1 out]
            n532 = call <userlib>:"Plots Visible - All or None - WaveformChart.vi"("error in (no error)"=w1131, "All Visible?"=w1135, "WaveformChart in"=w1136) -> ("error out"=w1130:errorcluster)  [unwired: 7 in, 1 out]
            n533 = call <userlib>:"Plots Visible - All or None - WaveformGraph.vi"("error in (no error)"=w1130, "All Visible?"=w1135, "WFGraph in"=w1134) -> ("error out"=w1129:errorcluster)  [unwired: 7 in, 1 out]
            n534 = control-ref of="XY Graph"() -> (w1132:refnum<vi>)
            n535 = call <userlib>:"Plots Visible - All or None - WaveformGraph.vi"("error in (no error)"=w1129, "All Visible?"=w1135, "WFGraph in"=w1133) -> ("error out"=w1128:errorcluster)  [unwired: 7 in, 1 out]
            n536 = call <userlib>:"Plots Visible - All or None - XYGraph.vi"("error in (no error)"=w1128, "All Visible?"=w1135, "XYGraph in"=w1132) -> ("error out"=w1127:errorcluster)  [unwired: 7 in, 1 out]
            n537 = call <vilib>:"Add State(s) to Queue__jki_lib_state_machine.vi"("State(s) in (\"\")"=w1143) -> ("States Out"=w1142:string)  [unwired: 14 in]
          }
          frame "DONE: Update Lockin Graphs" {
            # "#todo\nshould be owned by Lockin UI"
            # "#todo\nshould be owned by Lockin UI"
            n538 = Unbundle By Name(w1163) -> ("Lockin"=w1150:refnum<class "Instrument.Lockin.lvclass">)
            n539 = call "Parse Results (table).vi"("error in (no error)"=w1155, "Results (Dictionary)"=w1150) -> ("error out"=w1154:errorcluster, 1:→"Results", "Table"=w1149:string[][])  [unwired: 6 in, 1 out]
            n540 = call "Dictionary to Chart.vi"("error in (no error)"=w1154, "Display"="Display", "Results (Dictionary)"=w1149) -> ("error out"=w1156:errorcluster, "Y/Theta Array"=→"XY Graph":waveform(dbl)[], "X/R Array"=→"Lockin 2":waveform(dbl)[], "Results (Dictionary) out"=→"Lockin 1":cluster{"key":string, "value":dbl}[], 4:→"Results Plot Names")  [unwired: 4 in]
            n541 = call "Dictionary to Indicator.vi"("Results (Dictionary)"=w1149, "AI Channel"="Channel", "error in (no error)"=w1156) -> ("X"=→"X":dbl, "Y"=→"Y":dbl, "R"=→"R":dbl, "Theta"=→"Theta":dbl, "error out"=w1148:errorcluster)  [unwired: 8 in]
            n542 = call <vilib>:"Add State(s) to Queue__jki_lib_state_machine.vi"("State(s) in (\"\")"=w1166) -> ("States Out"=w1165:string)  [unwired: 14 in]
          }
          frame "DONE: Update Displays" {
            # "#done"
            n543 = local read "Display"() -> (w1169:enum16{"X and Y", "R and Theta", "Mean"})
            n544 = case shown="\"R and Theta\"" w1169 {
              tunnel: ["X (V)" "R (V)"] -> _
              tunnel: ["Y (V)" "Theta (°)"] -> _
              tunnel: ["Lockin X (V)" "R (V)"] -> w1168
              tunnel: ["Lockin Y (V)" "Theta (°)"] -> w1167
              frame "X and Y", Default {
              }
              frame "R and Theta" {
              }
            }
            n545 = property on="Lockin 1" class="WFChart (strict)"("YScale.NameLbl.Text"=w1168) -> ()  [unwired: 2 in, 2 out]
            n546 = property on="Lockin 2" class="WFChart (strict)"("YScale.NameLbl.Text"=w1167) -> ()  [unwired: 2 in, 2 out]
            n547 = call <vilib>:"Add State(s) to Queue__jki_lib_state_machine.vi"("State(s) in (\"\")"=w1174) -> ("States Out"=w1173:string)  [unwired: 14 in]
          }
          frame "DONE: Update Waveform Graphs" {
            # "#done"
            # "#todo\nshould be owned by Lockin UI"
            # "private"
            # "private"
            n548 = Unbundle By Name(w1201) -> ("Lockin"=w1193:refnum<class "Instrument.Lockin.lvclass">)
            n549 = local read "Y Axis (Output)"() -> (w1186:enum16{"Analog Output", "Reference"})
            n550 = Unbundle By Name(w1193) -> ("AI.Gain"=w1189:T40, "AI"=w1204:waveform(dbl)[], "AO"=w1195:waveform(dbl)[], "RefX"=w1185:waveform(dbl)[], "RefY"=w1184:waveform(dbl)[])
            n551 = local read "X Axis"() -> (w1191:enum16{"Time", "Samples"})
            n552 = Interleave 1D Arrays(w1185, w1184) -> (w1183:waveform(dbl)[])
            n553 = case shown="\"Reference\"" w1186 {
              tunnel: w1195 -> [w1212 _]
              tunnel: w1183 -> [_ w1213]
              tunnel: [w1212 w1213] -> w1194
              frame "Analog Output", Default {
              }
              frame "Reference" {
              }
            }
            n554 = Power Of 10(x="Decimate") -> (10^x=w1196:dbl)
            n555 = call "Display n or dt.vi"("error in (no error)"=w1192, "X Axis"=w1191, "Input Waveforms"=w1204) -> ("error out"=w1203:errorcluster, "Output Waveforms"=w1190:waveform(dbl)[])  [unwired: 7 in]
            n556 = call "Display n or dt.vi"("error in (no error)"=w1192, "X Axis"=w1191, "Input Waveforms"=w1194) -> ("error out"=w1202:errorcluster, "Output Waveforms"=w1207:waveform(dbl)[])  [unwired: 7 in]
            n557 = call "Decimate Waveforms.vi"("WFM"=w1207, "averaging"=FALSE, "decimating factor"=w1196, "error in (no error)"=w1202) -> ("WFM out"=→"AO Graph":waveform(dbl)[])  [unwired: 5 in, 1 out]
            n558 = call "Decimate Waveforms.vi"("WFM"=w1190, "averaging"=FALSE, "decimating factor"=w1196, "error in (no error)"=w1203) -> ("WFM out"=w1200:waveform(dbl)[], "error out"=w1198:errorcluster)  [unwired: 5 in]
            n559 = case shown="\"ADC\"" "Y Axis (Input)" {
              tunnel: w1200 -> [w1215 w1220]
              tunnel: w1189 -> [_ w1218]
              tunnel: [w1215 w1219] -> w1199
              tunnel: w1198 -> [w1214 w1217]
              tunnel: [w1214 w1216] -> w1188
              frame "Device", Default {
              }
              frame "ADC" {
                n560 = call "Multiply by Gain.vi"("error in (no error)"=w1217, "Gain"=w1218, "WFM in"=w1220) -> ("error out"=w1216:errorcluster, "WFM out"=w1219:waveform(dbl)[])  [unwired: 7 in]
              }
            }
            "AI Graph" <- w1199
            n561 = call <vilib>:"Add State(s) to Queue__jki_lib_state_machine.vi"("State(s) in (\"\")"=w1211) -> ("States Out"=w1210:string)  [unwired: 14 in]
          }
          frame "DONE: AO Graph Plot Visible" {
            # "#done"
            # "Do not put any code in this frame.\n(It is a separator no-op. You can make a copy of this frame to create a new UI frame)"
            n562 = case shown="\"All\"" w1227 {
              tunnel: [FALSE TRUE] -> w1223
              frame "None", Default {
              }
              frame "All" {
              }
            }
            n563 = control-ref of="AO Graph"() -> (w1225:refnum<vi>)
            n564 = call <userlib>:"Plots Visible - All or None - WaveformGraph.vi"("error in (no error)"=w1226, "All Visible?"=w1223, "WFGraph in"=w1225) -> ("error out"=w1222:errorcluster)  [unwired: 7 in, 1 out]
            n565 = control-ref of="Sweep Results AO"() -> (w1224:refnum<vi>)
            n566 = call <userlib>:"Plots Visible - All or None - WaveformGraph.vi"("error in (no error)"=w1222, "All Visible?"=w1223, "WFGraph in"=w1224) -> ("error out"=w1221:errorcluster)  [unwired: 7 in, 1 out]
            n567 = call <vilib>:"Add State(s) to Queue__jki_lib_state_machine.vi"("State(s) in (\"\")"=w1231) -> ("States Out"=w1230:string)  [unwired: 14 in]
          }
          frame "DONE: AI Graph Plot Visible" {
            # "#done"
            # "Do not put any code in this frame.\n(It is a separator no-op. You can make a copy of this frame to create a new UI frame)"
            n568 = case shown="\"All\"" w1239 {
              tunnel: [FALSE TRUE] -> w1236
              frame "None", Default {
              }
              frame "All" {
              }
            }
            n569 = control-ref of="AI Graph"() -> (w1240:refnum<vi>)
            n570 = control-ref of="Sweep Results AI"() -> (w1237:refnum<vi>)
            n571 = call <userlib>:"Plots Visible - All or None - WaveformGraph.vi"("error in (no error)"=w1238, "All Visible?"=w1236, "WFGraph in"=w1240) -> ("error out"=w1235:errorcluster)  [unwired: 7 in, 1 out]
            n572 = call <userlib>:"Plots Visible - All or None - WaveformGraph.vi"("error in (no error)"=w1235, "All Visible?"=w1236, "WFGraph in"=w1237) -> ("error out"=w1234:errorcluster)  [unwired: 7 in, 1 out]
            n573 = call <vilib>:"Add State(s) to Queue__jki_lib_state_machine.vi"("State(s) in (\"\")"=w1244) -> ("States Out"=w1243:string)  [unwired: 14 in]
          }
          frame "DONE: Enable Buttons" {
            # "#done"
            n574 = control-ref of="Start"() -> (w1252:refnum<vi>)
            n575 = control-ref of="Pause"() -> (w1251:refnum<vi>)
            n576 = control-ref of="Trigger"() -> (w1250:refnum<vi>)
            n577 = control-ref of="Reset"() -> (w1249:refnum<vi>)
            n578 = control-ref of="Help"() -> (w1248:refnum<vi>)
            n579 = Build Array(w1252, w1251, w1250, w1249, w1248) -> (w1247:refnum<vi>[])
            n580 = for {
              tunnel: w1247 -> [w1259] mode=indexing
              n581 = property class="Bool (strict)"(reference=w1259, "DisabledEnum"=T20."Enabled" ("Disabled")) -> ()  [unwired: 1 in, 2 out]
            }
            n582 = call <vilib>:"Add State(s) to Queue__jki_lib_state_machine.vi"("State(s) in (\"\")"=w1257) -> ("States Out"=w1256:string)  [unwired: 14 in]
          }
          frame "DONE: Disable Buttons" {
            # "#done"
            n583 = control-ref of="Start"() -> (w1265:refnum<vi>)
            n584 = control-ref of="Pause"() -> (w1264:refnum<vi>)
            n585 = control-ref of="Trigger"() -> (w1263:refnum<vi>)
            n586 = control-ref of="Reset"() -> (w1262:refnum<vi>)
            n587 = control-ref of="Help"() -> (w1261:refnum<vi>)
            n588 = Build Array(w1265, w1264, w1263, w1262, w1261) -> (w1260:refnum<vi>[])
            n589 = for {
              tunnel: w1260 -> [w1272] mode=indexing
              n590 = property class="Bool (strict)"(reference=w1272, "DisabledEnum"=T20."Disabled and Grayed Out" ("Disabled")) -> ()  [unwired: 1 in, 2 out]
            }
            n591 = call <vilib>:"Add State(s) to Queue__jki_lib_state_machine.vi"("State(s) in (\"\")"=w1270) -> ("States Out"=w1269:string)  [unwired: 14 in]
          }
          frame "DONE: Sync AO AI Plot Visibility" {
            # "#done"
            # "Do not put any code in this frame.\n(It is a separator no-op. You can make a copy of this frame to create a new UI frame)"
            n592 = Unbundle By Name(w1279) -> ("Lockin"=w1277:refnum<class "Instrument.Lockin.lvclass">)
            n593 = call "Get AO StringsAndValues.vi"("error in (no error)"=w1275, "Configuration.DAQ"=w1277) -> ("error out"=w1273:errorcluster, "AO Strings and Values"=w1276:cluster{string, i32}[])  [unwired: 8 in]
            n594 = call "Get AI StringsAndValues.vi"("error in (no error)"=w1275, "Configuration.DAQ"=w1277) -> ("error out"=w1274:errorcluster, "AI StringsAndValues"=w1278:cluster{string, i32}[])  [unwired: 8 in]
            n595 = for {
              tunnel: w1274 -> [w1299]
              tunnel: [w1295] -> w1281
              tunnel: w1278 -> [_] mode=indexing
              i -> [w1302]
              n596 = control-ref of="AI Graph"() -> (w1298:refnum<vi>)
              n597 = property on="Property Node" class="WFGraph (strict)"(reference=w1298, error in=w1299, "Active Plot"=w1302) -> (error out=w1303:errorcluster, "Plot.Visible?"=w1301:bool)  [unwired: 1 out]
              n598 = control-ref of="Sweep Results AI"() -> (w1300:refnum<vi>)
              n599 = property on="Property Node" class="WFGraph (strict)"(reference=w1300, error in=w1303, "Active Plot"=w1302, "Plot.Visible?"=w1301) -> (error out=w1296:errorcluster)  [unwired: 1 out]
              n600 = call <vilib>:"Clear Errors.vi"("error in (no error)"=w1296, "specific error code to clear (0: all)"=1077) -> ("error out"=w1295:errorcluster)  [unwired: 4 in, 1 out]
            }
            n601 = for {
              tunnel: w1273 -> [w1289]
              tunnel: [w1286] -> w1282
              tunnel: w1276 -> [_] mode=indexing
              i -> [w1293]
              n602 = control-ref of="AO Graph"() -> (w1290:refnum<vi>)
              n603 = property on="Property Node" class="WFGraph (strict)"(reference=w1290, error in=w1289, "Active Plot"=w1293) -> (error out=w1294:errorcluster, "Plot.Visible?"=w1292:bool)  [unwired: 1 out]
              n604 = control-ref of="Sweep Results AO"() -> (w1291:refnum<vi>)
              n605 = property on="Property Node" class="WFGraph (strict)"(reference=w1291, error in=w1294, "Active Plot"=w1293, "Plot.Visible?"=w1292) -> (error out=w1287:errorcluster)  [unwired: 1 out]
              n606 = call <vilib>:"Clear Errors.vi"("error in (no error)"=w1287, "specific error code to clear (0: all)"=1077) -> ("error out"=w1286:errorcluster)  [unwired: 4 in, 1 out]
            }
            n607 = Merge Errors(w1281, w1282) -> (w1280:errorcluster)
            n608 = call <vilib>:"Add State(s) to Queue__jki_lib_state_machine.vi"("State(s) in (\"\")"=w1285) -> ("States Out"=w1284:string)  [unwired: 14 in]
          }
          frame "DONE: Initialize AI Ch" {
            # "#done"
            # "Add or remove AI channels"
            n609 = Unbundle By Name(w1310) -> ("Lockin"=w1308:refnum<class "Instrument.Lockin.lvclass">)
            n610 = call "Initialize AI Channels.vi"("error in (no error)"=w1307, "Instrument.DAQ"=w1308) -> ("error out"=w1306:errorcluster, 2:w1309, "Instrument.DAQ out"=w1304:refnum<class "Instrument.DAQ.lvclass">)  [unwired: 7 in]
            n611 = property on="AI Channels" class="Arr (strict)"(error in=w1306, "Val(Sgnl)"=w1309) -> (error out=w1305:errorcluster)  [unwired: 1 in, 1 out]
            n612 = Bundle By Name(cluster=w1310, "Lockin"=w1304) -> (w1311:T44)
            n613 = call <vilib>:"Add State(s) to Queue__jki_lib_state_machine.vi"("State(s) in (\"\")"=w1314) -> ("States Out"=w1313:string)  [unwired: 14 in]
          }
          frame "DONE: Initialize AO Ch" {
            # "#done"
            n614 = Unbundle By Name(w1321) -> ("Lockin"=w1320:refnum<class "Instrument.Lockin.lvclass">)
            n615 = call "Initialize AO Channels.vi"("error in (no error)"=w1318, "Instrument.DAQ"=w1320) -> ("error out"=w1317:errorcluster, 2:w1316, "Instrument.DAQ out"=w1319:refnum<class "Instrument.DAQ.lvclass">)  [unwired: 7 in]
            n616 = property on="AO Channels" class="Arr (strict)"(error in=w1317, "Val(Sgnl)"=w1316) -> (error out=w1315:errorcluster)  [unwired: 1 in, 1 out]
            n617 = Bundle By Name(cluster=w1321, "Lockin"=w1319) -> (w1322:T44)
            n618 = call <vilib>:"Add State(s) to Queue__jki_lib_state_machine.vi"("State(s) in (\"\")"=w1325) -> ("States Out"=w1324:string)  [unwired: 14 in]
          }
          frame "DONE: Initialize REF Ch" {
            # "#done"
            n619 = Unbundle By Name(w1332) -> ("Lockin"=w1331:refnum<class "Instrument.Lockin.lvclass">)
            n620 = call "Initialize REF Channels.vi"("error in (no error)"=w1329, "Instrument.DAQ"=w1331) -> ("error out"=w1327:errorcluster, 2:w1328, "Instrument.DAQ out"=w1330:refnum<class "Instrument.DAQ.lvclass">)  [unwired: 7 in]
            n621 = property on="REF Channels" class="Arr (strict)"(error in=w1327, "Val(Sgnl)"=w1328) -> (error out=w1326:errorcluster)  [unwired: 1 in, 1 out]
            n622 = Bundle By Name(cluster=w1332, "Lockin"=w1330) -> (w1333:T44)
            n623 = call <vilib>:"Add State(s) to Queue__jki_lib_state_machine.vi"("State(s) in (\"\")"=w1336) -> ("States Out"=w1335:string)  [unwired: 14 in]
          }
          frame "DONE: Initialize" {
            w1337 = waveform(dbl)[][] [] ("History Data")
            # "#done"
            # "Initialize the User Interface, here.\n(this is called automatically, by the Macro: Init)"
            n624 = invoke on="Start" class="Bool (strict)" method="Reinit To Default"() -> ()  [unwired: 3 in, 3 out]
            n625 = invoke on="Start Sweep" class="Bool (strict)" method="Reinit To Default"() -> ()  [unwired: 3 in, 3 out]
            n626 = invoke on="Reset" class="Bool (strict)" method="Reinit To Default"() -> ()  [unwired: 3 in, 3 out]
            n627 = invoke on="Close" class="Bool (strict)" method="Reinit To Default"() -> ()  [unwired: 3 in, 3 out]
            n628 = property on="Lockin 1" class="WFChart (strict)"("History Data"=w1337) -> ()  [unwired: 2 in, 2 out]
            n629 = local write "Tab Control 2"(T13."AO/AI Display" ("Tab Control 2")) -> ()
            n630 = local write "Tab Control 4"(T1."AO/REF Setup" ("Tab Control 4")) -> ()
            n631 = property on="Lockin 2" class="WFChart (strict)"("History Data"=w1337) -> ()  [unwired: 2 in, 2 out]
            n632 = local write "Status"("Starting" ("Status")) -> ()
            n633 = invoke on="Trigger" class="Bool (strict)" method="Reinit To Default"() -> ()  [unwired: 3 in, 3 out]
            n634 = invoke on="Help" class="Bool (strict)" method="Reinit To Default"() -> ()  [unwired: 3 in, 3 out]
            n635 = call <userlib>:"MGI Get Executable Version.vi"() -> ("Version"=w1342:string)  [unwired: 7 in]
            n636 = Empty String/Path?(string/path=w1342) -> (empty?=w1343:bool)
            n637 = call <userlib>:"Fit VI window to Largest Dec__ogtk.vi"("error in (no error)"=w1346) -> ("error out"=w1348:errorcluster)  [unwired: 5 in, 1 out]
            n638 = Select(t=w1339, s=w1343, f=w1342) -> (s? t:f=w1341:string)
            n639 = Format Into String(format string="v%s", w1341) -> (resulting string=→"Version":string)  [unwired: 2 in, 1 out]
            n640 = call <vilib>:"Add State(s) to Queue__jki_lib_state_machine.vi"("State(s) in (\"\")"=w1352) -> ("States Out"=w1351:string)  [unwired: 14 in]
          }
          frame "DONE: Create Logger" {
            w1376 = T79 3 items=["User Home"=0, "User Desktop"=1, "User Documents"=2, "User Application Data"=3, "User Preferences"=4, "User Temporary"=5, "Public Documents"=6, "Public Application Data"=7, "Public Preferences"=8, "Public Cache"=13, "System Core Libraries"=9, "System Installed Libraries"=10, "Application Files"=11, "Boot Volume Root"=12] ("system directory type")
            n641 = Unbundle By Name(w1362) -> ("RemoteControl"=w1354:refnum<class "RemoteControl.lvclass">, "Lockin.DAQ"=w1368:refnum<class "Instrument.DAQ.lvclass">, "Logger.Error"=w1371:refnum<class "Logger.Error.lvclass">, "Lockin"=w1355:refnum<class "Instrument.Lockin.lvclass">)
            n642 = call-dynamic "Get SMO Name.vi"("error in (no error)"=w1356, "Instrument.Lockin"=w1355) -> ("error out"=w1357:errorcluster, "SMO Name"=w1359:string, "Instrument.Lockin out"=w1358:refnum<class "Instrument.Lockin.lvclass">)  [unwired: 7 in]
            n643 = call <vilib>:"Get System Directory.vi"("system directory type"=w1376) -> ("system directory"=w1378:path)  [unwired: 10 in]
            n644 = Build Path(base path=w1378, name or relative path="LevyLab") -> (appended path=w1375:path)
            n645 = call <vilib>:"Create.vi"("error in (no error)"=w1357, "SMO"=w1371) -> ("error out"=w1365:errorcluster, "SMO out"=w1370:refnum<class "Logger.Error.lvclass">)  [unwired: 7 in, 1 out]
            n646 = Build Path(base path=w1375, name or relative path="Error Logs") -> (appended path=w1373:path)
            n647 = Build Path(base path=w1373, name or relative path=w1359) -> (appended path=w1372:path)
            n648 = Build Array(w1354, w1368, w1358) -> (w1367:refnum<class "SMO.lvclass">[])
            n649 = call-dynamic "Write path.vi"("error in (no error)"=w1365, "folder"=w1372, "Logger in"=w1370) -> ("error out"=w1366:errorcluster, "Logger out"=w1369:refnum<class "Logger.Error.lvclass">)  [unwired: 7 in]
            n650 = call <userlib>:"Write Dependencies.vi"("error in (no error)"=w1366, "SMOs"=w1367, "Logger.Error in"=w1369) -> ("error out"=w1364:errorcluster, "Logger.Error out"=w1363:refnum<class "Logger.Error.lvclass">)  [unwired: 7 in]
            n651 = call <vilib>:"Start.vi"("error in (no error)"=w1364, "SMO"=w1363) -> ("error out"=w1360:errorcluster, "SMO out"=w1361:refnum<class "Logger.Error.lvclass">)  [unwired: 8 in]
            n652 = Bundle By Name(cluster=w1362, "Logger.Error"=w1361) -> (w1353:T44)
            n653 = call <vilib>:"Add State(s) to Queue__jki_lib_state_machine.vi"("State(s) in (\"\")"=w1381) -> ("States Out"=w1380:string)  [unwired: 14 in]
          }
          frame "DONE: Stop Logger" {
            n654 = Unbundle By Name(w1387) -> ("Logger.Error"=w1384:refnum<class "Logger.Error.lvclass">)
            n655 = call <vilib>:"GetState.vi"("error in (no error)"=w1383, "SMO"=w1384) -> ("SMO State"=w1385:T10, "SMO out"=w1386:refnum<class "Logger.Error.lvclass">)  [unwired: 7 in, 1 out]
            n656 = case shown="Default" w1385 {
              tunnel: [w1391 w1396] -> w1382
              tunnel: w1386 -> [_ w1399]
              tunnel: w1383 -> [w1391 w1398]
              frame "Stopped" {
              }
              frame Default {
                n657 = call <vilib>:"Stop.vi"("error in (no error)"=w1398, "SMO"=w1399) -> ("error out"=w1395:errorcluster, "SMO out"=w1394:refnum<class "Logger.Error.lvclass">)  [unwired: 8 in]
                n658 = call <vilib>:"GetState.vi"("error in (no error)"=w1395, "SMO"=w1394) -> ("error out"=w1393:errorcluster, "SMO out"=w1392:refnum<class "Logger.Error.lvclass">)  [unwired: 7 in, 1 out]
                n659 = call <vilib>:"Destroy.vi"("error in (no error)"=w1393, "SMO"=w1392) -> ("error out"=w1397:errorcluster)  [unwired: 9 in]
                n660 = call <vilib>:"Clear Errors.vi"("error in (no error)"=w1397) -> ("error out"=w1396:errorcluster)  [unwired: 5 in, 1 out]
              }
            }
            n661 = call <vilib>:"Add State(s) to Queue__jki_lib_state_machine.vi"("State(s) in (\"\")"=w1390) -> ("States Out"=w1389:string)  [unwired: 14 in]
          }
          frame "DONE: Create Remote" {
            # "#done\n#framework"
            n662 = Unbundle By Name(w1402) -> ("RemoteControl"=w1408:refnum<class "RemoteControl.lvclass">)
            n663 = Unbundle By Name(w1402) -> ("Lockin"=w1403:refnum<class "Instrument.Lockin.lvclass">)
            n664 = call <vilib>:"GetState.vi"("error in (no error)"=w1409, "SMO"=w1408) -> ("error out"=w1404:errorcluster, "SMO State"=w1407:T10, "SMO out"=w1406:refnum<class "RemoteControl.lvclass">)  [unwired: 7 in]
            n665 = call <vilib>:"Clear Errors.vi"("error in (no error)"=w1404) -> ("error out"=w1400:errorcluster)  [unwired: 5 in, 1 out]
            n666 = case shown="Default" w1407 {
              tunnel: [w1414 w1420] -> w1410
              tunnel: w1400 -> [w1414 _]
              tunnel: w1406 -> [_ _]
              tunnel: w1403 -> [_ w1428]
              tunnel: w1402 -> [w1413 w1434]
              tunnel: [w1413 w1433] -> w1401
              frame "Created".."Stopped" {
              }
              frame Default {
                # "this program acts as the command \"server\"\nthe list of methods is maintained here."
                n667 = call-dynamic "Get SMO RC Type.vi"("Instrument in"=w1428) -> ("error out"=w1421:errorcluster, "RC Type"=w1426:T80, "Instrument out"=w1427:refnum<class "Instrument.Lockin.lvclass">)  [unwired: 8 in]
                n668 = call <userlib>:"RC Enum to RC Object.vi"("error in (no error)"=w1421, "RC Type"=w1426) -> ("error out"=w1422:errorcluster, "RemoteControl out"=w1425:refnum<class "RemoteControl.lvclass">)  [unwired: 8 in]
                n669 = call-dynamic "Get SMO Port.vi"("error in (no error)"=w1422, "Instrument.Lockin in"=w1427) -> ("error out"=w1431:errorcluster, "Port"=w1424:u16, "Instrument.Lockin out"=w1432:refnum<class "Instrument.Lockin.lvclass">)  [unwired: 7 in]
                n670 = call-dynamic "Write Port.vi"("error in (no error)"=w1431, "Port"=w1424, "RemoteControl in"=w1425) -> ("error out"=w1430:errorcluster, "RemoteControl out"=w1438:refnum<class "RemoteControl.lvclass">)  [unwired: 7 in]
                n671 = local read "Allowed remote system"() -> (w1437:string)
                n672 = call-dynamic "Get SMO Public API.vi"("error in (no error)"=w1430, "Instrument.Lockin"=w1432) -> ("error out"=w1429:errorcluster, "Commands"=w1435:string[])  [unwired: 7 in, 1 out]
                n673 = call-dynamic "Write Commands.vi"("error in (no error)"=w1429, "Commands"=w1435, "RemoteControl in"=w1438) -> ("error out"=w1417:errorcluster, "RemoteControl out"=w1419:refnum<class "RemoteControl.lvclass">)  [unwired: 7 in]
                n674 = call <userlib>:"Write Debug Mode.vi"("error in (no error)"=w1417, "Debug Mode?"=FALSE, "RemoteControl in"=w1419) -> ("error out"=w1416:errorcluster, "RemoteControl out"=w1418:refnum<class "RemoteControl.lvclass">)  [unwired: 7 in]
                n675 = call-dynamic "Create Server SMO.vi"("error in (no error)"=w1416, "RemoteControl in"=w1418) -> ("error out"=w1420:errorcluster, "RemoteControl out"=w1423:refnum<class "RemoteControl.lvclass">)  [unwired: 8 in]
                n676 = Bundle By Name(cluster=w1434, "RemoteControl.Configure.address"="127.0.0.1", "RemoteControl.Configure.Port"=w1424, "RemoteControl.Configure.AllowedRemote"=w1437, "RemoteControl.Configure.Commands"=w1435, "RemoteControl"=w1423) -> (w1433:T44)
              }
            }
            n677 = call <vilib>:"Add State(s) to Queue__jki_lib_state_machine.vi"("State(s) in (\"\")"=w1412) -> ("States Out"=w1411:string)  [unwired: 14 in]
          }
          frame "DONE: Start Remote" {
            # "#done\n#framework"
            # "#done"
            n678 = Unbundle By Name(w1440) -> ("RemoteControl"=w1447:refnum<class "RemoteControl.lvclass">)
            n679 = call <vilib>:"GetState.vi"("error in (no error)"=w1448, "SMO"=w1447) -> ("error out"=w1441:errorcluster, "SMO State"=w1446:T10, "SMO out"=w1445:refnum<class "RemoteControl.lvclass">)  [unwired: 7 in]
            n680 = call <vilib>:"Clear Errors.vi"("error in (no error)"=w1441) -> ("error out"=w1443:errorcluster)  [unwired: 5 in, 1 out]
            n681 = case shown="Default" w1446 {
              tunnel: [w1451 w1458] -> w1442
              tunnel: [w1452 w1454] -> w1439
              tunnel: w1443 -> [w1451 w1456]
              tunnel: w1440 -> [w1452 w1455]
              tunnel: w1445 -> [_ w1457]
              frame "Started" {
              }
              frame Default {
                # "Start SMO"
                n682 = call <vilib>:"Start.vi"("error in (no error)"=w1456, "SMO"=w1457) -> ("error out"=w1458:errorcluster, "SMO out"=w1453:refnum<class "RemoteControl.lvclass">)  [unwired: 8 in]
                n683 = Bundle By Name(cluster=w1455, "RemoteControl"=w1453) -> (w1454:T44)
              }
            }
            n684 = call <vilib>:"Add State(s) to Queue__jki_lib_state_machine.vi"("State(s) in (\"\")"=w1450) -> ("States Out"=w1449:string)  [unwired: 14 in]
          }
          frame "DONE: AllowedRemote" {
            # "#done\n#framework"
            # "#done"
            # "only an \"allowed remote system\" is allowed to control this VI"
            n685 = Unbundle By Name(w1465) -> ("RemoteControl"=w1460:refnum<class "RemoteControl.lvclass">, "RemoteControl.Configure"=w1459:T42)
            n686 = local read "Allowed remote system"() -> (w1462:string)
            n687 = Bundle By Name(cluster=w1459, "AllowedRemote"=w1462) -> (w1461:T42)
            n688 = call <userlib>:"RemoteControl.Configure.vi"("error in (no error)"=w1464, "Configure"=w1461, "RemoteControl"=w1460) -> ("error out"=w1463:errorcluster)  [unwired: 7 in, 1 out]
            n689 = call <vilib>:"Add State(s) to Queue__jki_lib_state_machine.vi"("State(s) in (\"\")"=w1468) -> ("States Out"=w1467:string)  [unwired: 14 in]
          }
          frame "DONE: Reply to Command" {
            # "#done\n#framework"
            # "responds to the RC:process"
            n690 = Unbundle By Name(w1473) -> ("RemoteControl"=w1474:refnum<class "RemoteControl.lvclass">, "HandledMessage"=w1470:T43)
            n691 = Bundle("HandledMessage"=w1470) -> (w1469:cluster{"HandledMessage":T43})  [unwired: 1 in]
            n692 = call <userlib>:"RemoteControl.SendMessageToProcess.vi"("error in (no error)"=w1472, "SendMessageToProcess"=w1469, "RemoteControl"=w1474) -> ("error out"=w1471:errorcluster)  [unwired: 7 in, 1 out]
            n693 = call <vilib>:"Add State(s) to Queue__jki_lib_state_machine.vi"("State(s) in (\"\")"=w1477) -> ("States Out"=w1476:string)  [unwired: 14 in]
          }
          frame "DONE: Stop Remote" {
            # "#done\n#framework"
            n694 = Unbundle By Name(w1480) -> ("RemoteControl"=w1484:refnum<class "RemoteControl.lvclass">)
            n695 = call <vilib>:"GetState.vi"("error in (no error)"=w1482, "SMO"=w1484) -> ("SMO State"=w1478:T10, "SMO out"=w1483:refnum<class "RemoteControl.lvclass">)  [unwired: 7 in, 1 out]
            n696 = case shown="Default" w1478 {
              tunnel: [w1487 w1492] -> w1479
              tunnel: w1483 -> [_ w1495]
              tunnel: w1482 -> [w1487 w1494]
              frame "Stopped" {
              }
              frame Default {
                n697 = call <vilib>:"Stop.vi"("error in (no error)"=w1494, "SMO"=w1495) -> ("error out"=w1491:errorcluster, "SMO out"=w1490:refnum<class "RemoteControl.lvclass">)  [unwired: 8 in]
                n698 = call <vilib>:"GetState.vi"("error in (no error)"=w1491, "SMO"=w1490) -> ("error out"=w1489:errorcluster, "SMO out"=w1488:refnum<class "RemoteControl.lvclass">)  [unwired: 7 in, 1 out]
                n699 = call <vilib>:"Destroy.vi"("error in (no error)"=w1489, "SMO"=w1488) -> ("error out"=w1493:errorcluster)  [unwired: 9 in]
                n700 = call <vilib>:"Clear Errors.vi"("error in (no error)"=w1493) -> ("error out"=w1492:errorcluster)  [unwired: 5 in, 1 out]
              }
            }
            n701 = call <vilib>:"Add State(s) to Queue__jki_lib_state_machine.vi"("State(s) in (\"\")"=w1486) -> ("States Out"=w1485:string)  [unwired: 14 in]
          }
          frame "DONE: Create" {
            # "#done\n#framework"
            # "#done"
            n702 = Unbundle By Name(w1498) -> ("Lockin.DAQ"=w1506:refnum<class "Instrument.DAQ.lvclass">)
            n703 = call <vilib>:"GetState.vi"("error in (no error)"=w1496, "SMO"=w1506) -> ("error out"=w1500:errorcluster, "SMO State"=w1505:T10, "SMO out"=w1503:refnum<class "Instrument.DAQ.lvclass">)  [unwired: 7 in]
            n704 = call <vilib>:"Clear Errors.vi"("error in (no error)"=w1500) -> ("error out"=w1504:errorcluster)  [unwired: 5 in, 1 out]
            n705 = case shown="Default" w1505 {
              tunnel: [w1510 w1511] -> w1499
              tunnel: w1504 -> [w1510 w1514]
              tunnel: w1503 -> [w1509 w1513]
              tunnel: [w1509 w1512] -> w1501
              frame "Created".."Stopped" {
              }
              frame Default {
                n706 = call <vilib>:"Create.vi"("error in (no error)"=w1514, "SMO"=w1513) -> ("error out"=w1511:errorcluster, "SMO out"=w1512:refnum<class "Instrument.DAQ.lvclass">)  [unwired: 7 in, 1 out]
              }
            }
            n707 = Bundle By Name(cluster=w1498, "Lockin.DAQ"=w1501) -> (w1497:T44)
            n708 = call <vilib>:"Add State(s) to Queue__jki_lib_state_machine.vi"("State(s) in (\"\")"=w1508) -> ("States Out"=w1507:string)  [unwired: 14 in]
          }
          frame "DONE: Start" {
            # "#done\n#framework"
            # "#done"
            n709 = Unbundle By Name(w1515) -> ("Lockin.DAQ"=w1525:refnum<class "Instrument.DAQ.lvclass">)
            n710 = call <vilib>:"GetState.vi"("error in (no error)"=w1519, "SMO"=w1525) -> ("error out"=w1517:errorcluster, "SMO State"=w1524:T10, "SMO out"=w1523:refnum<class "Instrument.DAQ.lvclass">)  [unwired: 7 in]
            n711 = call <vilib>:"Clear Errors.vi"("error in (no error)"=w1517) -> ("error out"=w1518:errorcluster)  [unwired: 5 in, 1 out]
            n712 = case shown="Default" w1524 {
              tunnel: [w1529 w1533] -> w1520
              tunnel: w1518 -> [w1529 w1532]
              tunnel: w1523 -> [w1528 w1531]
              tunnel: [w1528 w1530] -> w1521
              frame "Started" {
              }
              frame Default {
                n713 = call <vilib>:"Start.vi"("error in (no error)"=w1532, "SMO"=w1531) -> ("error out"=w1533:errorcluster, "SMO out"=w1530:refnum<class "Instrument.DAQ.lvclass">)  [unwired: 8 in]
              }
            }
            n714 = Bundle By Name(cluster=w1515, "Lockin.DAQ"=w1521) -> (w1516:T44)
            n715 = call <vilib>:"Add State(s) to Queue__jki_lib_state_machine.vi"("State(s) in (\"\")"=w1527) -> ("States Out"=w1526:string)  [unwired: 14 in]
          }
          frame "DONE: Set State" {
            # "#done\n#framework"
            # "#done"
            n716 = Unbundle By Name(w1534) -> ("Lockin.DAQ"=w1540:refnum<class "Instrument.DAQ.lvclass">)
            n717 = case shown="\"stop sweep\"" w1536 {
              tunnel: [T15."stop" ("State") T15."start" ("State") T15."reset" ("State") T15."start sweep" ("State") T15."stop sweep" ("State")] -> w1535
              tunnel: [FALSE ("Trigger") TRUE ("Trigger") w1548 TRUE ("Trigger") TRUE ("Trigger")] -> w1537
              frame "stop", Default {
              }
              frame "start" {
              }
              frame "reset" {
                n718 = local read "Start"() -> (w1548:bool)
              }
              frame "start sweep" {
              }
              frame "stop sweep" {
              }
            }
            n719 = local write "Start"(w1537) -> ()
            n720 = call <userlib>:"Lockin.DAQ.setstate.vi"("error in (no error)"=w1539, "State"=w1535, "Lockin.DAQ"=w1540) -> ("error out"=w1538:errorcluster)  [unwired: 7 in, 1 out]
            n721 = call <vilib>:"Add State(s) to Queue__jki_lib_state_machine.vi"("State(s) in (\"\")"=w1543) -> ("States Out"=w1542:string)  [unwired: 14 in]
          }
          frame "DONE: Set AI Config" {
            # "#done\n#framework"
            # "#done"
            n722 = Unbundle By Name(w1555) -> ("Lockin.DAQ"=w1560:refnum<class "Instrument.DAQ.lvclass">, "Lockin"=w1556:refnum<class "Instrument.Lockin.lvclass">)
            n723 = Unbundle By Name(w1556) -> ("AI"=w1557:T50)
            n724 = call <userlib>:"Lockin.DAQ.setAIconfig.vi"("error in (no error)"=w1559, "Simulation mode"="AI Simulation mode", "AI Configuration"=w1557, "Lockin.DAQ"=w1560) -> ("error out"=w1558:errorcluster)  [unwired: 6 in, 1 out]
            n725 = call <vilib>:"Add State(s) to Queue__jki_lib_state_machine.vi"("State(s) in (\"\")"=w1563) -> ("States Out"=w1562:string)  [unwired: 14 in]
          }
          frame "DONE: Set AO Config" {
            # "#done\n#framework"
            # "#done"
            n726 = Unbundle By Name(w1565) -> ("Lockin.DAQ"=w1569:refnum<class "Instrument.DAQ.lvclass">, "Lockin"=w1566:refnum<class "Instrument.Lockin.lvclass">)
            n727 = Unbundle By Name(w1566) -> ("AO"=w1564:T46)
            n728 = call <userlib>:"Lockin.DAQ.setAOconfig.vi"("error in (no error)"=w1568, "AO Configuration"=w1564, "Lockin.DAQ"=w1569) -> ("error out"=w1567:errorcluster)  [unwired: 7 in, 1 out]
            n729 = call <vilib>:"Add State(s) to Queue__jki_lib_state_machine.vi"("State(s) in (\"\")"=w1572) -> ("States Out"=w1571:string)  [unwired: 14 in]
          }
          frame "DONE: Set AO" {
            # "#done\n#framework"
            # "#done"
            n730 = Unbundle By Name(w1578) -> ("Lockin.DAQ"=w1577:refnum<class "Instrument.DAQ.lvclass">, "Lockin"=w1574:refnum<class "Instrument.Lockin.lvclass">)
            n731 = Unbundle By Name(w1574) -> ("AO"=w1573:T81)
            n732 = call <userlib>:"Lockin.DAQ.setAO.vi"("error in (no error)"=w1576, "AO Channels"=w1573, "Lockin.DAQ"=w1577) -> ("error out"=w1575:errorcluster)  [unwired: 7 in, 1 out]
            n733 = call <vilib>:"Add State(s) to Queue__jki_lib_state_machine.vi"("State(s) in (\"\")"=w1581) -> ("States Out"=w1580:string)  [unwired: 14 in]
          }
          frame "DONE: Set REF" {
            # "#done\n#framework"
            # "#done"
            n734 = Unbundle By Name(w1584) -> ("Lockin.DAQ"=w1587:refnum<class "Instrument.DAQ.lvclass">, "Lockin"=w1585:refnum<class "Instrument.Lockin.lvclass">)
            n735 = Unbundle By Name(w1585) -> ("REF"=w1582:T83)
            n736 = call <userlib>:"Lockin.DAQ.setREF.vi"("error in (no error)"=w1583, "Channels: Lockin"=w1582, "Lockin.DAQ"=w1587) -> ("error out"=w1586:errorcluster)  [unwired: 7 in, 1 out]
            n737 = call <vilib>:"Add State(s) to Queue__jki_lib_state_machine.vi"("State(s) in (\"\")"=w1590) -> ("States Out"=w1589:string)  [unwired: 14 in]
          }
          frame "DONE: Set AI" {
            # "#done\n#framework"
            # "#done"
            n738 = Unbundle By Name(w1595) -> ("Lockin.DAQ"=w1594:refnum<class "Instrument.DAQ.lvclass">, "Lockin"=w1596:refnum<class "Instrument.Lockin.lvclass">)
            n739 = Unbundle By Name(w1596) -> ("AI"=w1591:T77)
            n740 = call <userlib>:"Lockin.DAQ.setAI.vi"("error in (no error)"=w1593, "AI Channels"=w1591, "Lockin.DAQ"=w1594) -> ("error out"=w1592:errorcluster)  [unwired: 7 in, 1 out]
            n741 = call <vilib>:"Add State(s) to Queue__jki_lib_state_machine.vi"("State(s) in (\"\")"=w1599) -> ("States Out"=w1598:string)  [unwired: 14 in]
          }
          frame "DONE: Set Input Gain" {
            # "#done\n#framework"
            # "#done"
            n742 = Unbundle By Name(w1600) -> ("Lockin.DAQ"=w1605:refnum<class "Instrument.DAQ.lvclass">, "Lockin"=w1603:refnum<class "Instrument.Lockin.lvclass">)
            n743 = Unbundle By Name(w1603) -> ("AI.Gain"=w1602:T40)
            n744 = call <userlib>:"Lockin.DAQ.setInputGain.vi"("error in (no error)"=w1601, "setInputGain"=w1602, "Lockin.DAQ"=w1605) -> ("error out"=w1604:errorcluster)  [unwired: 7 in, 1 out]
            n745 = call <vilib>:"Add State(s) to Queue__jki_lib_state_machine.vi"("State(s) in (\"\")"=w1608) -> ("States Out"=w1607:string)  [unwired: 14 in]
          }
          frame "DONE: Set Output Gain" {
            # "#done\n#framework"
            # "#done"
            n746 = Unbundle By Name(w1613) -> ("Lockin.DAQ"=w1612:refnum<class "Instrument.DAQ.lvclass">, "Lockin"=w1614:refnum<class "Instrument.Lockin.lvclass">)
            n747 = Unbundle By Name(w1614) -> ("AO.Gain"=w1610:T40)
            n748 = call <userlib>:"Lockin.DAQ.setOutputGain.vi"("error in (no error)"=w1611, "setOutputGain"=w1610, "Lockin.DAQ"=w1612) -> ("error out"=w1609:errorcluster)  [unwired: 7 in, 1 out]
            n749 = call <vilib>:"Add State(s) to Queue__jki_lib_state_machine.vi"("State(s) in (\"\")"=w1617) -> ("States Out"=w1616:string)  [unwired: 14 in]
          }
          frame "DONE: Set Prefilter" {
            # "#done\n#framework"
            # "#done"
            n750 = Unbundle By Name(w1620) -> ("Lockin.DAQ"=w1622:refnum<class "Instrument.DAQ.lvclass">, "Lockin"=w1623:refnum<class "Instrument.Lockin.lvclass">)
            n751 = Unbundle By Name(w1623) -> ("Prefilter"=w1621:T85)
            n752 = call <userlib>:"Lockin.DAQ.setPreFilter.vi"("error in (no error)"=w1619, "PreFilter"=w1621, "Lockin.DAQ"=w1622) -> ("error out"=w1618:errorcluster)  [unwired: 7 in, 1 out]
            n753 = call <vilib>:"Add State(s) to Queue__jki_lib_state_machine.vi"("State(s) in (\"\")"=w1626) -> ("States Out"=w1625:string)  [unwired: 14 in]
          }
          frame "DONE: Calibration" {
            # "#done\n#framework"
            # "#done"
            # "This will only get the current calibration inf\nActually doing calibration is done via Set State >> Calibration"
            n754 = Unbundle By Name(w1632) -> ("Lockin.DAQ"=w1631:refnum<class "Instrument.DAQ.lvclass">)
            n755 = case shown="\"False\", Default" w1627 {
              tunnel: [FALSE ("setCalibration") TRUE ("setCalibration")] -> w1628
              frame "False", Default {
                # "check calibration"
              }
              frame "True" {
                # "calibrate"
              }
            }
            n756 = call <userlib>:"Lockin.DAQ.setCalibration.vi"("error in (no error)"=w1630, "setCalibration"=w1628, "Lockin.DAQ"=w1631) -> ("error out"=w1629:errorcluster)  [unwired: 7 in, 1 out]
            n757 = call <vilib>:"Add State(s) to Queue__jki_lib_state_machine.vi"("State(s) in (\"\")"=w1635) -> ("States Out"=w1634:string)  [unwired: 14 in]
          }
          frame "DONE: Auto DAQ" {
            # "#done\n#framework"
            # "#done"
            n758 = Unbundle By Name(w1641) -> ("Lockin.DAQ"=w1640:refnum<class "Instrument.DAQ.lvclass">)
            n759 = call <userlib>:"Lockin.DAQ.autoConfigureDAQ.vi"("error in (no error)"=w1639, "Lockin.DAQ"=w1640) -> ("error out"=w1638:errorcluster)  [unwired: 8 in, 1 out]
            n760 = call <vilib>:"Add State(s) to Queue__jki_lib_state_machine.vi"("State(s) in (\"\")"=w1644) -> ("States Out"=w1643:string)  [unwired: 14 in]
          }
          frame "DONE: Reset Phase" {
            # "#done\n#framework"
            # "#done"
            n761 = Unbundle By Name(w1649) -> ("Lockin.DAQ"=w1648:refnum<class "Instrument.DAQ.lvclass">)
            n762 = call <userlib>:"Lockin.DAQ.ResetPhase.vi"("error in (no error)"=w1647, "Reset Phase"=TRUE, "Lockin.DAQ"=w1648) -> ("error out"=w1646:errorcluster)  [unwired: 7 in, 1 out]
            n763 = call <vilib>:"Add State(s) to Queue__jki_lib_state_machine.vi"("State(s) in (\"\")"=w1652) -> ("States Out"=w1651:string)  [unwired: 14 in]
          }
          frame "DONE: Measure Offset" {
            # "#done\n#framework"
            # "#done"
            n764 = Unbundle By Name(w1653) -> ("Lockin.DAQ"=w1657:refnum<class "Instrument.DAQ.lvclass">)
            n765 = call <userlib>:"Lockin.DAQ.measureOffset.vi"("error in (no error)"=w1655, "measureOffset"=TRUE, "Lockin.DAQ"=w1657) -> ("error out"=w1654:errorcluster)  [unwired: 7 in, 1 out]
            n766 = call <vilib>:"Add State(s) to Queue__jki_lib_state_machine.vi"("State(s) in (\"\")"=w1660) -> ("States Out"=w1659:string)  [unwired: 14 in]
          }
          frame "DONE: Remove Offset" {
            # "#done\n#framework"
            # "#done"
            n767 = Unbundle By Name(w1661) -> ("Lockin.DAQ"=w1665:refnum<class "Instrument.DAQ.lvclass">)
            n768 = call <userlib>:"Lockin.DAQ.zeroOffset.vi"("error in (no error)"=w1662, "zeroOffset"=TRUE, "Lockin.DAQ"=w1665) -> ("error out"=w1664:errorcluster)  [unwired: 7 in, 1 out]
            n769 = call <vilib>:"Add State(s) to Queue__jki_lib_state_machine.vi"("State(s) in (\"\")"=w1668) -> ("States Out"=w1667:string)  [unwired: 14 in]
          }
          frame "DONE: Stop" {
            # "#done\n#framework"
            # "#done"
            n770 = Unbundle By Name(w1669) -> ("Lockin.DAQ"=w1671:refnum<class "Instrument.DAQ.lvclass">)
            n771 = call <userlib>:"Lockin.DAQ.setstate.vi"("error in (no error)"=w1672, "State"=T15."stop", "Lockin.DAQ"=w1671) -> ("error out"=w1674:errorcluster, "Lockin.DAQ out"=w1673:refnum<class "Lockin.DAQ.lvclass">)  [unwired: 7 in]
            n772 = call <vilib>:"GetState.vi"("error in (no error)"=w1674, "SMO"=w1673) -> ("SMO State"=w1676:T10, "SMO out"=w1677:refnum<class "SMO.lvclass">)  [unwired: 7 in, 1 out]
            n773 = case shown="Default" w1676 {
              tunnel: [w1681 w1687] -> w1678
              tunnel: w1677 -> [_ w1690]
              tunnel: w1674 -> [w1681 w1689]
              frame "Stopped" {
              }
              frame Default {
                n774 = call <vilib>:"Stop.vi"("error in (no error)"=w1689, "SMO"=w1690) -> ("error out"=w1686:errorcluster, "SMO out"=w1685:refnum<class "SMO.lvclass">)  [unwired: 8 in]
                n775 = call <vilib>:"GetState.vi"("error in (no error)"=w1686, "SMO"=w1685) -> ("error out"=w1684:errorcluster, "SMO State"=w1682:T10, "SMO out"=w1683:refnum<class "SMO.lvclass">)  [unwired: 7 in]
                n776 = local write "LockinDAQ SMO State"(w1682) -> ()
                n777 = call <vilib>:"Destroy.vi"("error in (no error)"=w1684, "SMO"=w1683) -> ("error out"=w1688:errorcluster)  [unwired: 9 in]
                n778 = call <vilib>:"Clear Errors.vi"("error in (no error)"=w1688) -> ("error out"=w1687:errorcluster)  [unwired: 5 in, 1 out]
              }
            }
            n779 = call <vilib>:"Add State(s) to Queue__jki_lib_state_machine.vi"("State(s) in (\"\")"=w1680) -> ("States Out"=w1679:string)  [unwired: 14 in]
          }
          frame "DONE: Initialize CONFIG" {
            # "#done\nuses config #framework"
            n780 = Unbundle By Name(w1691) -> ("Lockin"=w1697:refnum<class "Instrument.Lockin.lvclass">)
            n781 = call-dynamic "Get SMO Name.vi"("error in (no error)"=w1692, "Instrument.Lockin"=w1697) -> ("error out"=w1694:errorcluster, "SMO Name"=w1698:string, "Instrument.Lockin out"=w1699:refnum<class "Instrument.Lockin.lvclass">)  [unwired: 7 in]
            n782 = call <userlib>:"Write Configuration Path.vi"("error in (no error)"=w1694, "name or relative path"=w1698, "Instrument in"=w1699) -> ("error out"=w1693:errorcluster, "Instrument out"=w1695:refnum<class "Instrument.Lockin.lvclass">)  [unwired: 7 in]
            n783 = Bundle By Name(cluster=w1691, "Lockin"=w1695) -> (w1696:T44)
            n784 = call <vilib>:"Add State(s) to Queue__jki_lib_state_machine.vi"("State(s) in (\"\")"=w1702) -> ("States Out"=w1701:string)  [unwired: 14 in]
          }
          frame "DONE: Write CONFIG" {
            # "#done\nuses config #framework"
            n785 = Unbundle By Name(w1703) -> ("Lockin"=w1705:refnum<class "Instrument.Lockin.lvclass">)
            n786 = call-dynamic "Write Configuration File.vi"("error in (no error)"=w1704, "Instrument.Lockin"=w1705) -> ("error out"=w1706:errorcluster)  [unwired: 8 in, 1 out]
            n787 = disable-structure shown="Disabled" {
              disable-tunnel: [w1712 w1713] -> w1707
              disable-tunnel: w1706 -> [w1711 w1713]
              frame Disabled {
                n788 = call <userlib>:"write_lockin_FP_DSC.vi"("error in (no error)"=w1711) -> ("error out"=w1712:errorcluster)  [unwired: 10 in]
              }
              frame Enabled {
              }
            }
            n789 = call <vilib>:"Add State(s) to Queue__jki_lib_state_machine.vi"("State(s) in (\"\")"=w1709) -> ("States Out"=w1710:string)  [unwired: 14 in]
          }
          frame "DONE: Read CONFIG" {
            # "#done\nuses config #framework"
            # "Do not write values to FP if error. Eg, if file ini file does not exist yet."
            n790 = Unbundle By Name(w1717) -> ("Lockin"=w1722:refnum<class "Instrument.Lockin.lvclass">)
            n791 = disable-structure shown="Disabled" {
              disable-tunnel: w1723 -> [w1742 _]
              frame Disabled {
                n792 = call <userlib>:"read_lockin_FP_DSC.vi"("error in (no error)"=w1742) -> ()  [unwired: 9 in, 2 out]
              }
              frame Enabled {
              }
            }
            n793 = call-dynamic "Read Configuration File.vi"("error in (no error)"=w1723, "Instrument.Lockin"=w1722) -> ("error out"=w1721:errorcluster, "Instrument.Lockin out"=w1720:refnum<class "Instrument.Lockin.lvclass">)  [unwired: 8 in]
            n794 = call <userlib>:"Lockin.Read Configuration.vi"("error in (no error)"=w1721, "Instrument.Lockin"=w1720) -> ("error out"=w1718:errorcluster, "Configuration"=w1719:T86, "Instrument.Lockin out"=w1716:refnum<class "Instrument.Lockin.lvclass">)  [unwired: 7 in]
            n795 = case shown="No Error" w1718 {
              selector: w1718 -> [w1736 w1741]
              tunnel: w1719 -> [w1738 _]
              tunnel: [w1736 w1740] -> w1724
              tunnel: ["" ("State(s) in Front (\"\")") "//DONE: Write CONFIG" ("State(s) in Front (\"\")")] -> w1714
              frame No Error {
                n796 = Unbundle By Name(w1738) -> ("AI Configuration"=w1731:T92, "AO Configuration"=w1730:T95, "AO Channels"=w1734:T54, "REF Channels"=w1733:T57, "Calibration.Cal Info"=w1737:T63[], "DAQ.sampling"=w1732:T91, "Aux Channel"=w1728:tag)  [unwired: 6 out]
                n797 = local write "REF Channels"(w1733) -> ()
                n798 = call "config not UI to UI (AO and AI).vi"("AO Config"=w1730, "AI Config"=w1731) -> ("New Ch []"=w1729:T98[])  [unwired: 8 in, 1 out]
                n799 = local write "Sampling"(w1732) -> ()
                n800 = local write "DAQ Config"(w1729) -> ()
                n801 = local write "AO Channels"(w1734) -> ()
                n802 = local write "Aux Channel"(w1728) -> ()
                n803 = local write "Cal Info"(w1737) -> ()
              }
              frame Error {
                # "If error, file might not exist. Try to write it."
                n804 = call <vilib>:"Clear Errors.vi"("error in (no error)"=w1741) -> ("error out"=w1740:errorcluster)  [unwired: 5 in, 1 out]
              }
            }
            n805 = Bundle By Name(cluster=w1717, "Lockin"=w1716) -> (w1715:T44)
            n806 = call <vilib>:"Add State(s) to Queue__jki_lib_state_machine.vi"("State(s) in Front (\"\")"=w1714, "State(s) in (\"\")"=w1726) -> ("States Out"=w1727:string)  [unwired: 13 in]
          }
          frame "Command: Handle Command" {
            # "#done"
            n807 = Unbundle By Name(w1744) -> ("Lockin"=w1753:refnum<class "Instrument.Lockin.lvclass">, "Message.Command"=w1751:string, "Message.Data"=w1750:variant, "Message.ID"=w1749:string)
            n808 = call-dynamic "Handle Command.vi"("error in (no error)"=w1746, "Data"=w1750, "Command"=w1751, "Instrument.Lockin"=w1753) -> ("error out"=w1745:errorcluster, "Processed Data"=w1748:variant, "Command"=w1747:string, "Instrument.Lockin out"=w1752:refnum<class "Instrument.Lockin.lvclass">)  [unwired: 4 in]
            n809 = Bundle By Name(cluster=w1744, "Lockin"=w1752, "HandledMessage.Command"=w1747, "HandledMessage.Data"=w1748, "HandledMessage.ID"=w1749) -> (w1743:T44)
            n810 = call <vilib>:"Add State(s) to Queue__jki_lib_state_machine.vi"("State(s) in (\"\")"=w1756) -> ("States Out"=w1755:string)  [unwired: 14 in]
          }
          frame "Command: getAOconfig" {
            # "#done"
            n811 = call <vilib>:"Add State(s) to Queue__jki_lib_state_machine.vi"("State(s) in Front (\"\")"="Command: Handle Command" ("State(s) in Front (\"\")"), "State(s) in (\"\")"=w1762) -> ("States Out"=w1761:string)  [unwired: 13 in]
          }
          frame "Command: getSampling" {
            # "#done"
            n812 = call <vilib>:"Add State(s) to Queue__jki_lib_state_machine.vi"("State(s) in Front (\"\")"="Command: Handle Command" ("State(s) in Front (\"\")"), "State(s) in (\"\")"=w1768) -> ("States Out"=w1767:string)  [unwired: 13 in]
          }
          frame "Command: getREFconfig" {
            # "#done"
            # "Simply respond with data on data cluster"
            n813 = call <vilib>:"Add State(s) to Queue__jki_lib_state_machine.vi"("State(s) in Front (\"\")"="Command: Handle Command" ("State(s) in Front (\"\")"), "State(s) in (\"\")"=w1774) -> ("States Out"=w1773:string)  [unwired: 13 in]
          }
          frame "Command: getInputGain" {
            # "#done"
            # "Simply respond with data on data cluster"
            n814 = call <vilib>:"Add State(s) to Queue__jki_lib_state_machine.vi"("State(s) in Front (\"\")"="Command: Handle Command" ("State(s) in Front (\"\")"), "State(s) in (\"\")"=w1780) -> ("States Out"=w1779:string)  [unwired: 13 in]
          }
          frame "Command: getOutputGain" {
            # "#done"
            # "Simply respond with data on data cluster"
            n815 = call <vilib>:"Add State(s) to Queue__jki_lib_state_machine.vi"("State(s) in Front (\"\")"="Command: Handle Command" ("State(s) in Front (\"\")"), "State(s) in (\"\")"=w1786) -> ("States Out"=w1785:string)  [unwired: 13 in]
          }
          frame "Command: getAO" {
            # "#done"
            # "Simply respond with data on data cluster"
            n816 = call <vilib>:"Add State(s) to Queue__jki_lib_state_machine.vi"("State(s) in Front (\"\")"="Command: Handle Command" ("State(s) in Front (\"\")"), "State(s) in (\"\")"=w1792) -> ("States Out"=w1791:string)  [unwired: 13 in]
          }
          frame "Command: getAI" {
            # "#done"
            # "Simply respond with data on data cluster"
            n817 = call <vilib>:"Add State(s) to Queue__jki_lib_state_machine.vi"("State(s) in Front (\"\")"="Command: Handle Command" ("State(s) in Front (\"\")"), "State(s) in (\"\")"=w1798) -> ("States Out"=w1797:string)  [unwired: 13 in]
          }
          frame "Command: getResults" {
            # "#done"
            # "Simply respond with data on data cluster"
            n818 = call <vilib>:"Add State(s) to Queue__jki_lib_state_machine.vi"("State(s) in Front (\"\")"="Command: Handle Command" ("State(s) in Front (\"\")"), "State(s) in (\"\")"=w1804) -> ("States Out"=w1803:string)  [unwired: 13 in]
          }
          frame "Command: HELP" {
            # "#done"
            # "Simply respond with data on data cluster"
            n819 = call <vilib>:"Add State(s) to Queue__jki_lib_state_machine.vi"("State(s) in Front (\"\")"="Command: Handle Command" ("State(s) in Front (\"\")"), "State(s) in (\"\")"=w1810) -> ("States Out"=w1809:string)  [unwired: 13 in]
          }
          frame "Command: ACK" {
            # "#done"
            # "Simply respond with data on data cluster"
            n820 = call <vilib>:"Add State(s) to Queue__jki_lib_state_machine.vi"("State(s) in Front (\"\")"="Command: Handle Command" ("State(s) in Front (\"\")"), "State(s) in (\"\")"=w1816) -> ("States Out"=w1815:string)  [unwired: 13 in]
          }
          frame "Command: NOT HANDLED COMMANDS" {
            # "#done"
            n821 = call <vilib>:"Add State(s) to Queue__jki_lib_state_machine.vi"("State(s) in (\"\")"=w1821) -> ("States Out"=w1820:string)  [unwired: 14 in]
          }
          frame "Command: getAll" {
            # "#done"
            n822 = Unbundle By Name(w1822) -> ("Message"=w1824:T43)
            n823 = Bundle By Name(cluster=w1824, "Data"="Not Supported" ("Not Supported")) -> (w1823:T43)
            n824 = Bundle By Name(cluster=w1822, "HandledMessage"=w1823) -> (w1826:T44)
            n825 = call <vilib>:"Add State(s) to Queue__jki_lib_state_machine.vi"("State(s) in (\"\")"=w1830) -> ("States Out"=w1829:string)  [unwired: 14 in]
          }
          frame "Command: getTrigger" {
            # "#done"
            # "Simply respond with data on data cluster"
            n826 = Unbundle By Name(w1835) -> ("Message"=w1833:T43)
            n827 = local read "Trigger"() -> (w1836:bool)
            n828 = To Variant(anything=w1836) -> (Variant=w1834:variant)
            n829 = Bundle By Name(cluster=w1833, "Data"=w1834) -> (w1831:T43)
            n830 = Bundle By Name(cluster=w1835, "HandledMessage"=w1831) -> (w1832:T44)
            n831 = call <vilib>:"Add State(s) to Queue__jki_lib_state_machine.vi"("State(s) in (\"\")"=w1840) -> ("States Out"=w1839:string)  [unwired: 14 in]
          }
          frame "Command: getStatus" {
            # "#done"
            # "Simply respond with data on data cluster"
            n832 = Unbundle By Name(w1841) -> ("Message"=w1842:T43, "DAQ state"=w1843:T45)
            n833 = To Variant(anything=w1843) -> (Variant=w1844:variant)
            n834 = Bundle By Name(cluster=w1842, "Data"=w1844) -> (w1846:T43)
            n835 = Bundle By Name(cluster=w1841, "HandledMessage"=w1846) -> (w1845:T44)
            n836 = call <vilib>:"Add State(s) to Queue__jki_lib_state_machine.vi"("State(s) in (\"\")"=w1850) -> ("States Out"=w1849:string)  [unwired: 14 in]
          }
          frame "Command: getSweepResults" {
            # "#done"
            # "Simply respond with data on data cluster"
            n837 = Unbundle By Name(w1851) -> ("Message"=w1854:T43, "SweepResults"=w1855:T71)
            n838 = To Variant(anything=w1855) -> (Variant=w1857:variant)
            n839 = Bundle By Name(cluster=w1854, "Data"=w1857) -> (w1852:T43)
            n840 = Bundle By Name(cluster=w1851, "HandledMessage"=w1852) -> (w1853:T44)
            n841 = call <vilib>:"Add State(s) to Queue__jki_lib_state_machine.vi"("State(s) in (\"\")"=w1860) -> ("States Out"=w1859:string)  [unwired: 14 in]
          }
          frame "Command: getSweepWaveforms" {
            # "#done"
            # "Simply respond with data on data cluster"
            n842 = Unbundle By Name(w1861) -> ("Message"=w1863:T43, "SweepWaveforms"=w1865:T70)
            n843 = To Variant(anything=w1865) -> (Variant=w1867:variant)
            n844 = Bundle By Name(cluster=w1863, "Data"=w1867) -> (w1864:T43)
            n845 = Bundle By Name(cluster=w1861, "HandledMessage"=w1864) -> (w1862:T44)
            n846 = call <vilib>:"Add State(s) to Queue__jki_lib_state_machine.vi"("State(s) in (\"\")"=w1870) -> ("States Out"=w1869:string)  [unwired: 14 in]
          }
          frame "Command: getIVmode" {
            # "#done"
            # "Simply respond with data on data cluster"
            n847 = Unbundle By Name(w1871) -> ("Message"=w1874:T43)
            n848 = local read "Pause"() -> (w1876:bool)
            n849 = To Variant(anything=w1876) -> (Variant=w1875:variant)
            n850 = Bundle By Name(cluster=w1874, "Data"=w1875) -> (w1873:T43)
            n851 = Bundle By Name(cluster=w1871, "HandledMessage"=w1873) -> (w1872:T44)
            n852 = call <vilib>:"Add State(s) to Queue__jki_lib_state_machine.vi"("State(s) in (\"\")"=w1880) -> ("States Out"=w1879:string)  [unwired: 14 in]
          }
          frame "Command: getAutoSampling" {
            # "#todo"
            n853 = Unbundle By Name(w1884) -> ("Message"=w1883:T43)
            n854 = local read "Sampling Mode"() -> (w1887:enum16{"Manual", "Auto Fs", "Max Fs"})
            n855 = To Variant(anything=w1887) -> (Variant=w1885:variant)
            n856 = Bundle By Name(cluster=w1883, "Data"=w1885) -> (w1882:T43)
            n857 = Bundle By Name(cluster=w1884, "HandledMessage"=w1882) -> (w1881:T44)
            n858 = call <vilib>:"Add State(s) to Queue__jki_lib_state_machine.vi"("State(s) in (\"\")"=w1890) -> ("States Out"=w1889:string)  [unwired: 14 in]
          }
          frame "Command: getRefreshTime" {
            # "#done"
            n859 = Unbundle By Name(w1895) -> ("Message"=w1893:T43)
            n860 = local read "Refresh time (ms)"() -> (w1894:u32)
            n861 = To Variant(anything=w1894) -> (Variant=w1896:variant)
            n862 = Bundle By Name(cluster=w1893, "Data"=w1896) -> (w1892:T43)
            n863 = Bundle By Name(cluster=w1895, "HandledMessage"=w1892) -> (w1891:T44)
            n864 = call <vilib>:"Add State(s) to Queue__jki_lib_state_machine.vi"("State(s) in (\"\")"=w1900) -> ("States Out"=w1899:string)  [unwired: 14 in]
          }
          frame "Command: setAO_Amplitude" {
            # "#done"
            # "Convert Data from Message\nto appropriate data type"
            # "Triggers User Event to update front panel\nand put data onto class wire"
            n865 = Unbundle By Name(w1910) -> ("Message"=w1908:T43, "Lockin"=w1914:refnum<class "Instrument.Lockin.lvclass">, "Message.Command"=w1904:string, "Message.Data"=w1905:variant)
            n866 = call "Variant to LV Data.vim"("type"=T21 {"AO Channel"=5, "Amplitude (V)"=0.0} ("setAO_Amp"), "error in (no error)"=w1903, "JSON Data in"=w1905, "Command"=w1904) -> ("error out"=w1902:errorcluster, "Data out"=w1901:T21)  [unwired: 4 in, 2 out]
            n867 = Unbundle By Name(w1901) -> ("AO Channel"=w1918:i32, "Amplitude (V)"=w1917:dbl)
            n868 = call "Update AO Parameter.vi"("Parameter"=T22."Amplitude", "error in"=w1902, "Value"=w1917, "Channel"=w1918, "Instrument.Lockin"=w1914) -> ("error out"=w1915:errorcluster, 2:w1913, "Instrument.Lockin out"=w1912:refnum<class "Instrument.Lockin.lvclass">)  [unwired: 4 in]
            n869 = property on="AO Channels" class="Arr (strict)"(error in=w1915, "Val(Sgnl)"=w1913) -> (error out=w1907:errorcluster)  [unwired: 1 in, 1 out]
            n870 = To Variant(anything=w1913) -> (Variant=w1919:variant)
            n871 = Bundle By Name(cluster=w1908, "Data"=w1919) -> (w1909:T43)
            n872 = Bundle By Name(cluster=w1910, "HandledMessage"=w1909, "Lockin"=w1912) -> (w1911:T44)
            n873 = call <vilib>:"Add State(s) to Queue__jki_lib_state_machine.vi"("State(s) in (\"\")"=w1922) -> ("States Out"=w1921:string)  [unwired: 14 in]
          }
          frame "Command: setAO_DC" {
            # "#done"
            # "Convert Data from Message\nto appropriate data type"
            # "Triggers User Event to update front panel\nand put data onto class wire"
            n874 = Unbundle By Name(w1932) -> ("Message"=w1930:T43, "Lockin"=w1936:refnum<class "Instrument.Lockin.lvclass">, "Message.Command"=w1924:string, "Message.Data"=w1925:variant)
            n875 = call "Variant to LV Data.vim"("type"=T23 {"AO Channel"=5, "DC (V)"=0.0} ("setAO_DC"), "error in (no error)"=w1927, "JSON Data in"=w1925, "Command"=w1924) -> ("error out"=w1926:errorcluster, "Data out"=w1923:T23)  [unwired: 4 in, 2 out]
            n876 = Unbundle By Name(w1923) -> ("AO Channel"=w1940:i32, "DC (V)"=w1939:dbl)
            n877 = call "Update AO Parameter.vi"("Parameter"=T22."DC", "error in"=w1926, "Value"=w1939, "Channel"=w1940, "Instrument.Lockin"=w1936) -> ("error out"=w1937:errorcluster, "Instrument.Lockin out"=w1934:refnum<class "Instrument.Lockin.lvclass">)  [unwired: 5 in]
            n878 = property on="AO Channels" class="Arr (strict)"(error in=w1937) -> (error out=w1929:errorcluster, "Val(Sgnl)"=w1935:T3)  [unwired: 1 in, 1 out]
            n879 = To Variant(anything=w1935) -> (Variant=w1941:variant)
            n880 = Bundle By Name(cluster=w1930, "Data"=w1941) -> (w1931:T43)
            n881 = Bundle By Name(cluster=w1932, "HandledMessage"=w1931, "Lockin"=w1934) -> (w1933:T44)
            n882 = call <vilib>:"Add State(s) to Queue__jki_lib_state_machine.vi"("State(s) in (\"\")"=w1944) -> ("States Out"=w1943:string)  [unwired: 14 in]
          }
          frame "Command: setAO_Frequency" {
            # "#done"
            # "Convert Data from Message\nto appropriate data type"
            # "Triggers User Event to update front panel\nand put data onto class wire"
            n883 = Unbundle By Name(w1954) -> ("Message"=w1952:T43, "Lockin"=w1958:refnum<class "Instrument.Lockin.lvclass">, "Message.Command"=w1948:string, "Message.Data"=w1949:variant)
            n884 = call "Variant to LV Data.vim"("type"=T24 {"AO Channel"=5, "Frequency (Hz)"=0.0} ("setAO_f"), "error in (no error)"=w1947, "JSON Data in"=w1949, "Command"=w1948) -> ("error out"=w1946:errorcluster, "Data out"=w1945:T24)  [unwired: 4 in, 2 out]
            n885 = Unbundle By Name(w1945) -> ("AO Channel"=w1962:i32, "Frequency (Hz)"=w1961:dbl)
            n886 = call "Update AO Parameter.vi"("Parameter"=T22."Frequency", "error in"=w1946, "Value"=w1961, "Channel"=w1962, "Instrument.Lockin"=w1958) -> ("error out"=w1959:errorcluster, 2:w1957, "Instrument.Lockin out"=w1956:refnum<class "Instrument.Lockin.lvclass">)  [unwired: 4 in]
            n887 = property on="AO Channels" class="Arr (strict)"(error in=w1959, "Val(Sgnl)"=w1957) -> (error out=w1951:errorcluster)  [unwired: 1 in, 1 out]
            n888 = To Variant(anything=w1957) -> (Variant=w1963:variant)
            n889 = Bundle By Name(cluster=w1952, "Data"=w1963) -> (w1953:T43)
            n890 = Bundle By Name(cluster=w1954, "HandledMessage"=w1953, "Lockin"=w1956) -> (w1955:T44)
            n891 = call <vilib>:"Add State(s) to Queue__jki_lib_state_machine.vi"("State(s) in (\"\")"=w1966) -> ("States Out"=w1965:string)  [unwired: 14 in]
          }
          frame "Command: setAO_Phase" {
            # "#done"
            # "Convert Data from Message\nto appropriate data type"
            # "Triggers User Event to update front panel\nand put data onto class wire"
            n892 = Unbundle By Name(w1976) -> ("Message"=w1974:T43, "Lockin"=w1980:refnum<class "Instrument.Lockin.lvclass">, "Message.Command"=w1970:string, "Message.Data"=w1971:variant)
            n893 = call "Variant to LV Data.vim"("type"=T25 {"AO Channel"=5, "Phase (°)"=0.0} ("setAO_phi"), "error in (no error)"=w1969, "JSON Data in"=w1971, "Command"=w1970) -> ("error out"=w1968:errorcluster, "Data out"=w1967:T25)  [unwired: 4 in, 2 out]
            n894 = Unbundle By Name(w1967) -> ("AO Channel"=w1984:i32, "Phase (°)"=w1983:dbl)
            n895 = call "Update AO Parameter.vi"("Parameter"=T22."Phase", "error in"=w1968, "Value"=w1983, "Channel"=w1984, "Instrument.Lockin"=w1980) -> ("error out"=w1981:errorcluster, 2:w1979, "Instrument.Lockin out"=w1978:refnum<class "Instrument.Lockin.lvclass">)  [unwired: 4 in]
            n896 = property on="AO Channels" class="Arr (strict)"(error in=w1981, "Val(Sgnl)"=w1979) -> (error out=w1973:errorcluster)  [unwired: 1 in, 1 out]
            n897 = To Variant(anything=w1979) -> (Variant=w1985:variant)
            n898 = Bundle By Name(cluster=w1974, "Data"=w1985) -> (w1975:T43)
            n899 = Bundle By Name(cluster=w1976, "HandledMessage"=w1975, "Lockin"=w1978) -> (w1977:T44)
            n900 = call <vilib>:"Add State(s) to Queue__jki_lib_state_machine.vi"("State(s) in (\"\")"=w1988) -> ("States Out"=w1987:string)  [unwired: 14 in]
          }
          frame "Command: setAO_Function" {
            # "#done"
            # "Convert Data from Message\nto appropriate data type"
            # "Triggers User Event to update front panel\nand put data onto class wire"
            n901 = Unbundle By Name(w1998) -> ("Message"=w1996:T43, "Lockin"=w2002:refnum<class "Instrument.Lockin.lvclass">, "Message.Command"=w1993:string, "Message.Data"=w1992:variant)
            n902 = call "Variant to LV Data.vim"("type"=T26 {"AO Channel"=5, "Function"=enum."Sine"} ("setAO_function"), "error in (no error)"=w1991, "JSON Data in"=w1992, "Command"=w1993) -> ("error out"=w1990:errorcluster, "Data out"=w1989:T26)  [unwired: 4 in, 2 out]
            n903 = Unbundle By Name(w1989) -> ("AO Channel"=w2006:i32, "Function"=w2005:T27)
            n904 = call "Update AO Parameter.vi"("Parameter"=T22."Function", "error in"=w1990, "Value"=w2005, "Channel"=w2006, "Instrument.Lockin"=w2002) -> ("error out"=w2003:errorcluster, 2:w2001, "Instrument.Lockin out"=w2000:refnum<class "Instrument.Lockin.lvclass">)  [unwired: 4 in]
            n905 = property on="AO Channels" class="Arr (strict)"(error in=w2003, "Val(Sgnl)"=w2001) -> (error out=w1995:errorcluster)  [unwired: 1 in, 1 out]
            n906 = To Variant(anything=w2001) -> (Variant=w2007:variant)
            n907 = Bundle By Name(cluster=w1996, "Data"=w2007) -> (w1997:T43)
            n908 = Bundle By Name(cluster=w1998, "HandledMessage"=w1997, "Lockin"=w2000) -> (w1999:T44)
            n909 = call <vilib>:"Add State(s) to Queue__jki_lib_state_machine.vi"("State(s) in (\"\")"=w2010) -> ("States Out"=w2009:string)  [unwired: 14 in]
          }
          frame "Command: setREF_Frequency" {
            # "#done"
            # "Convert Data from Message\nto appropriate data type"
            # "Triggers User Event to update front panel\nand put data onto class wire"
            n910 = Unbundle By Name(w2021) -> ("Message"=w2019:T43, "Lockin"=w2025:refnum<class "Instrument.Lockin.lvclass">, "Message.Command"=w2015:string, "Message.Data"=w2014:variant)
            n911 = call "Variant to LV Data.vim"("type"=T29 {"REF Channel"=0, "Frequency (Hz)"=0.0} ("setREF_f"), "error in (no error)"=w2013, "JSON Data in"=w2014, "Command"=w2015) -> ("error out"=w2012:errorcluster, "Data out"=w2011:T29)  [unwired: 4 in, 2 out]
            n912 = Unbundle By Name(w2011) -> ("REF Channel"=w2028:i32, "Frequency (Hz)"=w2027:dbl)
            n913 = call "Update REF Parameter.vi"("Parameter"=REF_Parameter--Enum."Frequency", "error in"=w2012, "Value"=w2027, "Channel"=w2028, "Instrument.Lockin"=w2025) -> ("error out"=w2026:errorcluster, 2:w2024, "Instrument.Lockin out"=w2023:refnum<class "Instrument.Lockin.lvclass">)  [unwired: 4 in]
            n914 = property on="REF Channels" class="Arr (strict)"(error in=w2026, "Val(Sgnl)"=w2024) -> (error out=w2018:errorcluster)  [unwired: 1 in, 1 out]
            n915 = To Variant(anything=w2024) -> (Variant=w2029:variant)
            n916 = Bundle By Name(cluster=w2019, "Data"=w2029) -> (w2020:T43)
            n917 = Bundle By Name(cluster=w2021, "HandledMessage"=w2020, "Lockin"=w2023) -> (w2022:T44)
            n918 = call <vilib>:"Add State(s) to Queue__jki_lib_state_machine.vi"("State(s) in (\"\")"=w2032) -> ("States Out"=w2031:string)  [unwired: 14 in]
          }
          frame "Command: setREF_Phase" {
            # "#done"
            # "Convert Data from Message\nto appropriate data type"
            # "Triggers User Event to update front panel\nand put data onto class wire"
            n919 = Unbundle By Name(w2043) -> ("Message"=w2041:T43, "Lockin"=w2047:refnum<class "Instrument.Lockin.lvclass">, "Message.Command"=w2036:string, "Message.Data"=w2037:variant)
            n920 = call "Variant to LV Data.vim"("type"=T30 {"REF Channel"=0, "Phase (°)"=0.0} ("setREF_phi"), "error in (no error)"=w2035, "JSON Data in"=w2037, "Command"=w2036) -> ("error out"=w2034:errorcluster, "Data out"=w2033:T30)  [unwired: 4 in, 2 out]
            n921 = Unbundle By Name(w2033) -> ("REF Channel"=w2050:i32, "Phase (°)"=w2049:dbl)
            n922 = call "Update REF Parameter.vi"("Parameter"=REF_Parameter--Enum."Phase", "error in"=w2034, "Value"=w2049, "Channel"=w2050, "Instrument.Lockin"=w2047) -> ("error out"=w2048:errorcluster, 2:w2046, "Instrument.Lockin out"=w2045:refnum<class "Instrument.Lockin.lvclass">)  [unwired: 4 in]
            n923 = property on="REF Channels" class="Arr (strict)"(error in=w2048, "Val(Sgnl)"=w2046) -> (error out=w2040:errorcluster)  [unwired: 1 in, 1 out]
            n924 = To Variant(anything=w2046) -> (Variant=w2051:variant)
            n925 = Bundle By Name(cluster=w2041, "Data"=w2051) -> (w2042:T43)
            n926 = Bundle By Name(cluster=w2043, "HandledMessage"=w2042, "Lockin"=w2045) -> (w2044:T44)
            n927 = call <vilib>:"Add State(s) to Queue__jki_lib_state_machine.vi"("State(s) in (\"\")"=w2054) -> ("States Out"=w2053:string)  [unwired: 14 in]
          }
          frame "Command: setREF_TC" {
            # "#done"
            # "Convert Data from Message\nto appropriate data type"
            # "Triggers User Event to update front panel\nand put data onto class wire"
            n928 = Unbundle By Name(w2065) -> ("Message"=w2063:T43, "Lockin"=w2069:refnum<class "Instrument.Lockin.lvclass">, "Message.Command"=w2058:string, "Message.Data"=w2059:variant)
            n929 = call "Variant to LV Data.vim"("type"=T31 {"REF Channel"=0, "TC (s)"=1e-05} ("setREF_phi"), "error in (no error)"=w2057, "JSON Data in"=w2059, "Command"=w2058) -> ("error out"=w2056:errorcluster, "Data out"=w2055:T31)  [unwired: 4 in, 2 out]
            n930 = Unbundle By Name(w2055) -> ("REF Channel"=w2072:i32, "TC (s)"=w2071:dbl)
            n931 = call "Update REF Parameter.vi"("Parameter"=REF_Parameter--Enum."Time Constant", "error in"=w2056, "Value"=w2071, "Channel"=w2072, "Instrument.Lockin"=w2069) -> ("error out"=w2070:errorcluster, 2:w2068, "Instrument.Lockin out"=w2067:refnum<class "Instrument.Lockin.lvclass">)  [unwired: 4 in]
            n932 = property on="REF Channels" class="Arr (strict)"(error in=w2070, "Val(Sgnl)"=w2068) -> (error out=w2062:errorcluster)  [unwired: 1 in, 1 out]
            n933 = To Variant(anything=w2068) -> (Variant=w2073:variant)
            n934 = Bundle By Name(cluster=w2063, "Data"=w2073) -> (w2064:T43)
            n935 = Bundle By Name(cluster=w2065, "HandledMessage"=w2064, "Lockin"=w2067) -> (w2066:T44)
            n936 = call <vilib>:"Add State(s) to Queue__jki_lib_state_machine.vi"("State(s) in (\"\")"=w2076) -> ("States Out"=w2075:string)  [unwired: 14 in]
          }
          frame "Command: setREF_RollOff" {
            # "#done"
            # "Convert Data from Message\nto appropriate data type"
            # "Triggers User Event to update front panel\nand put data onto class wire"
            n937 = Unbundle By Name(w2087) -> ("Message"=w2085:T43, "Lockin"=w2091:refnum<class "Instrument.Lockin.lvclass">, "Message.Command"=w2077:string, "Message.Data"=w2078:variant)
            n938 = call "Variant to LV Data.vim"("type"=T32 {"REF Channel"=0, "Roll-Off"=1} ("setREF_Roll-Off"), "error in (no error)"=w2079, "JSON Data in"=w2078, "Command"=w2077) -> ("error out"=w2080:errorcluster, "Data out"=w2081:T32)  [unwired: 4 in, 2 out]
            n939 = Unbundle By Name(w2081) -> ("REF Channel"=w2094:i32, "Roll-Off"=w2093:i32)
            n940 = call "Update REF Parameter.vi"("Parameter"=REF_Parameter--Enum."RollOff", "error in"=w2080, "Value"=w2093, "Channel"=w2094, "Instrument.Lockin"=w2091) -> ("error out"=w2092:errorcluster, 2:w2090, "Instrument.Lockin out"=w2089:refnum<class "Instrument.Lockin.lvclass">)  [unwired: 4 in]
            n941 = property on="REF Channels" class="Arr (strict)"(error in=w2092, "Val(Sgnl)"=w2090) -> (error out=w2084:errorcluster)  [unwired: 1 in, 1 out]
            n942 = To Variant(anything=w2090) -> (Variant=w2095:variant)
            n943 = Bundle By Name(cluster=w2085, "Data"=w2095) -> (w2086:T43)
            n944 = Bundle By Name(cluster=w2087, "HandledMessage"=w2086, "Lockin"=w2089) -> (w2088:T44)
            n945 = call <vilib>:"Add State(s) to Queue__jki_lib_state_machine.vi"("State(s) in (\"\")"=w2098) -> ("States Out"=w2097:string)  [unwired: 14 in]
          }
          frame "Command: setOffset" {
            # "#done"
            # "Convert Data from Message\nto appropriate data type"
            # "Triggers User Event to update front panel\nand put data onto class wire"
            n946 = Unbundle By Name(w2105) -> ("Message"=w2104:T43, "Message.Command"=w2099:string, "Message.Data"=w2100:variant)
            n947 = call "Variant to LV Data.vim"("type"=Offset_Mode--Enum."Remove" ("Offset Mode"), "error in (no error)"=w2101, "JSON Data in"=w2100, "Command"=w2099) -> ("error out"=w2102:errorcluster, "Data out"=w2103:T33)  [unwired: 4 in, 2 out]
            n948 = case shown="\"Remove\"" w2103 {
              tunnel: ["DONE: Measure Offset" ("State(s) in Front (\"\")") "DONE: Remove Offset" ("State(s) in Front (\"\")")] -> w2108
              frame "Measure", Default {
              }
              frame "Remove" {
              }
            }
            n949 = Bundle By Name(cluster=w2104, "Data"=w2103) -> (w2109:T43)
            n950 = Bundle By Name(cluster=w2105, "HandledMessage"=w2109) -> (w2106:T44)
            n951 = call <vilib>:"Add State(s) to Queue__jki_lib_state_machine.vi"("State(s) in Front (\"\")"=w2108, "State(s) in (\"\")"=w2112) -> ("States Out"=w2111:string)  [unwired: 13 in]
          }
          frame "4461: SAMPLING SETUP" {
            # "#DONE....mostly"
            n952 = Unbundle By Name(w2118) -> ("Lockin"=w2121:refnum<class "Instrument.Lockin.lvclass">)
            n953 = call "DAQ.Sampling.Configure.vi"("Instrument.DAQ"=w2121) -> ("Instrument.DAQ out"=w2115:refnum<class "Instrument.DAQ.lvclass">)  [unwired: 9 in, 1 out]
            n954 = call <userlib>:"Write sampling.vi"("error in (no error)"=w2120, "sampling"=w2115, "Instrument.Lockin in"=w2121) -> ("error out"=w2119:errorcluster, "Instrument.Lockin out"=w2117:refnum<class "Instrument.Lockin.lvclass">)  [unwired: 7 in]
            n955 = Bundle By Name(cluster=w2118, "Lockin"=w2117) -> (w2116:T44)
            n956 = local write "Sampling"(w2115) -> ()
            n957 = call <vilib>:"Add State(s) to Queue__jki_lib_state_machine.vi"("State(s) in (\"\")"=w2124) -> ("States Out"=w2123:string)  [unwired: 14 in]
          }
          frame "done: SAVE" {
            (unwired) i32[] [1, 1] ("X,Y Log")
            (unwired) string[] ["FFT0", "FFT1", "FFT2", "FFT3", "FFT4", "FFT5", "FFT6", "FFT7"] ("wavenames (.Vx, etc)")
            (unwired) string[] ["ch0", "ch1", "ch2", "ch3", "ch4", "ch5", "ch6", "ch7"] ("wavenames (.Vx, etc)")
            # "#done\n(not used)"
            # "Wait for Trigger signal from other VI"
            n958 = local read "PS WFGraph"() -> (w2138:cluster{"f0":dbl, "df":dbl, "magnitude":dbl[]}[])
            n959 = Unbundle By Name(w2126) -> ("Lockin"=w2128:refnum<class "Instrument.Lockin.lvclass">)
            n960 = Unbundle By Name(w2128) -> ("AI"=w2129:waveform(dbl)[])
            n961 = for {
              tunnel: w2138 -> [w2155] mode=indexing
              tunnel: [w2150] -> _ mode=indexing
              n962 = Unbundle By Name(w2155) -> ("df"=w2157:dbl, "magnitude"=w2156:dbl[])  [unwired: 1 out]
              n963 = Bundle By Name("dt"=w2157, "Y"=w2156) -> (w2154:waveform(dbl))  [unwired: 1 in]
              n964 = call-poly <vilib>:"Waveform to XY Pairs.vi"("waveform in"=w2154) -> ("XY pairs"=w2153:cluster{"x":timestamp, "y":dbl}[])  [unwired: 8 in, 2 out]
              n965 = for {
                tunnel: w2153 -> [w2161] mode=indexing
                tunnel: [w2159] -> w2151 mode=indexing
                tunnel: [w2158] -> w2152 mode=indexing
                n966 = Unbundle(w2161) -> ("x"=w2160:timestamp, "y"=w2159:dbl)
                n967 = To Double Precision Float(number=w2160) -> (double precision float=w2158:dbl)
              }
              n968 = Bundle(w2152, w2151) -> (w2150:cluster{dbl[], dbl[]})  [unwired: 1 in]
            }
            n969 = Get Date/Time In Seconds() -> (seconds since 1Jan1904=w2137:timestamp)
            n970 = for {
              tunnel: [w2142] -> _ mode=indexing
              tunnel: w2129 -> [w2141] mode=indexing
              n971 = call-poly <vilib>:"Waveform to XY Pairs.vi"("waveform in"=w2141) -> ("XY pairs"=w2145:cluster{"x":timestamp, "y":dbl}[])  [unwired: 8 in, 2 out]
              n972 = for {
                tunnel: w2145 -> [w2149] mode=indexing
                tunnel: [w2147] -> w2143 mode=indexing
                tunnel: [w2146] -> w2144 mode=indexing
                n973 = Unbundle(w2149) -> ("x"=w2148:timestamp, "y"=w2147:dbl)
                n974 = To Double Precision Float(number=w2148) -> (double precision float=w2146:dbl)
              }
              n975 = Bundle(w2144, w2143) -> (w2142:cluster{dbl[], dbl[]})  [unwired: 1 in]
            }
            n976 = Format Date/Time String(time format string (%c)="%Y-%m-%d", seconds (now)=w2137) -> (date/time string=w2136:string)  [unwired: 1 in]
            n977 = Build Path(base path="Path", name or relative path=w2136) -> (appended path=w2135:path)
            n978 = Build Path(base path=w2135, name or relative path="signal" ("filename")) -> ()  [unwired: 1 out]
            n979 = Build Path(base path=w2135, name or relative path="FFT" ("filename")) -> ()  [unwired: 1 out]
            n980 = local write "Save"(FALSE ("SAVE DATA")) -> ()
            n981 = call <vilib>:"Add State(s) to Queue__jki_lib_state_machine.vi"("State(s) in (\"\")"=w2127) -> ("States Out"=w2140:string)  [unwired: 14 in]
          }
          frame "Notes: Controls" {
            n982 = call <vilib>:"Add State(s) to Queue__jki_lib_state_machine.vi"("State(s) in (\"\")"=w2166) -> ("States Out"=w2165:string)  [unwired: 14 in]
          }
          frame "Notes: Notes" {
            # "calculate RMS, Noise bandwidth, etc"
            # "Go to \"4461: SETUP\" if Reset, remote mode,\nor IV/continuous mode buttons are pushed"
            # "Multichannel Lockin v2016/06/02 SW TIMED SINGLE POINT\nREF:\nhttp://www.ni.com/white-paper/3215/en/ Example 9"
            # "TO DO:\n- intelligent decimate to dt setpoint\ncalculate RMS, Noise bandwidth, etc"
            n983 = disable-structure shown="Enabled" {
              frame Disabled {
                n984 = call <vilib>:"Open Config Data.vi"() -> ()  [unwired: 9 in, 3 out]
              }
              frame Enabled {
                # "JKI State Machine™\nhttp://jkisoft.com/state-machine/\nCopyright (C) 2005-2008, JKI <info@jkisoft.com>\nALL RIGHTS RESERVED"
                # "State Syntax:\nStateCategory: State >> Argument\nLine Terminator: Line feed\nExample:\nUI: Help >> About\n\nWhere \"UI\" is the state category\nWhere \"Help\" is the state\nWhere \"About\" is the argument\nOther Examples:\nApp Data: Initialize\nUI: Initialize\nHelp >> About\n\nCommenting:\nTo add a comment use \"//\" or \"#\" and all text to the right will be ignored\n\nCommenting Example:\nUI: Initialize // This initializes the UI\n# This whole line is a comment\n// Another comment line"
              }
            }
            n985 = call <vilib>:"Add State(s) to Queue__jki_lib_state_machine.vi"("State(s) in (\"\")"=w2171) -> ("States Out"=w2170:string)  [unwired: 14 in]
          }
          frame "TODO: Set AO Zero Amplitude" {
            # "#done"
            n986 = Unbundle By Name(w2178) -> ("Lockin.DAQ"=w2185:refnum<class "Instrument.DAQ.lvclass">, "Lockin"=w2177:refnum<class "Instrument.Lockin.lvclass">)
            n987 = Unbundle By Name(w2177) -> ("AO"=w2172:T81, "#s"=w2183:i32, "Fs"=w2182:dbl)
            n988 = Divide(x=w2183, y=w2182) -> (x/y=w2175:dbl)
            n989 = Multiply(x=1000.0 ("y"), y=w2175) -> (x*y=w2181:dbl)
            n990 = for {
              tunnel: w2172 -> [w2191] mode=indexing
              tunnel: [w2189] -> w2174 mode=indexing
              n991 = Bundle By Name(cluster=w2191, "Amplitude"=0.0 ("element")) -> (w2189:T82)
            }
            n992 = To Unsigned Long Integer(number=w2181) -> (unsigned 32bit integer=w2180:u32)
            n993 = call <userlib>:"Lockin.DAQ.setAO.vi"("error in (no error)"=w2184, "AO Channels"=w2174, "Lockin.DAQ"=w2185) -> ("error out"=w2173:errorcluster)  [unwired: 7 in, 1 out]
            n994 = call <userlib>:"Wait (ms)__ogtk.vi"("error in (no error)"=w2173, "milliseconds to wait"=w2180) -> ("error out"=w2179:errorcluster)  [unwired: 8 in, 1 out]
            n995 = call <vilib>:"Add State(s) to Queue__jki_lib_state_machine.vi"("State(s) in (\"\")"=w2188) -> ("States Out"=w2187:string)  [unwired: 14 in]
          }
          frame "TODO: Update Plot Names" {
            # "#done"
            # "#done"
            # "#done"
            n996 = Unbundle By Name(w2193) -> ("Lockin"=w2200:refnum<class "Instrument.Lockin.lvclass">)
            n997 = Equal?(x=w2202, y="Reset") -> ()  [unwired: 1 out]
            n998 = call "Get AO StringsAndValues.vi"("error in (no error)"=w2199, "Configuration.DAQ"=w2200) -> ("error out"=w2204:errorcluster, "AO Strings and Values"=w2195:cluster{string, i32}[])  [unwired: 8 in]
            n999 = call "Get AI StringsAndValues.vi"("error in (no error)"=w2199, "Configuration.DAQ"=w2200) -> ("error out"=w2205:errorcluster, "AI StringsAndValues"=w2206:cluster{string, i32}[])  [unwired: 8 in]
            n1000 = call "Get AI REF StringsAndValues.vi"("error in (no error)"=w2199, "Channels.REF"=w2200) -> ("error out"=w2197:errorcluster, "REF StringsAndValues"=w2192:cluster{string, i32}[])  [unwired: 8 in]
            n1001 = for {
              tunnel: w2195 -> [w2223] mode=indexing
              tunnel: w2204 -> [w2224]
              tunnel: [w2221] -> w2203
              i -> [w2225]
              n1002 = control-ref of="Sweep Results AO"() -> (w2222:refnum<vi>)
              n1003 = Unbundle(w2223) -> (w2226:string)  [unwired: 1 out]
              n1004 = call <userlib>:"Legend - WaveformGraph.vi"("error in (no error)"=w2224, "Plot.Plot Name"=w2226, "Active Plot"=w2225, "WFGraph in"=w2222) -> ("error out"=w2221:errorcluster)  [unwired: 4 in, 3 out]
            }
            n1005 = for {
              tunnel: w2206 -> [w2236] mode=indexing
              tunnel: w2205 -> [w2237]
              tunnel: [w2229] -> w2208
              i -> [w2238]
              n1006 = control-ref of="AI Graph"() -> (w2239:refnum<vi>)
              n1007 = Unbundle(w2236) -> (w2240:string)  [unwired: 1 out]
              n1008 = control-ref of="Sweep Results AI"() -> (w2232:refnum<vi>)
              n1009 = call <userlib>:"Legend - WaveformGraph.vi"("error in (no error)"=w2237, "Plot.Plot Name"=w2240, "Active Plot"=w2238, "WFGraph in"=w2239) -> ("error out"=w2235:errorcluster, "Plot.Plot Name"=w2234:string, "Active Plot"=w2233:i32)  [unwired: 4 in, 1 out]
              n1010 = call <userlib>:"Legend - WaveformGraph.vi"("error in (no error)"=w2235, "Plot.Plot Name"=w2234, "Active Plot"=w2233, "WFGraph in"=w2232) -> ("error out"=w2231:errorcluster, "Plot.Plot Name"=w2228:string, "Active Plot"=w2227:i32)  [unwired: 4 in, 1 out]
              n1011 = control-ref of="PS WFGraph"() -> (w2230:refnum<vi>)
              n1012 = call <userlib>:"Legend - WDTWaveformGraph.vi"("error in (no error)"=w2231, "Plot.Plot Name"=w2228, "Active Plot"=w2227, "WFGraph (WDT) in"=w2230) -> ("error out"=w2229:errorcluster)  [unwired: 4 in, 3 out]
            }
            n1013 = local read "Y Axis (Output)"() -> (w2194:enum16{"Analog Output", "Reference"})
            n1014 = case shown="\"Reference\"" w2194 {
              tunnel: [w2212 w2213] -> w2198
              tunnel: w2192 -> [_ w2214]
              tunnel: w2195 -> [w2212 _]
              frame "Analog Output", Default {
              }
              frame "Reference" {
                n1015 = Interleave 1D Arrays(w2214, w2214) -> (w2213:cluster{string, i32}[])
              }
            }
            n1016 = for {
              tunnel: w2198 -> [w2219] mode=indexing
              tunnel: w2197 -> [w2217]
              tunnel: [w2216] -> w2196
              i -> [w2218]
              n1017 = Unbundle(w2219) -> (w2215:string)  [unwired: 1 out]
              n1018 = control-ref of="AO Graph"() -> (w2220:refnum<vi>)
              n1019 = call <userlib>:"Legend - WaveformGraph.vi"("error in (no error)"=w2217, "Plot.Plot Name"=w2215, "Active Plot"=w2218, "WFGraph in"=w2220) -> ("error out"=w2216:errorcluster)  [unwired: 4 in, 3 out]
            }
            n1020 = call <vilib>:"Add State(s) to Queue__jki_lib_state_machine.vi"("State(s) in (\"\")"=w2211) -> ("States Out"=w2210:string)  [unwired: 14 in]
            n1021 = Merge Errors(w2203, w2208, w2196) -> (w2207:errorcluster)
          }
          frame "TODO: Set Sampling" {
            w2242 = 100  # AI Buffer Size (S)
            # "#done mostly\n#todo decimate/sample mode?"
            # "Is there a more elegant way to do this?"
            n1022 = Unbundle By Name(w2243) -> ("Lockin.DAQ"=w2250:refnum<class "Instrument.DAQ.lvclass">, "Lockin"=w2246:refnum<class "Instrument.Lockin.lvclass">)
            n1023 = Unbundle By Name(w2246) -> ("Sampling"=w2244:T99)
            n1024 = case shown="\"10178\", Default" w2245 {
              tunnel: [w2254 w2255] -> w2247
              frame "10178", Default {
                w2254 = 10178 items=["Finite Samples"=10178, "Continuous Samples"=10123] ("Sample Mode")
              }
              frame "10123" {
                w2255 = 10123 items=["Finite Samples"=10178, "Continuous Samples"=10123] ("Sample Mode")
              }
            }
            n1025 = call <userlib>:"Lockin.DAQ.setSampling.vi"("Decimation"="decimating factor", "AI Buffer Size (S)"=w2242, "error in (no error)"=w2249, "Sample Mode"=w2247, "Sampling"=w2244, "Lockin.DAQ"=w2250) -> ("error out"=w2248:errorcluster)  [unwired: 4 in, 1 out]
            n1026 = call <vilib>:"Add State(s) to Queue__jki_lib_state_machine.vi"("State(s) in (\"\")"=w2253) -> ("States Out"=w2252:string)  [unwired: 14 in]
          }
          frame "---------- TODO ----------" {
            n1027 = call <vilib>:"Add State(s) to Queue__jki_lib_state_machine.vi"("State(s) in (\"\")"=w2260) -> ("States Out"=w2259:string)  [unwired: 14 in]
          }
          frame "4461: OUT" {
            n1028 = Unbundle By Name(w2262) -> ("Lockin"=w2265:refnum<class "Instrument.Lockin.lvclass">)
            n1029 = case shown="True" "Enable Output" {
              tunnel: [w2269 w2277] -> w2263
              tunnel: w2265 -> [_ w2281]
              tunnel: w2261 -> [w2269 w2273]
              frame False {
              }
              frame True {
                # "this will act as a self-call\nmeaning after the remote call comes\nin the data on the data bus will get updated\nby other means"
                n1030 = Unbundle By Name(w2281) -> ("AI.Gain"=w2282:T40, "Results (Dictionary)"=w2276:cluster{"key":string, "value":dbl}[])
                n1031 = call "Parse Results (all).vi"("error in (no error)"=w2273, "Results (Dictionary)"=w2276) -> ("error out"=w2274:errorcluster, "Results (Dictionary)"=w2275:cluster{"key":string, "value":dbl}[])  [unwired: 6 in, 2 out]
                n1032 = Index Array(array=w2282, index="Type") -> (element=w2280:T41)
                n1033 = call "Parse Results (single).vi"("Type"="Type", "error in (no error)"=w2274, "Reference Channel"="Reference Channel", "AI Channel"="AI Channel", "Results (Dictionary)"=w2275) -> ("error out"=w2278:errorcluster, "Data"=w2279:dbl)  [unwired: 3 in, 2 out]
                n1034 = Multiply(x=w2279, y=w2280) -> (x*y=w2283:dbl)
                "Output (V)" <- w2283
                n1035 = call "setAO_DC.vi"("error in (no error)"=w2278, "DC (V)"=w2283, "AO Channel"="Output Channel", "Instrument.Lockin in"=w2281) -> ("error out"=w2277:errorcluster)  [unwired: 6 in, 1 out]
              }
            }
            n1036 = call <vilib>:"Add State(s) to Queue__jki_lib_state_machine.vi"("State(s) in (\"\")"=w2267) -> ("States Out"=w2268:string)  [unwired: 14 in]
          }
          frame "4461: FFT" {
            n1037 = Unbundle By Name(w2303) -> ("Lockin"=w2302:refnum<class "Instrument.Lockin.lvclass">)
            n1038 = Unbundle By Name(w2302) -> ("AI"=w2292:waveform(dbl)[])
            n1039 = Bundle By Name(cluster=T34 {"averaging mode"=enum."No averaging", "weighting mode"=enum."Exponential", "number of averages"=10} ("averaging parameters"), "averaging mode"="averaging mode", "weighting mode"="weighting mode", "number of averages"="# averages") -> (w2295:T34)
            n1040 = call-poly <vilib>:"FFT Power Spectrum and PSD.vi"("export mode"="export mode", "averaging parameters"=w2295, "restart averaging (F)"="restart", "error in (no error)"=w2291, "dB On (F)"=TRUE, "window"="window", "time signals"=w2292) -> ("error out"=w2304:errorcluster, "averages completed"=→"averages":dbl, "averaging done"=→"done?":bool, "Power Spectrum / PSD"=w2288:cluster{"f0":dbl, "df":dbl, "magnitude":dbl[]}[])  [unwired: 1 in]
            "PS WFGraph" <- w2288
            n1041 = control-ref of="PS WFGraph"() -> (w2285:refnum<vi>)
            n1042 = for {
              tunnel: [w2311] -> w2290
              tunnel: w2291 -> [w2310]
              tunnel: w2288 -> [_] mode=indexing
              i -> [w2313]
              n1043 = property on="PS WFGraph" class="WFGraph (strict)"(error in=w2310, "Active Plot"=w2313) -> (error out=w2314:errorcluster, "Plot.Visible?"=w2312:bool)  [unwired: 1 in, 1 out]
              n1044 = property on="PS Chart" class="WFChart (strict)"(error in=w2314, "Active Plot"=w2313, "Plot.Visible?"=w2312) -> (error out=w2311:errorcluster)  [unwired: 1 in, 1 out]
            }
            n1045 = call "PS Chart.vi"("error in (no error)"=w2304, "Power Spectrum / PSD"=w2288, "WFGraph (WDT) in"=w2285) -> ("error out"=w2287:errorcluster, "Chart"=→"PS Chart":dbl[][])  [unwired: 7 in]
            n1046 = Merge Errors(w2287, w2290) -> (w2286:errorcluster)
            n1047 = call <vilib>:"Add State(s) to Queue__jki_lib_state_machine.vi"("State(s) in (\"\")"=w2305) -> ("States Out"=w2309:string)  [unwired: 14 in]
          }
          frame "AUX: Set AUX" {
            n1048 = call <userlib>:"Voltage Update.vi"("error in (no error)"=w2316, "Amplifier Gain"="Amplifier Gain", "Voltage Output"="Voltage Output (V)", "Physical Channel"="Aux Channel") -> ("error out"=w2315:errorcluster, "Amplified output"=→"Amplified Output (V)":dbl, "DAQ output"=→"DAQ Output (V)":dbl)  [unwired: 5 in]
            n1049 = Unbundle By Name(w2318) -> ("Lockin"=w2321:refnum<class "Instrument.Lockin.lvclass">)
            n1050 = Bundle By Name(cluster=w2321, "Aux Channel"="Aux Channel") -> (w2320:refnum<class "Instrument.Lockin.lvclass">)
            n1051 = Bundle By Name(cluster=w2318, "Lockin"=w2320) -> (w2322:T44)
            n1052 = call <vilib>:"Add State(s) to Queue__jki_lib_state_machine.vi"("State(s) in Front (\"\")"="DONE: Write CONFIG" ("State(s) in Front (\"\")"), "State(s) in (\"\")"=w2329) -> ("States Out"=w2328:string)  [unwired: 13 in]
          }
          frame "---------Command----------" {
            n1053 = call <vilib>:"Add State(s) to Queue__jki_lib_state_machine.vi"("State(s) in (\"\")"=w2334) -> ("States Out"=w2333:string)  [unwired: 14 in]
          }
          frame "Command: Reset" {
            # "#todo\nfollow event"
            # "#done"
            # "call Macro: RESET remote\nwhich does not restart the remote server"
            # "Convert Data from Message\nto appropriate data type"
            n1054 = Unbundle By Name(w2340) -> ("Message"=w2343:T43, "Message.Command"=w2339:string, "Message.Data"=w2338:variant)
            n1055 = call "Variant to LV Data.vim"("type"=TRUE, "error in (no error)"=w2337, "JSON Data in"=w2338, "Command"=w2339) -> ("error out"=w2336:errorcluster, "Data out"=w2335:bool)  [unwired: 4 in, 2 out]
            n1056 = To Variant(anything=w2335) -> (Variant=w2345:variant)
            n1057 = property on="Reset" class="Bool (strict)"(error in=w2336, "Val(Sgnl)"=w2335) -> (error out=w2346:errorcluster)  [unwired: 1 in, 1 out]
            n1058 = Bundle By Name(cluster=w2343, "Data"=w2345) -> (w2342:T43)
            n1059 = Bundle By Name(cluster=w2340, "HandledMessage"=w2342) -> (w2344:T44)
            n1060 = call <vilib>:"Add State(s) to Queue__jki_lib_state_machine.vi"("State(s) in Front (\"\")"="", "State(s) in (\"\")"=w2350) -> ("States Out"=w2349:string)  [unwired: 13 in]
          }
          frame "Command: Trigger" {
            # "#done"
            # "Convert Data from Message\nto appropriate data type"
            # "Triggers User Event to update front panel\nand put data onto class wire"
            n1061 = Unbundle By Name(w2361) -> ("Message"=w2359:T43, "Message.Command"=w2356:string, "Message.Data"=w2354:variant)
            n1062 = call "Variant to LV Data.vim"("type"=TRUE, "error in (no error)"=w2353, "JSON Data in"=w2354, "Command"=w2356) -> ("error out"=w2351:errorcluster, "Data out"=w2352:bool)  [unwired: 4 in, 2 out]
            n1063 = To Variant(anything=w2352) -> (Variant=w2360:variant)
            n1064 = property on="Trigger" class="Bool (strict)"(error in=w2351, "Val(Sgnl)"=w2352) -> (error out=w2362:errorcluster)  [unwired: 1 in, 1 out]
            n1065 = Bundle By Name(cluster=w2359, "Data"=w2360) -> (w2358:T43)
            n1066 = Bundle By Name(cluster=w2361, "HandledMessage"=w2358) -> (w2357:T44)
            n1067 = call <vilib>:"Add State(s) to Queue__jki_lib_state_machine.vi"("State(s) in (\"\")"=w2365) -> ("States Out"=w2364:string)  [unwired: 14 in]
          }
          frame "Command: setAO" {
            # "#todo\nfollow event"
            # "Convert Data from Message\nto appropriate data type"
            # "Triggers User Event to update front panel\nand put data onto class wire"
            n1068 = Unbundle By Name(w2377) -> ("Lockin"=w2371:refnum<class "Instrument.Lockin.lvclass">, "Message"=w2374:T43, "Message.Command"=w2368:string, "Message.Data"=w2367:variant)
            n1069 = Unbundle By Name(w2371) -> ("AO Channels"=w2372)
            n1070 = call "Variant to LV Data.vim"("type"=w2372, "error in (no error)"=w2366, "JSON Data in"=w2367, "Command"=w2368) -> ("error out"=w2370:errorcluster, "Data out"=w2369:variant)  [unwired: 4 in, 2 out]
            n1071 = To Variant(anything=w2369) -> (Variant=w2378:variant)
            n1072 = property on="AO Channels" class="Arr (strict)"(error in=w2370, "Val(Sgnl)"=w2369) -> (error out=w2375:errorcluster)  [unwired: 1 in, 1 out]
            n1073 = Bundle By Name(cluster=w2374, "Data"=w2378) -> (w2376:T43)
            n1074 = Bundle By Name(cluster=w2377, "HandledMessage"=w2376) -> (w2373:T44)
            n1075 = call <vilib>:"Add State(s) to Queue__jki_lib_state_machine.vi"("State(s) in (\"\")"=w2381) -> ("States Out"=w2380:string)  [unwired: 14 in]
          }
          frame "Command: setREF" {
            # "#todo\nfollow event"
            # "#done"
            # "Convert Data from Message\nto appropriate data type"
            # "Triggers User Event to update front panel\nand put data onto class wire"
            n1076 = Unbundle By Name(w2388) -> ("Lockin"=w2394:refnum<class "Instrument.Lockin.lvclass">, "Message"=w2390:T43, "Message.Command"=w2382:string, "Message.Data"=w2384:variant)
            n1077 = Unbundle By Name(w2394) -> ("REF Channels"=w2383)
            n1078 = call "Variant to LV Data.vim"("type"=w2383, "error in (no error)"=w2387, "JSON Data in"=w2384, "Command"=w2382) -> ("error out"=w2386:errorcluster, "Data out"=w2385:variant)  [unwired: 4 in, 2 out]
            n1079 = property on="REF Channels" class="Arr (strict)"(error in=w2386, "Val(Sgnl)"=w2385) -> (error out=w2393:errorcluster)  [unwired: 1 in, 1 out]
            n1080 = To Variant(anything=w2385) -> (Variant=w2392:variant)
            n1081 = Bundle By Name(cluster=w2390, "Data"=w2392) -> (w2389:T43)
            n1082 = Bundle By Name(cluster=w2388, "HandledMessage"=w2389) -> (w2391:T44)
            n1083 = call <vilib>:"Add State(s) to Queue__jki_lib_state_machine.vi"("State(s) in (\"\")"=w2397) -> ("States Out"=w2396:string)  [unwired: 14 in]
          }
          frame "Command: setAUX" {
            # "Convert Data from Message\nto appropriate data type"
            # "Triggers User Event to update front panel\nand put data onto class wire"
            n1084 = Unbundle By Name(w2406) -> ("Message"=w2407:T43, "Message.Command"=w2399:string, "Message.Data"=w2398:variant)
            n1085 = call "Variant to LV Data.vim"("type"=T35 {"AO Channel"=0, "AUX (V)"=0.0} ("setAUX"), "error in (no error)"=w2400, "JSON Data in"=w2398, "Command"=w2399) -> ("error out"=w2401:errorcluster, "Data out"=w2402:T35)  [unwired: 4 in, 2 out]
            n1086 = Unbundle By Name(w2402) -> ("AUX (V)"=w2405:dbl)  [unwired: 1 out]
            n1087 = local write "Voltage Output (V)"(w2405) -> ()
            n1088 = Bundle By Name(cluster=w2407, "Data"=w2405) -> (w2404:T43)
            n1089 = Bundle By Name(cluster=w2406, "HandledMessage"=w2404) -> (w2408:T44)
            n1090 = call <vilib>:"Add State(s) to Queue__jki_lib_state_machine.vi"("State(s) in Front (\"\")"="AUX: Set AUX" ("State(s) in Front (\"\")"), "State(s) in (\"\")"=w2412) -> ("States Out"=w2411:string)  [unwired: 13 in]
          }
          frame "Command: setSampling" {
            # "#todo\nfollow event"
            # "#done"
            # "Convert Data from Message\nto appropriate data type"
            # "Triggers User Event to update front panel\nand put data onto class wire"
            n1091 = Unbundle By Name(w2424) -> ("Lockin"=w2418:refnum<class "Instrument.Lockin.lvclass">, "Message"=w2419:T43, "Message.Command"=w2413:string, "Message.Data"=w2414:variant)
            n1092 = Unbundle By Name(w2418) -> ("sampling"=w2420)
            n1093 = call "Variant to LV Data.vim"("type"=w2420, "error in (no error)"=w2415, "JSON Data in"=w2414, "Command"=w2413) -> ("error out"=w2417:errorcluster, "Data out"=w2416:variant)  [unwired: 4 in, 2 out]
            n1094 = To Variant(anything=w2416) -> (Variant=w2425:variant)
            n1095 = Bundle By Name(cluster=w2419, "Data"=w2425) -> (w2422:T43)
            n1096 = property on="Sampling" class="Clust (strict)"(error in=w2417, "Val(Sgnl)"=w2416) -> (error out=w2421:errorcluster)  [unwired: 1 in, 1 out]
            n1097 = Bundle By Name(cluster=w2424, "HandledMessage"=w2422) -> (w2423:T44)
            n1098 = call <vilib>:"Add State(s) to Queue__jki_lib_state_machine.vi"("State(s) in (\"\")"=w2428) -> ("States Out"=w2427:string)  [unwired: 14 in]
          }
          frame "Command: setSweep" {
            w2435 = T103 {"Sweep Time (s)"=0.0, "Initial Wait (s)"=0.0, "Return to Start"=FALSE, "Channels"=[]}  # Configure Sweep
            # "#done"
            # "Convert Data from Message\nto appropriate data type"
            # "Triggers User Event to update front panel\nand put data onto class wire"
            n1099 = Unbundle By Name(w2434) -> ("Message"=w2437:T43, "Message.Command"=w2432:string, "Message.Data"=w2433:variant)
            n1100 = call "Variant to LV Data.vim"("type"=w2435, "error in (no error)"=w2431, "JSON Data in"=w2433, "Command"=w2432) -> ("error out"=w2430:errorcluster, "Data out"=w2429:T103)  [unwired: 4 in, 2 out]
            n1101 = To Variant(anything=w2429) -> (Variant=w2439:variant)
            n1102 = Unbundle By Name(w2429) -> ("Channels"=w2438:T8[], "Sweep Time (s)"=w2441:dbl, "Initial Wait (s)"=w2442:dbl, "Return to Start"=w2440:bool)
            n1103 = Bundle By Name(cluster=w2437, "Data"=w2439) -> (w2436:T43)
            n1104 = property on="Sweep Channels" class="Arr (strict)"("Val(Sgnl)"=w2438) -> ()  [unwired: 2 in, 2 out]
            n1105 = local write "Initial Wait (s)"(w2442) -> ()
            n1106 = Bundle By Name(cluster=w2434, "HandledMessage"=w2436) -> (w2443:T44)
            n1107 = property on="Sweep Time (s)" class="DigNum (strict)"("Val(Sgnl)"=w2441) -> ()  [unwired: 2 in, 2 out]
            n1108 = local write "Return to Start?"(w2440) -> ()
            n1109 = call <vilib>:"Add State(s) to Queue__jki_lib_state_machine.vi"("State(s) in (\"\")"=w2446) -> ("States Out"=w2445:string)  [unwired: 14 in]
          }
          frame "Command: startSweep" {
            # "#todo\nfollow event"
            # "#done"
            # "Convert Data from Message\nto appropriate data type"
            # "Triggers User Event to update front panel\nand put data onto class wire"
            n1110 = Unbundle By Name(w2452) -> ("Message"=w2455:T43, "Message.Command"=w2447:string, "Message.Data"=w2448:variant)
            n1111 = call "Variant to LV Data.vim"("type"=TRUE, "error in (no error)"=w2451, "JSON Data in"=w2448, "Command"=w2447) -> ("error out"=w2450:errorcluster, "Data out"=w2449:bool)  [unwired: 4 in, 2 out]
            n1112 = To Variant(anything=w2449) -> (Variant=w2456:variant)
            n1113 = Bundle By Name(cluster=w2455, "Data"=w2456) -> (w2454:T43)
            n1114 = Bundle By Name(cluster=w2452, "HandledMessage"=w2454) -> (w2453:T44)
            n1115 = property on="Start Sweep" class="Bool (strict)"(error in=w2450, "Val(Sgnl)"=w2449) -> (error out=w2458:errorcluster)  [unwired: 1 in, 1 out]
            n1116 = call <vilib>:"Add State(s) to Queue__jki_lib_state_machine.vi"("State(s) in (\"\")"=w2461) -> ("States Out"=w2460:string)  [unwired: 14 in]
          }
          frame "Command: stopSweep" {
            # "#todo\nfollow event"
            # "#done"
            # "Convert Data from Message\nto appropriate data type"
            # "Triggers User Event to update front panel\nand put data onto class wire"
            n1117 = Unbundle By Name(w2472) -> ("Message"=w2471:T43, "Message.Command"=w2462:string, "Message.Data"=w2463:variant)
            n1118 = call "Variant to LV Data.vim"("type"=TRUE, "error in (no error)"=w2466, "JSON Data in"=w2463, "Command"=w2462) -> ("error out"=w2465:errorcluster, "Data out"=w2464:bool)  [unwired: 4 in, 2 out]
            n1119 = To Variant(anything=w2464) -> (Variant=w2468:variant)
            n1120 = property on="Stop Sweep" class="Bool (strict)"(error in=w2465, "Val(Sgnl)"=w2464) -> (error out=w2473:errorcluster)  [unwired: 1 in, 1 out]
            n1121 = Bundle By Name(cluster=w2471, "Data"=w2468) -> (w2470:T43)
            n1122 = Bundle By Name(cluster=w2472, "HandledMessage"=w2470) -> (w2469:T44)
            n1123 = call <vilib>:"Add State(s) to Queue__jki_lib_state_machine.vi"("State(s) in (\"\")"=w2476) -> ("States Out"=w2475:string)  [unwired: 14 in]
          }
          frame "Command: setInputGain" {
            # "#todo\nfollow event"
            # "Convert Data from Message\nto appropriate data type"
            # "Triggers User Event to update front panel\nand put data onto class wire"
            n1124 = Unbundle By Name(w2490) -> ("Message"=w2484:T43, "Lockin"=w2488:refnum<class "Instrument.Lockin.lvclass">, "Message.Command"=w2480:string, "Message.Data"=w2481:variant)  [unwired: 1 out]
            n1125 = call "Get AI StringsAndValues.vi"("error in (no error)"=w2485, "Configuration.DAQ"=w2488) -> ("error out"=w2479:errorcluster, "AI StringsAndValues"=w2487:cluster{string, i32}[])  [unwired: 8 in]
            n1126 = Unbundle By Name(w2488) -> ("AI.Gain"=w2482:T40)
            n1127 = call "Variant to LV Data.vim"("type"=w2482, "error in (no error)"=w2479, "JSON Data in"=w2481, "Command"=w2480) -> ("error out"=w2478:errorcluster, "Data out"=w2477:T41[])  [unwired: 4 in, 2 out]
            n1128 = for {
              tunnel: [w2499] -> w2489 mode=indexing
              tunnel: w2477 -> [w2498] mode=indexing
              tunnel: w2487 -> [w2497] mode=indexing
              n1129 = Unbundle(w2497) -> (w2496:string)  [unwired: 1 out]
              n1130 = Bundle(w2496, "System Cluster"=w2498) -> (w2499:cluster{string, "System Cluster":T41})  [unwired: 1 in]
            }
            n1131 = To Variant(anything=w2477) -> (Variant=w2492:variant)
            n1132 = Bundle By Name(cluster=w2484, "Data"=w2492) -> (w2483:T43)
            n1133 = property on="Input Gain" class="Arr (strict)"(error in=w2478, "Val(Sgnl)"=w2489) -> (error out=w2486:errorcluster)  [unwired: 1 in, 1 out]
            n1134 = Bundle By Name(cluster=w2490, "HandledMessage"=w2483) -> (w2491:T44)
            n1135 = call <vilib>:"Add State(s) to Queue__jki_lib_state_machine.vi"("State(s) in (\"\")"=w2495) -> ("States Out"=w2494:string)  [unwired: 14 in]
          }
          frame "Command: setOutputGain" {
            # "#todo\nfollow event"
            # "Convert Data from Message\nto appropriate data type"
            # "Triggers User Event to update front panel\nand put data onto class wire"
            n1136 = Unbundle By Name(w2512) -> ("Message"=w2506:T43, "Lockin"=w2508:refnum<class "Instrument.Lockin.lvclass">, "Message.Command"=w2500:string, "Message.Data"=w2501:variant)
            n1137 = call "Get AO StringsAndValues.vi"("error in (no error)"=w2507, "Configuration.DAQ"=w2508) -> ("error out"=w2503:errorcluster, "AO Strings and Values"=w2509:cluster{string, i32}[])  [unwired: 8 in]
            n1138 = Unbundle By Name(w2508) -> ("AO.Gain"=w2513:T40)
            n1139 = call "Variant to LV Data.vim"("type"=w2513, "error in (no error)"=w2503, "JSON Data in"=w2501, "Command"=w2500) -> ("error out"=w2502:errorcluster, "Data out"=w2504:T41[])  [unwired: 4 in, 2 out]
            n1140 = for {
              tunnel: [w2522] -> w2511 mode=indexing
              tunnel: w2504 -> [w2521] mode=indexing
              tunnel: w2509 -> [w2520] mode=indexing
              n1141 = Unbundle(w2520) -> (w2519:string)  [unwired: 1 out]
              n1142 = Bundle(w2519, "System Cluster"=w2521) -> (w2522:cluster{string, "System Cluster":T41})  [unwired: 1 in]
            }
            n1143 = To Variant(anything=w2504) -> (Variant=w2515:variant)
            n1144 = Bundle By Name(cluster=w2506, "Data"=w2515) -> (w2505:T43)
            n1145 = property on="Output Gain" class="Arr (strict)"(error in=w2502, "Val(Sgnl)"=w2511) -> (error out=w2510:errorcluster)  [unwired: 1 in, 1 out]
            n1146 = Bundle By Name(cluster=w2512, "HandledMessage"=w2505) -> (w2514:T44)
            n1147 = call <vilib>:"Add State(s) to Queue__jki_lib_state_machine.vi"("State(s) in (\"\")"=w2518) -> ("States Out"=w2517:string)  [unwired: 14 in]
          }
          frame "Command: setIVmode" {
            # "#todo\nfollow event"
            # "Convert Data from Message\nto appropriate data type"
            # "Triggers User Event to update front panel\nand put data onto class wire"
            n1148 = Unbundle By Name(w2529) -> ("Message"=w2530:T43, "Message.Command"=w2526:string, "Message.Data"=w2527:variant)
            n1149 = call "Variant to LV Data.vim"("type"=TRUE, "error in (no error)"=w2525, "JSON Data in"=w2527, "Command"=w2526) -> ("error out"=w2523:errorcluster, "Data out"=w2524:bool)  [unwired: 4 in, 2 out]
            n1150 = To Variant(anything=w2524) -> (Variant=w2534:variant)
            n1151 = Bundle By Name(cluster=w2530, "Data"=w2534) -> (w2531:T43)
            n1152 = Bundle By Name(cluster=w2529, "HandledMessage"=w2531) -> (w2532:T44)
            n1153 = property on="Pause" class="Bool (strict)"(error in=w2523, "Val(Sgnl)"=w2524) -> (error out=w2533:errorcluster)  [unwired: 1 in, 1 out]
            n1154 = call <vilib>:"Add State(s) to Queue__jki_lib_state_machine.vi"("State(s) in (\"\")"=w2537) -> ("States Out"=w2536:string)  [unwired: 14 in]
          }
          frame "Command: setAutoSampling" {
            # "Convert Data from Message\nto appropriate data type"
            # "Triggers User Event to update front panel\nand put data onto class wire"
            n1155 = Unbundle By Name(w2545) -> ("Message"=w2543:T43, "Message.Command"=w2541:string, "Message.Data"=w2542:variant)
            n1156 = call "Variant to LV Data.vim"("type"=enum16{"Manual", "Auto Fs", "Max Fs"}."Auto Fs" ("Sampling Mode"), "error in (no error)"=w2540, "JSON Data in"=w2542, "Command"=w2541) -> ("error out"=w2539:errorcluster, "Data out"=w2538:enum16{"Manual", "Auto Fs", "Max Fs"})  [unwired: 4 in, 2 out]
            n1157 = To Variant(anything=w2538) -> (Variant=w2548:variant)
            n1158 = local write "Sampling Mode"(w2538) -> ()
            n1159 = Bundle By Name(cluster=w2543, "Data"=w2548) -> (w2544:T43)
            n1160 = Bundle By Name(cluster=w2545, "HandledMessage"=w2544) -> (w2547:T44)
            n1161 = call <vilib>:"Add State(s) to Queue__jki_lib_state_machine.vi"("State(s) in (\"\")"=w2551) -> ("States Out"=w2550:string)  [unwired: 14 in]
          }
          frame "Command: setDAQ" {
            # "#todo\nfollow event"
            # "Convert Data from Message\nto appropriate data type"
            # "Triggers User Event to update front panel\nand put data onto class wire"
            n1162 = Unbundle By Name(w2562) -> ("Message"=w2558:T43, "Message.Command"=w2555:string, "Message.Data"=w2556:variant)
            n1163 = call "Variant to LV Data.vim"("type"=T39 [] ("Value (Signaling)"), "error in (no error)"=w2554, "JSON Data in"=w2556, "Command"=w2555) -> ("error out"=w2552:errorcluster, "Data out"=w2553:T39)  [unwired: 4 in, 2 out]
            n1164 = To Variant(anything=w2553) -> (Variant=w2563:variant)
            n1165 = property on="DAQ Config" class="Arr (strict)"(error in=w2552, "Val(Sgnl)"=w2553) -> (error out=w2560:errorcluster)  [unwired: 1 in, 1 out]
            n1166 = Bundle By Name(cluster=w2558, "Data"=w2563) -> (w2557:T43)
            n1167 = Bundle By Name(cluster=w2562, "HandledMessage"=w2557) -> (w2561:T44)
            n1168 = call <vilib>:"Add State(s) to Queue__jki_lib_state_machine.vi"("State(s) in (\"\")"=w2566) -> ("States Out"=w2565:string)  [unwired: 14 in]
          }
        }
        n1169 = call <userlib>:"State History.vi"("Current State"=w8) -> ("History"=→"State History":string)  [unwired: 6 in]
      }
    }
    frame Enabled {
    }
  }
